vi "COD主界面（列队使用）.vi"() -> (8 "多列列表框":i32(listbox))   [LabVIEW 2016, in "斯坦道CODMn.lvlib"]
uses:
  <vilib>/Analysis/6fits.llb/Curve Fitting Criteria.ctl
  <vilib>/Utility/miscctls.llb/LVPointTypeDef.ctl
  <vilib>/Utility/config.llb/Read Key (I32).vi
  <vilib>/Utility/config.llb/Read Key (Double).vi
  <vilib>/Utility/config.llb/Read Key (Boolean).vi
  <vilib>/Utility/config.llb/Write Key (Double).vi
  <vilib>/Utility/config.llb/Write Key (Boolean).vi
  <vilib>/Utility/config.llb/Write Key (I32).vi
  <vilib>/Waveform/WDTFileIO.llb/Read Waveform from File.vi
  <vilib>/ptbypt/NI_PtbyPt.lvlib
  <vilib>/Utility/config.llb/NI_LVConfig.lvlib
  <vilib>/Analysis/NI_AALPro.lvlib
panel:
  in  "标样核查量程选择":enum32{"H", "L", "AUTO"}(ring)=enum."AUTO"
  in  "标样浓度":dbl
  in  "零点核查量程选择":enum32{"H", "L", "AUTO"}(ring)=enum."AUTO"
  in  "零点核查浓度":dbl
  out "序列号":string
  in  "采水泵排液时间/s:":i32
  in  "采水泵润洗时间/s:":i32
  in  "采水泵沉淀时间/s:":i32
  in  "采水泵进样时间/s:":i32
  in  "常规版/认证版":enum16{"常规版", "认证版", "浮台版"}(ring)
  in  "释放串口":bool
  in  "打开串口":bool
  in  "保存参数":dbl[](array[numeric])
  out "报警数字":i16
  out "CODMn工作状态":T1(ring)
  out "ORP-K":string
  out "ORP-B":string
  out "ORP-A":string
  out "x = y?":bool
  out "稀释倍数解释":string
  in  "跨度量程选择":enum32{"H", "L", "AUTO"}(ring)=enum."AUTO"
  in  "跨度液浓度":dbl
  in  "水样":dbl
  in  "蒸馏水":dbl
  in  "标液":dbl
  in  "质控样":dbl
  in  "加标回收":dbl
  in  "草酸钠":dbl
  in  "高锰酸钾":dbl
  in  "硫酸":dbl
  out "量程解释说明":string
  in  "高切低阈值:":dbl
  in  "低切高阈值:":dbl
  in  "自动切换量程:":enum16{"关闭", "自动切换测一次", "自动切换测两次"}(ring)
  in  "修正系数":dbl
  in  "标准液浓度":dbl
  in  "温度":dbl
  in  "恒温时间":dbl
  in  "基本量程":enum16{"L", "H"}(ring)
  in  "CODMn零点核查选择":enum16{"零点核查走纯水管", "零点核查走质控管"}(ring)
  in  "锁定按钮":bool
  in  "低量程稀释倍数:":i8=1
  out "切换量程连续测两次":bool
  in  "高量程稀释倍数:":i8=2
  in  "一键写入":bool
  in  "测量模式(公式)":u16(ring)=1 items=["水样测试"=1, "标样核查"=2, "零点核查"=3, "跨度核查"=4, "空白测试"=5, "平行样"=6, "加标回收"=7]
  out "基本量程(显示)":string
  out "测量模式(显示)":string
  in  "量程切换次数":u8
  out "数据时间":string
  out "断电排液标记":bool
  out "COM":string
  in  "启用5":bool
  in  "校准5":bool
  in  "泵滴定数5":dbl
  in  "浓度5":dbl
  in  "启用4":bool
  in  "校准4":bool
  in  "泵滴定数4":dbl
  in  "浓度4":dbl
  out "波形时间":timestamp
  in  "历史波形":bool
  out "滴定数-ORP值":u16[](array[numeric]) caption="数组"
  in  "关闭 3":bool
  in  "滴定曲线":bool
  out "ORP滴定曲线":u16[](graph)
  out "空白测试标记":bool
  out "跨度核查标记":bool
  out "启动选择 2":u16(ring) items=["水样测试", "标样核查", "零点核查", "跨度核查", "空白测试", "加标回收", "平行样", "校零", "校标"]
  in  "量程选择":enum16{"低量程", "高量程", "0-2量程"}(ring)
  in  "手动控制":bool
  in  "选用水样":enum16{"葡萄糖", "草酸钠"}(ring)
  in  "方程系数":cluster{"K":dbl, "b":dbl, "X^2":dbl} {"X^2" format="%#.6g"; "b" format="%#.6g"; "K" format="%#.6g"}
  out "多项式系数":dbl[](array[numeric])
  out "XY图":cluster{"X Values":dbl[], "Y Values":dbl[]}[](graph)
  in  "模型":enum32{"线性", "多项式"}(ring)
  out "启动时间":timestamp format="%<%Y/%m/%d %H:%M:%S>T"
  in  "关闭 2":bool
  out "r^2":dbl format="%.8g"
  out "拟合公式":string
  out "b":dbl format="%#.4g"
  out "K":dbl format="%#.4f"
  out "当前校准":i32
  in  "启用3":bool
  in  "启用2":bool
  in  "启用1":bool
  in  "校准3":bool
  in  "校准2":bool
  in  "校准1":bool
  in  "泵滴定数3":dbl
  in  "泵滴定数2":dbl
  in  "泵滴定数1":dbl
  in  "浓度3":dbl
  in  "浓度2":dbl
  in  "浓度1":dbl
  in  "写入":bool
  out "测量模式数字":i32
  out "零点核查标记":bool
  out "排液故障":bool
  out "进水样超量程":bool
  out "标样核查标记":bool
  out "平行样测量":bool
  out "加标回收测量":bool
  out "质控样测量":bool
  out "待机":bool
  out "校标错误":bool
  out "校零错误":bool
  out "测量错误":bool
  out "草酸钠报警":bool
  out "高锰酸钾报警":bool
  out "加热故障":bool
  out "温控器故障":bool
  out "ORP故障":bool
  out "排液标记":bool
  out "故障标记":bool
  out "校标标记":bool
  out "校零标记":bool
  out "通讯状态":bool
  out "水样测量":bool
  in  "读取":bool
  in  "返回":bool
  in  "校准配置":bool
  in  "零点泵计量数 2":dbl
  in  "标度泵计量数 2":dbl
  out "标度滴定值":dbl
  out "零点滴定值":dbl
  in  "保存":bool
  in  "关闭":bool
  out "测量数据区":T2 {"单位" items=["ug/L", "mg/L", "ppm", "mg/m3", "cm", "ppb", "ug/m3", "%", "nmol/mol", "umol/mol", "MPN/L", "MPN/100ml", "ng/m3", "NTU", "无量纲", "ms/cm", "us/cm", "℃", "mV", "万个/L"]}
  out "仪器时间":timestamp format="%<%Y/%m/%d %H:%M:%S>T"
  out "秒":u16
  out "分":u16
  out "COD浓度（mg/L)":dbl format="%.2g"
  out "进样管":dbl
  out "高锰酸钾":dbl
  out "草酸钠":dbl
  out "硫酸":dbl
  out "ORP显示":dbl
  out "温度":dbl
  out "加热":bool
  out "搅拌":bool
  out "进硫酸":bool
  out "进加标回收样":bool
  out "进质控样":bool
  out "进标液":bool
  out "进蒸馏水":bool
  out "进水样":bool
  out "进草酸钠":bool
  out "进高锰酸钾":bool
  out "定时启动":bool
  in  "启动":bool
  in  "故障清除":bool
  in  "参数配置":bool
  in  "停止":bool
  in  "单步启动":bool
  out "系统时间":timestamp
  in  "时间校准":bool
  out "报警簇":T3
  out "模式（受控）":u16
  # "测量时间："
  # "(水样~加标回收)"
  # "mV"
  # "℃"
  # "注：遇到加热故障和排液故障时仪器不能正常启动，\n必须排查故障并点击报警清除按钮方可运行。"
  # "mg/L"
  # "基本参数设置"
  # "校零校标结果"
  # "泵计量参数设置"
  # "校零结果："
  # "校零滴定值："
  # "加热恒温温度(℃):"
  # "水样："
  # "高锰酸钾："
  # "校标结果："
  # "标度滴定值："
  # "恒温时间(分钟):"
  # "草酸钠："
  # "蒸馏水："
  # "零点泵计量值："
  # "标准液浓度(mg/L):"
  # "硫酸："
  # "标液："
  # "标度泵计量值："
  # "修正系数："
  # "跨度核查浓度："
  # "质控样:"
  # "基本量程(L、H)可选:"
  # "跨度量程选择："
  # "加标回收样："
  # "零点核查浓度："
  # "标样浓度："
  # "零点量程选择："
  # "标样量程选择："
  # "是否启用"
  # "泵滴定数"
  # "浓度"
  # "辅\n助\n计\n算\n区"
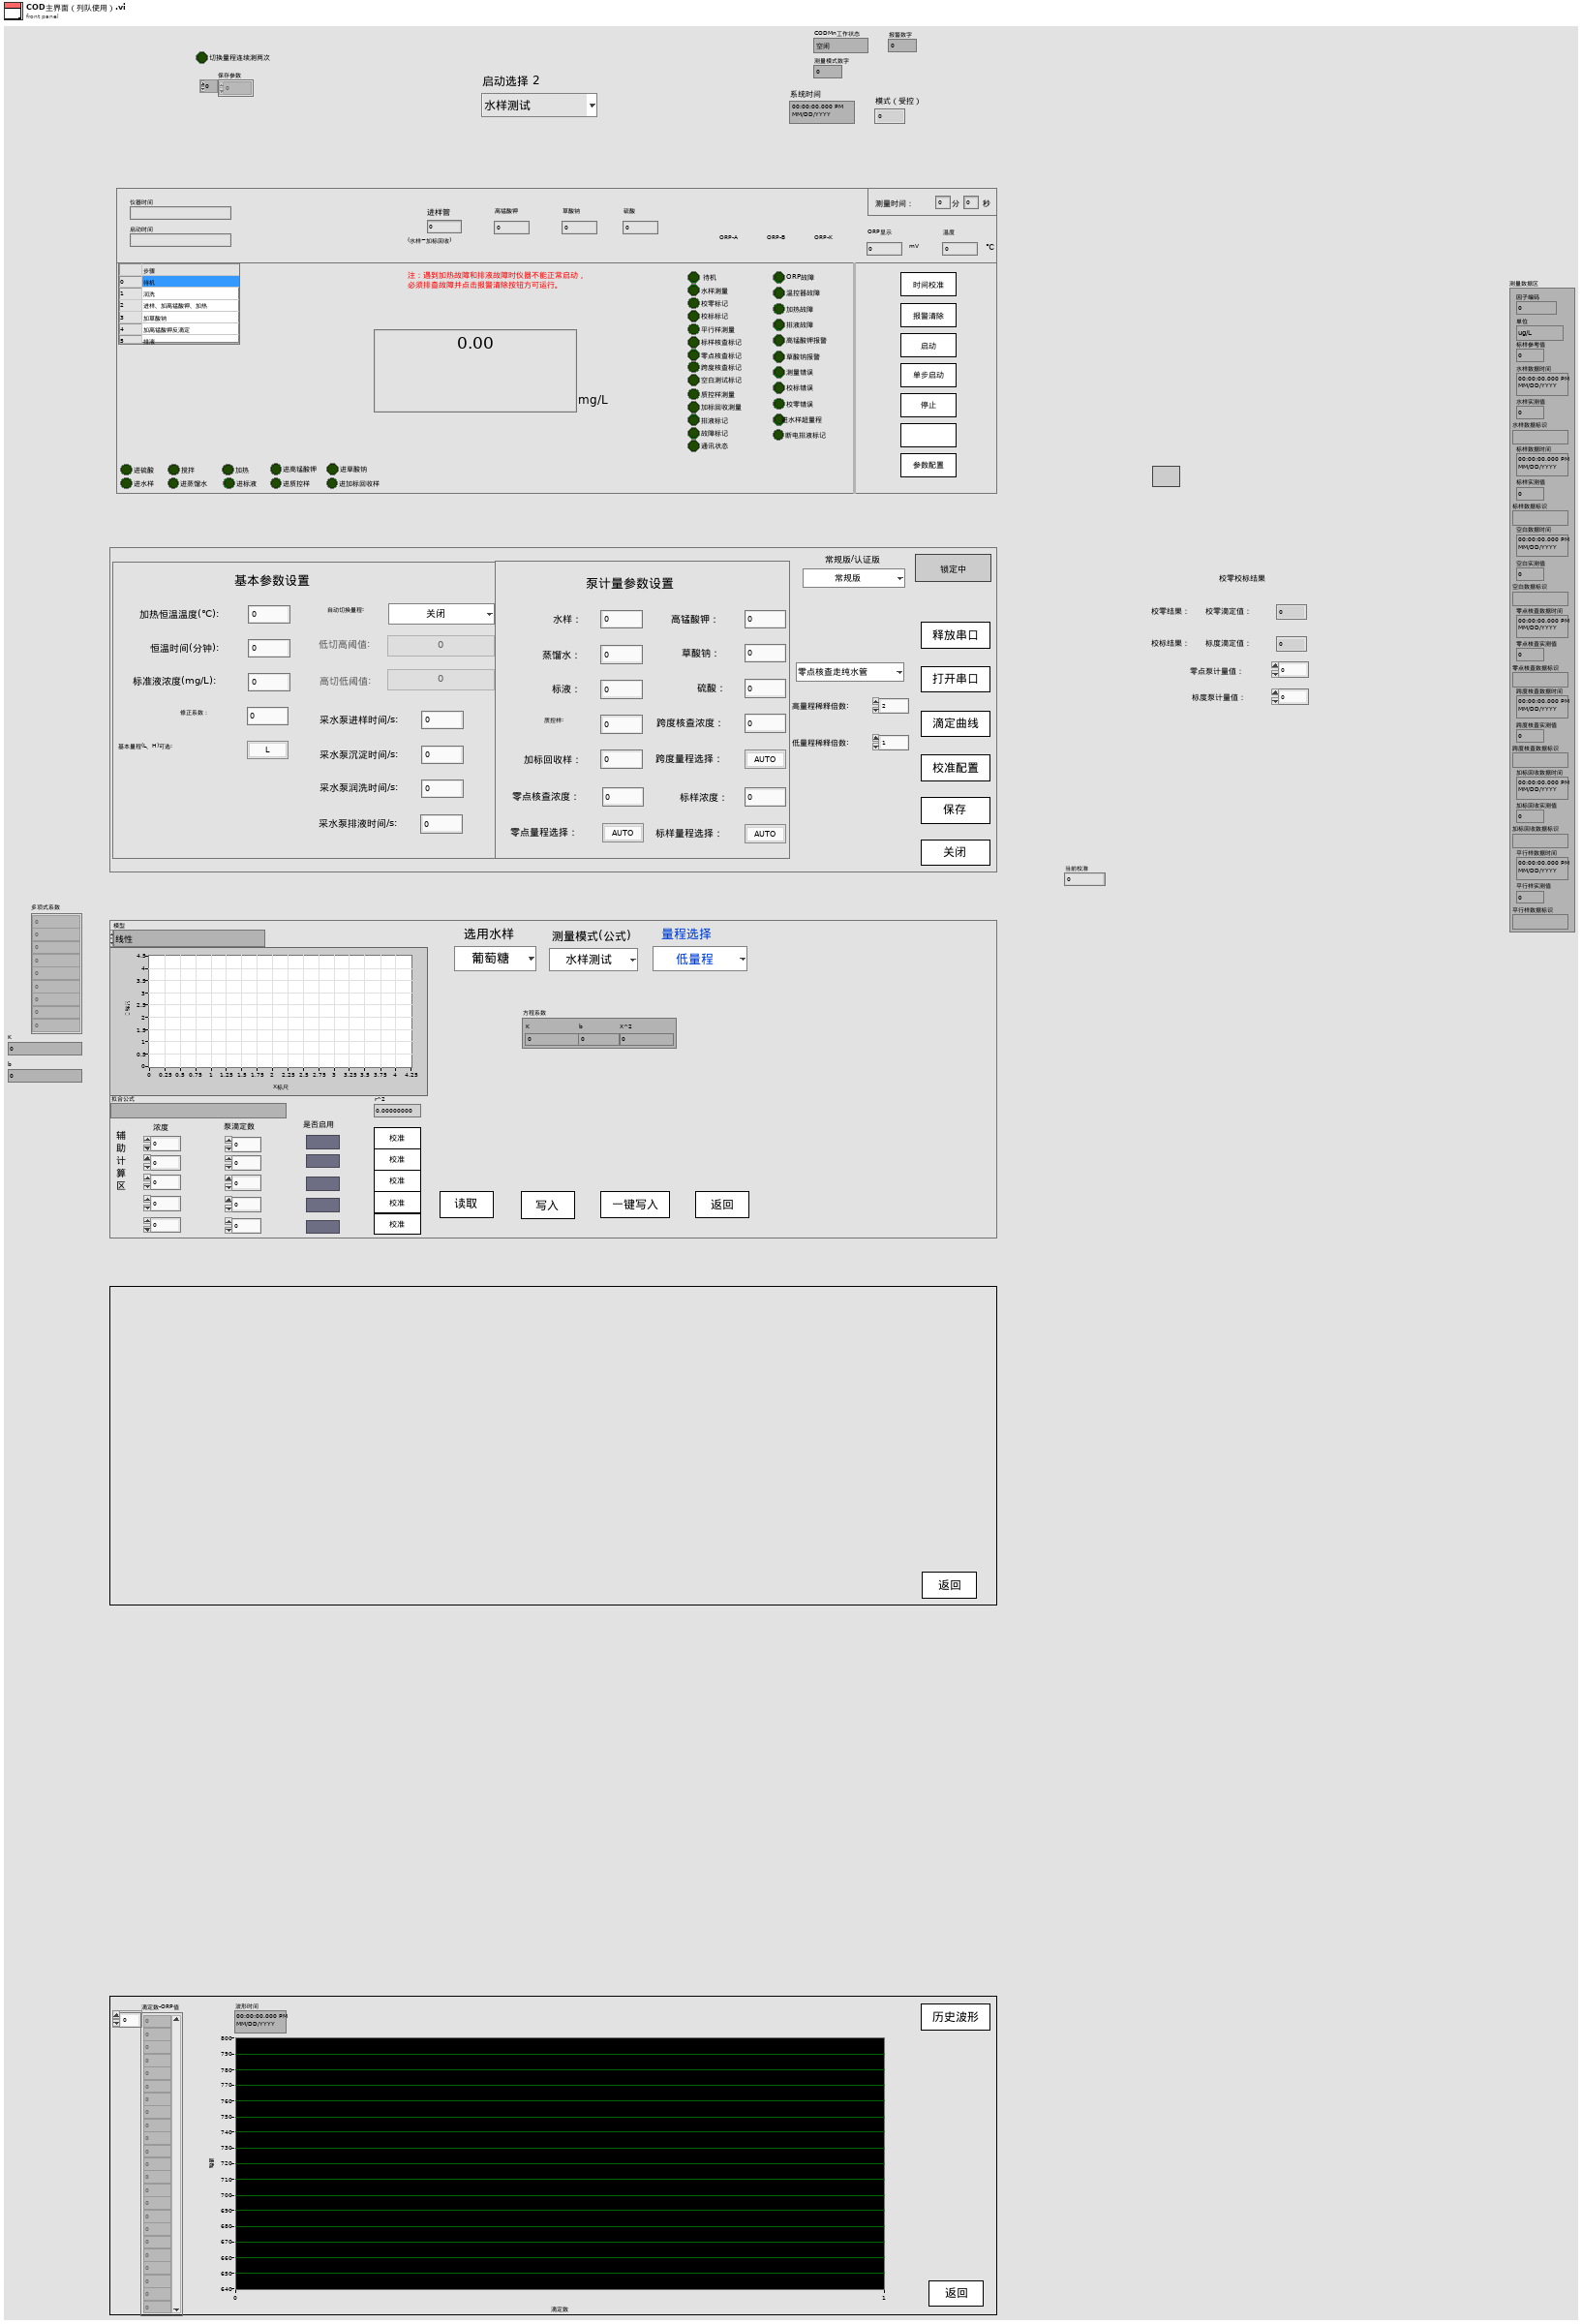
[diagram p1: front panel]
types:
  T1 = enum16{"空闲", "水样测试", "标样核查", "零点核查", "跨度核查", "空白测试", "平行样测试", "质控样", "空白校准", "标样校准", "加标回收"}
  T2 = cluster{"因子编码":u32, "单位":u16, "标样参考值":sgl, "水样数据时间":timestamp, "水样实测值":sgl, "水样数据标识":string, "标样数据时间":timestamp, "标样实测值":sgl, "标样数据标识":string, "空白数据时间":timestamp, "空白实测值":sgl, "空白数据标识":string, "零点核查数据时间":timestamp, "零点核查实测值":sgl, "零点核查数据标识":string, "跨度核查数据时间":timestamp, "跨度核查实测值":sgl, "跨度核查数据标识":string, "加标回收数据时间":timestamp, "加标回收实测值":sgl, "加标回收数据标识":string, "平行样数据时间":timestamp, "平行样实测值":sgl, "平行样数据标识":string}
  T3 = cluster{"ORP故障":bool, "温控器故障":bool, "加热故障":bool, "高锰酸钾报警":bool, "草酸钠报警":bool, "测量错误":bool, "校零错误":bool, "校标错误":bool, " 进水样超量程":bool, "排液阀故障":bool}
  T4 = cluster{"命令":string, "测量模式":enum16{"水样测量", "标样核查", "零点核查", "跨度核查", "空白测试", "加标回收", "平行样", "校零", "校标"}, "CODMn量程切换":enum32{"H", "L", "AUTO"}}
  T5 = cluster{"时间":timestamp, "测量模式":string, "数据类型":string, "检测值":sgl, "单位":string, "数据标识":string, "因子编码":string, "标样参考值":sgl, "ORP-A":sgl, "ORP-B":sgl, "ORP-K":sgl, "COD滴定值":sgl, "高锰酸钾滴定数":sgl, "温度":sgl, "序列号":string, "量程":sgl, "LastTime":timestamp}
  T6 = enum8{"Enabled", "Disabled", "Disabled and Grayed Out"}
  T7 = cluster{"数组 2[0]":sgl, "数组 2[1]":sgl, "数组 2[2]":sgl, "数组 2[3]":sgl, "数组 2[4]":sgl, "数组 2[5]":sgl, "数组 2[6]":sgl, "数组 2[7]":sgl, "数组 2[8]":sgl, "数组 2[9]":sgl, "数组 2[10]":sgl, "数组 2[11]":sgl, "数组 2[12]":sgl, "数组 2[13]":sgl, "数组 2[14]":sgl, "数组 2[15]":sgl, "数组 2[16]":sgl, "数组 2[17]":sgl, "数组 2[18]":sgl, "数组 2[19]":sgl, "数组 2[20]":sgl, "数组 2[21]":sgl, "数组 2[22]":sgl, "数组 2[23]":sgl, "数组 2[24]":sgl, "数组 2[25]":sgl, "数组 2[26]":sgl, "数组 2[27]":sgl, "数组 2[28]":sgl, "数组 2[29]":sgl, "数组 2[30]":sgl, "数组 2[31]":sgl, "数组 2[32]":sgl, "数组 2[33]":sgl, "数组 2[34]":sgl, "数组 2[35]":sgl, "数组 2[36]":sgl, "数组 2[37]":sgl, "数组 2[38]":sgl, "数组 2[39]":sgl, "数组 2[40]":sgl, "数组 2[41]":sgl}
  T8 = typedef "NI_AALPro.lvlib/Curve Fitting Criteria.ctl" = u16
  T9 = cluster{"测量模式":enum16{"水样测量", "标样核查", "零点核查", "跨度核查", "空白测试", "加标回收", "平行样", "校零", "校标"}}
  T10 = cluster{"仪器测试类型":enum16{"水样测试", "零点核查", "标样核查", "空白测试", "跨度核查", "加标回收", "平行样", "校零", "校标"}, "周期设置类型":enum16{"定点启动", "间隔启动"}, "定时功能启用":bool, "定时间隔":dbl, "24H周期设置":bool[]}
  T11 = typedef "LVDateTimeRec.ctl" = cluster{"秒数的小数部分":dbl, "秒":i32, "分":i32, "时":i32, "日":i32, "月":i32, "年":i32, "天数（周）":i32, "天数（年）":i32, "DST":i32}
  T12 = enum16{"水样测试", "零点核查", "标样核查", "空白测试", "跨度核查", "加标回收", "平行样", "校零", "校标"}
  T13 = cluster{"时间标识":timestamp, "设备":string, "日志信息":string}
  T14 = cluster{"时间标识":timestamp, "参数":string, "日志信息":string, "流程参数":string}
  T15 = cluster{"时间标识":timestamp, "设备":string, "日志信息":string, "流程参数":string}
  T16 = typedef "NI_LVConfig.lvlib/Config Data RefNum.ctl" = refnum<k1>
  T17 = typedef "LVPointTypeDef.ctl" = cluster{"Horizontal":i16, "Vertical":i16}
  T18 = enum16{"水样测量", "标样核查", "零点核查", "跨度核查", "空白测试", "加标回收", "平行样", "校零", "校标"}
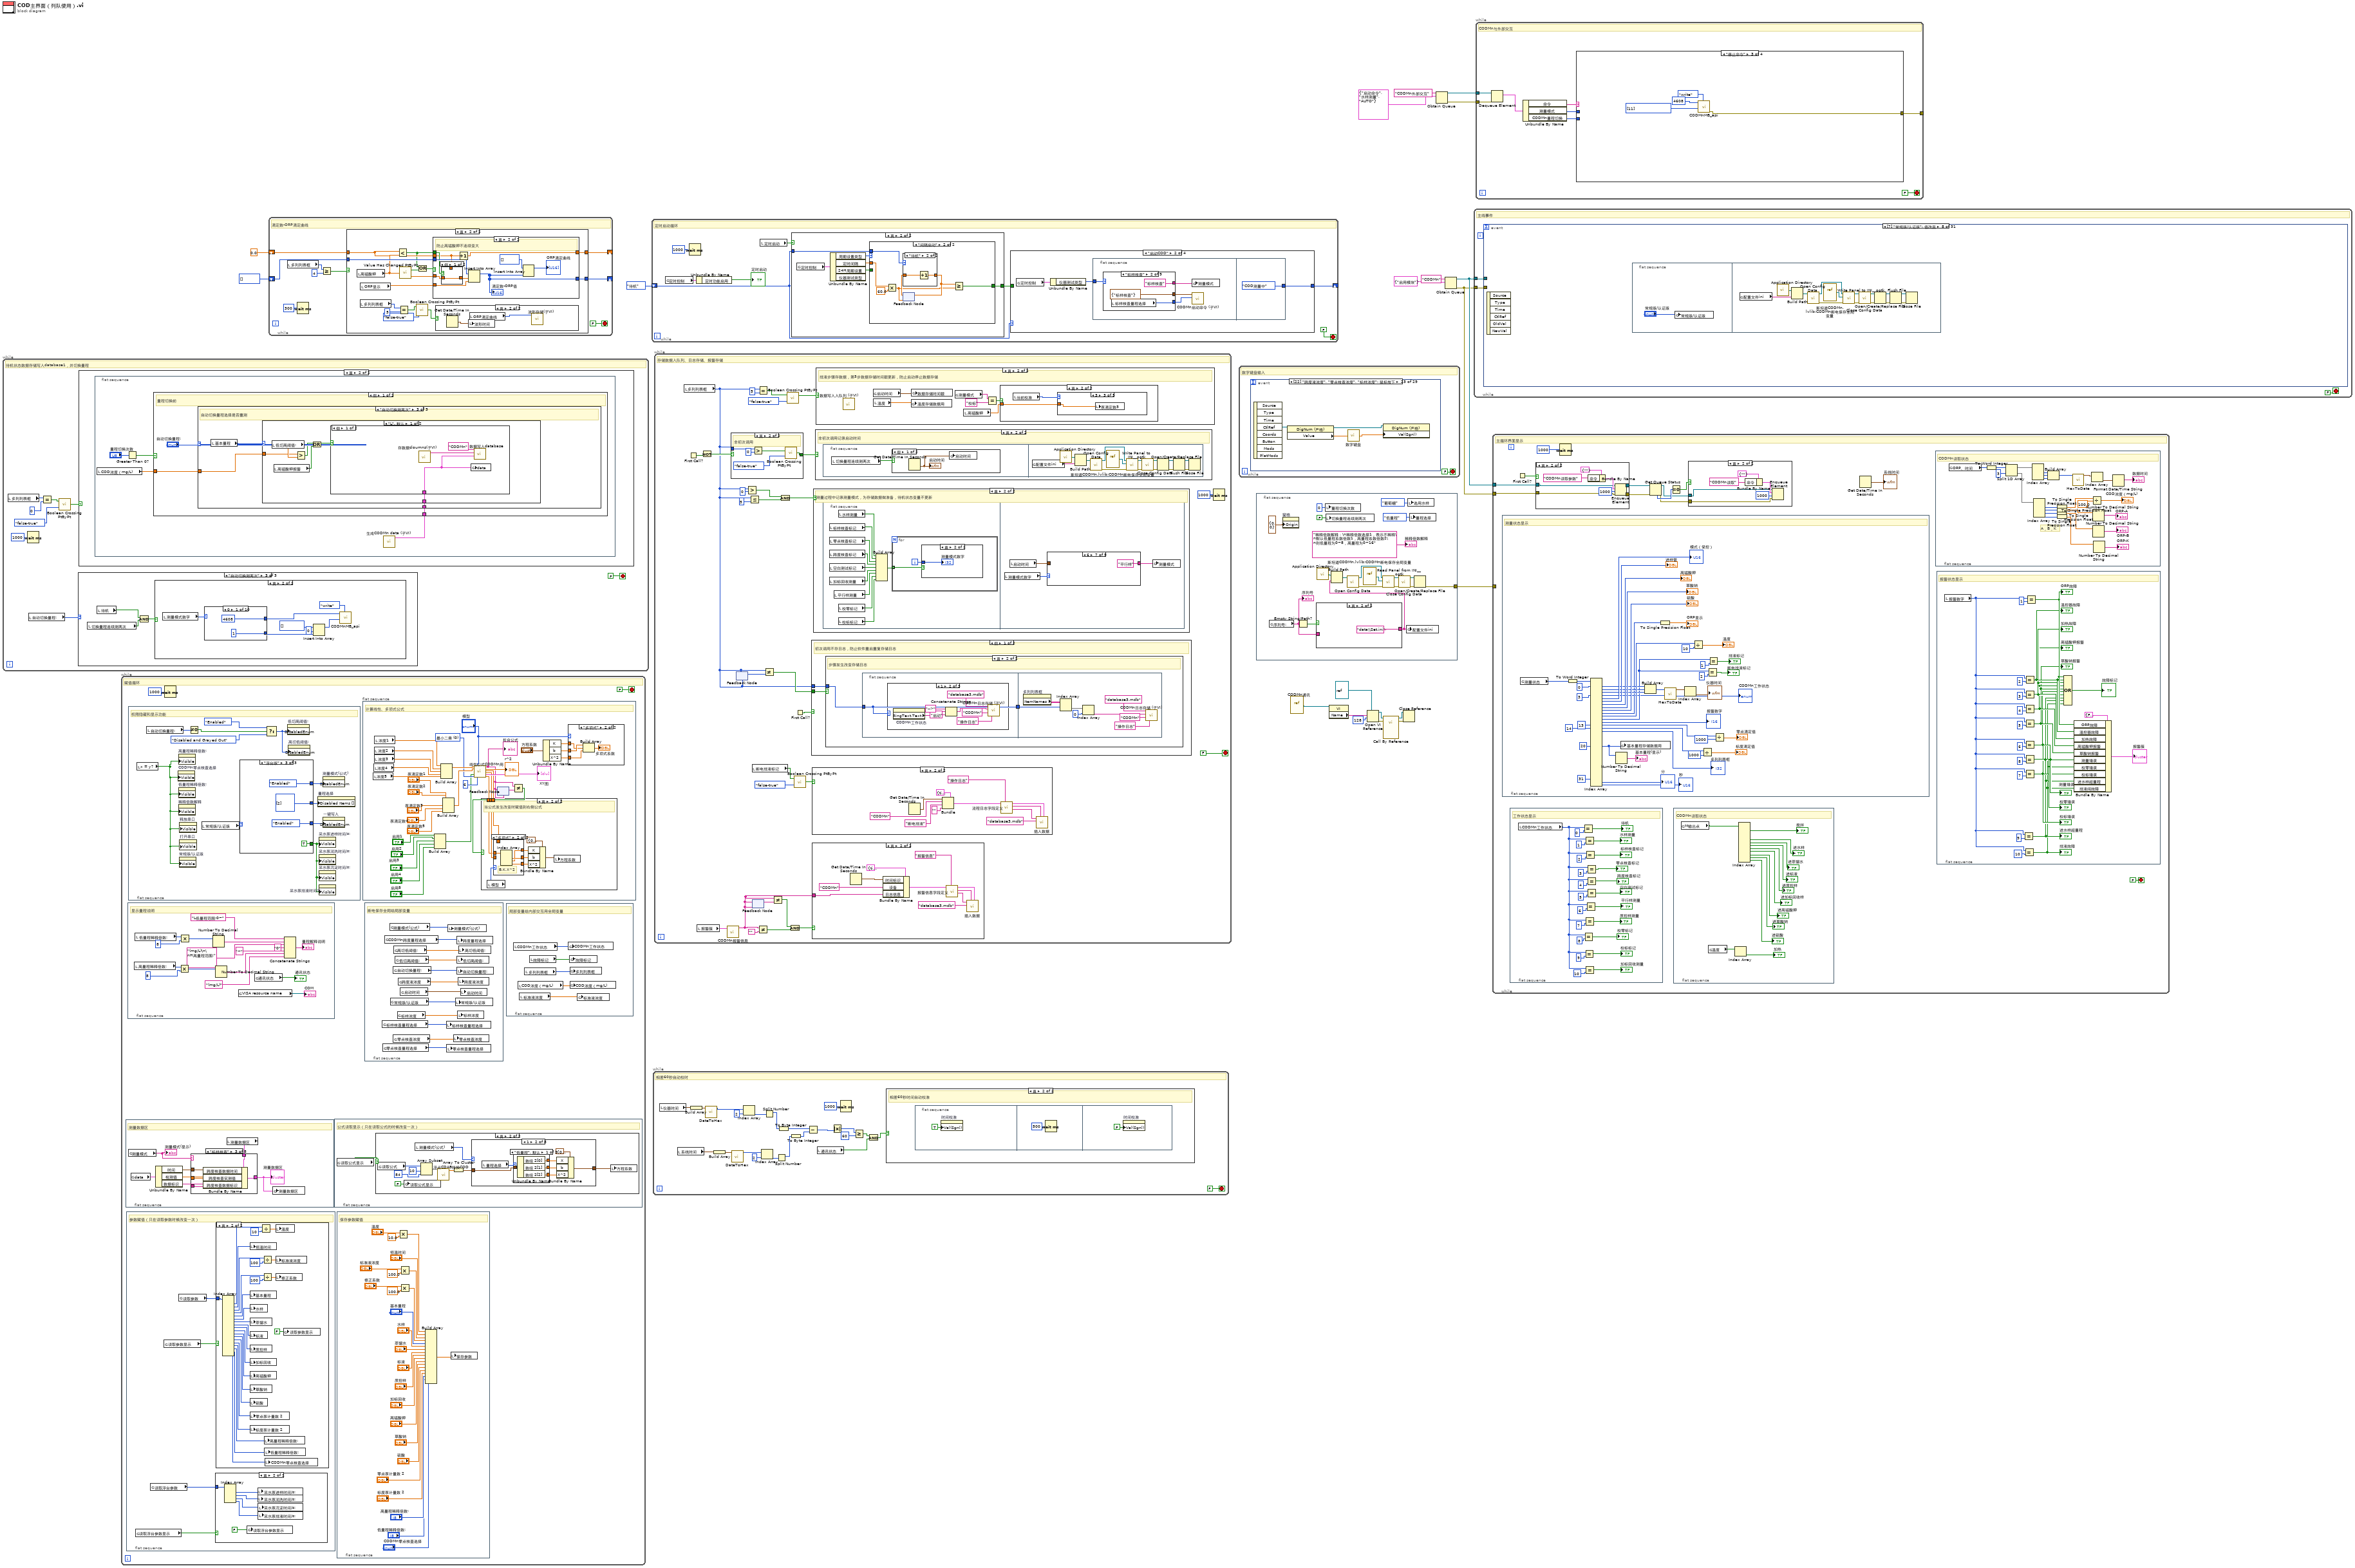
[diagram p0: block diagram]
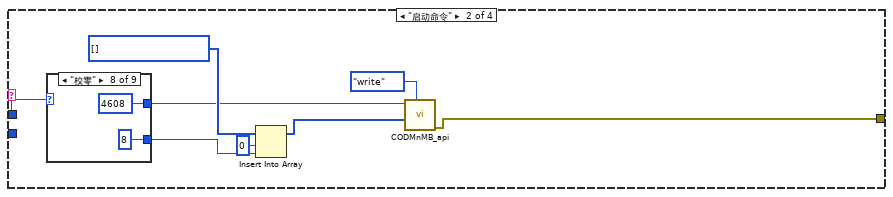
[diagram p3: hidden frame]
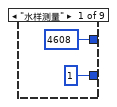
[diagram p4: hidden frame]
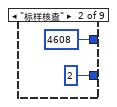
[diagram p5: hidden frame]
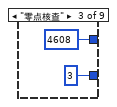
[diagram p6: hidden frame]
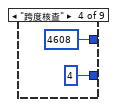
[diagram p7: hidden frame]
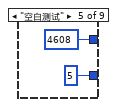
[diagram p8: hidden frame]
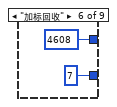
[diagram p9: hidden frame]
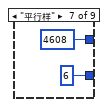
[diagram p10: hidden frame]
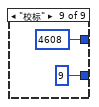
[diagram p11: hidden frame]
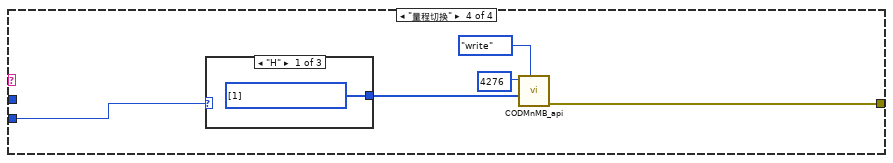
[diagram p12: hidden frame]
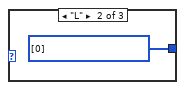
[diagram p13: hidden frame]
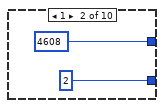
[diagram p19: hidden frame]
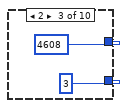
[diagram p20: hidden frame]
diagram:
  n1 = while {
    stop <- FALSE stop-if-true
    # "待机状态数据存储写入database1，并切换量程"
    n2 = local read "多列列表框"() -> (w26:i32)
    n3 = Wait (ms)(milliseconds to wait=u32 1000 ("等待时间（毫秒）")) -> ()  [unwired: 1 out]
    n4 = local read "自动切换量程:"() -> (w21:enum16{"关闭", "自动切换测一次", "自动切换测两次"})
    n5 = Equal?(x=w26, y=0) -> (x = y?=w24:bool)
    n6 = call <vilib>:"Boolean Crossing PtByPt.vi"("direction"=enum16{"either", "false-true", "true-false"}."false-true", "input"=w24) -> ("crossing"=w22:bool)  [unwired: 1 in]
    n7 = case shown="\"自动切换测两次\"" w21 {
      frame "关闭", Default {
      }
      frame "自动切换测一次" {
      }
      frame "自动切换测两次" {
        n8 = local read "切换量程连续测两次"() -> (w30:bool)
        n9 = local read "待机"() -> (w31:bool)
        n10 = Compound Arithmetic op=AND ("复合运算")(w31, w30) -> (w29:bool)
        n11 = case shown="真" w29 {
          frame False {
          }
          frame True {
            n12 = local read "测量模式数字"() -> (w35:i32)
            n13 = case shown="0" w35 {
              tunnel: [u16 4608 ("address") u16 4608 ("address") u16 4608 ("address") u16 4608 ("address") u16 4608 ("address") u16 4608 ("address") u16 4608 ("address") u16 4608 ("address") u16 4608 ("address") u16 4608 ("address")] -> w32
              tunnel: [u16 1 ("address") u16 2 ("address") u16 3 ("address") u16 4 ("address") u16 5 ("address") u16 7 ("address") u16 6 ("address") u16 8 ("address") u16 9 ("address") u16 0 ("address")] -> w38
              frame 0 {
              }
              frame 1 {
              }
              frame 2 {
              }
              frame 3 {
              }
              frame 4 {
              }
              frame 5 {
              }
              frame 6 {
              }
              frame 7 {
              }
              frame 8 {
              }
              frame 9, Default {
              }
            }
            n14 = Insert Into Array(array=u16[] [] ("values"), index=0 ("索引"), new element=w38) -> (w33:u16[])
            n15 = call "CODMnMB_api.vi"("STEP"=enum16{"open", "read", "write", "close"}."write", "values"=w33, "starting address"=w32) -> ()  [unwired: 5 in, 4 out]
          }
        }
      }
    }
    n16 = case shown="真" w22 {
      frame False {
      }
      frame True {
        n17 = flat-sequence {
          frame #0 {
            n18 = local read "COD浓度（mg/L)"() -> (w59:dbl)
            n19 = Greater Than 0?(x="量程切换次数") -> (x > 0?=w60:bool)
            n20 = call "生成CODMn data (子VI).vi"() -> ("data"=w62:T5)  [unwired: 11 in]
            n21 = case shown="假" w60 {
              tunnel: w62 -> [w64 w121]
              tunnel: w59 -> [w63 _]
              frame False {
                # "量程切换前"
                n22 = case shown="\"自动切换测两次\"" "自动切换量程:" {
                  tunnel: w64 -> [w66 w71 w95]
                  tunnel: w63 -> [_ w70 w94]
                  frame "关闭", Default {
                    # "关闭自动切换量程"
                    n23 = call "存数据cloumns(子VI).vi"() -> ("数组"=w68:string[])  [unwired: 11 in]
                    n24 = global write "COD读取DATA全局.vi" "data"(w66) -> ()
                    n25 = call "数据写入database.vi"("data"=w66, "columns"=w68, "table"="CODMn") -> ()  [unwired: 8 in, 1 out]
                  }
                  frame "自动切换测一次" {
                    # "自动切换量程选择是否重测"
                    n26 = global read "COD测量模式全局.vi" "测量模式"() -> (w77:string)
                    n27 = Not Equal?(x=w77, y="水样测试") -> (x != y?=w75:bool)
                    n28 = case shown="假" w75 {
                      tunnel: [w78 w79] -> w74
                      tunnel: w70 -> [w78 _]
                      frame False {
                      }
                      frame True {
                        n29 = global read "COD读取DATA全局.vi" "测量数据区"() -> (w80:T2)
                        n30 = Unbundle By Name(w80) -> ("水样实测值"=w79:sgl)
                      }
                    }
                    n31 = local read "基本量程"() -> (w69:enum16{"L", "H"})
                    n32 = case shown="\"H\"" w69 {
                      tunnel: w74 -> [w81 w87]
                      frame "L", Default {
                        n33 = Greater?(x=w81, y="低切高阈值:") -> (0:w82:bool)
                        n34 = case shown="假" w82 {
                          frame False {
                          }
                          frame True {
                            n35 = call "CODMnMB_api.vi"("STEP"=enum16{"open", "read", "write", "close"}."write", "values"=u16[] [1], "starting address"=u16 4276) -> ()  [unwired: 5 in, 4 out]
                          }
                        }
                      }
                      frame "H" {
                        n36 = Less?(x=w87, y="高切低阈值:") -> (x < y?=w88:bool)
                        n37 = case shown="真" w88 {
                          frame False {
                          }
                          frame True {
                            n38 = call "CODMnMB_api.vi"("STEP"=enum16{"open", "read", "write", "close"}."write", "values"=u16[] [0], "starting address"=u16 4276) -> ()  [unwired: 5 in, 4 out]
                          }
                        }
                      }
                    }
                    n39 = call "存数据cloumns(子VI).vi"() -> ("数组"=w73:string[])  [unwired: 11 in]
                    n40 = global write "COD读取DATA全局.vi" "data"(w71) -> ()
                    n41 = call "数据写入database.vi"("data"=w71, "columns"=w73, "table"="CODMn") -> ()  [unwired: 8 in, 1 out]
                  }
                  frame "自动切换测两次" {
                    # "自动切换量程选择是否重测"
                    n42 = local read "基本量程"() -> (w93:enum16{"L", "H"})
                    n43 = case shown="\"L\", 默认" w93 {
                      tunnel: w94 -> [w99 w110]
                      tunnel: w95 -> [w98 w109]
                      frame "L", Default {
                        n44 = local read "低切高阈值:"() -> (w100:dbl)
                        n45 = local read "高锰酸钾报警"() -> (w96:bool)
                        n46 = Greater?(x=w99, y=w100) -> (0:w101:bool)
                        n47 = Or(x=w101, y=w96) -> (x .or. y?=w97:bool)
                        n48 = case shown="假" w97 {
                          tunnel: w98 -> [w102 _]
                          frame False {
                            n49 = call "存数据cloumns(子VI).vi"() -> ("数组"=w104:string[])  [unwired: 11 in]
                            n50 = global write "COD读取DATA全局.vi" "data"(w102) -> ()
                            n51 = call "数据写入database.vi"("data"=w102, "columns"=w104, "table"="CODMn") -> ()  [unwired: 8 in, 1 out]
                          }
                          frame True {
                            n52 = call "CODMnMB_api.vi"("STEP"=enum16{"open", "read", "write", "close"}."write", "values"=u16[] [1], "starting address"=u16 4276) -> ()  [unwired: 5 in, 4 out]
                            "切换量程连续测两次" <- TRUE ("切换量程连续测两次")
                          }
                        }
                      }
                      frame "H" {
                        n53 = local read "高切低阈值:"() -> (w111:dbl)
                        n54 = Less?(x=w110, y=w111) -> (x < y?=w112:bool)
                        n55 = case shown="真" w112 {
                          tunnel: w109 -> [w113 _]
                          frame False {
                            n56 = call "存数据cloumns(子VI).vi"() -> ("数组"=w115:string[])  [unwired: 11 in]
                            n57 = global write "COD读取DATA全局.vi" "data"(w113) -> ()
                            n58 = call "数据写入database.vi"("data"=w113, "columns"=w115, "table"="CODMn") -> ()  [unwired: 8 in, 1 out]
                          }
                          frame True {
                            # "重测第一次不存数据"
                            n59 = call "CODMnMB_api.vi"("STEP"=enum16{"open", "read", "write", "close"}."write", "values"=u16[] [0], "starting address"=u16 4276) -> ()  [unwired: 5 in, 4 out]
                            n60 = local write "切换量程连续测两次"(TRUE ("切换量程连续测两次")) -> ()
                          }
                        }
                      }
                    }
                  }
                }
              }
              frame True {
                # "防止无限切量程"
                n61 = local write "量程切换次数"(u8 0 ("量程切换次数")) -> ()
                n62 = call "存数据cloumns(子VI).vi"() -> ("数组"=w123:string[])  [unwired: 11 in]
                n63 = call "数据写入database.vi"("data"=w121, "columns"=w123, "table"="CODMn") -> ()  [unwired: 8 in, 1 out]
                n64 = global write "COD读取DATA全局.vi" "data"(w121) -> ()
              }
            }
          }
        }
      }
    }
  }
  n65 = while {
    stop <- FALSE stop-if-true
    # "赋值循环"
    n66 = flat-sequence {
      frame #0 {
        # "测量数据区"
        n67 = global read "COD测量模式全局.vi" "测量模式"() -> (w391:string)
        "测量模式(显示)" <- w391
        n68 = global read "COD读取DATA全局.vi" "data"() -> (w396:T5)
        n69 = Unbundle By Name(w396) -> ("时间"=w395:timestamp, "检测值"=w394:sgl, "数据标识"=w393:string)
        n70 = local read "测量数据区"() -> (w397:T2)
        n71 = case shown="\"标样核查\"" w391 {
          tunnel: w397 -> [w398 w403 w408 w413 w418 w423 w428 w433]
          tunnel: [w398 w402 w404 w412 w417 w422 w424 w432] -> w392
          tunnel: w395 -> [_ w401 w407 w411 w416 w421 w427 w431]
          tunnel: w394 -> [_ w400 w406 w410 w415 w420 w426 w430]
          tunnel: w393 -> [_ w399 w405 w409 w414 w419 w425 w429]
          frame "", Default {
          }
          frame "水样测试" {
            n72 = Bundle By Name(cluster=w403, "水样数据时间"=w401, "水样实测值"=w400, "水样数据标识"=w399) -> (w402:T2)
          }
          frame "标样核查" {
            n73 = Bundle By Name(cluster=w408, "跨度核查数据时间"=w407, "跨度核查实测值"=w406, "跨度核查数据标识"=w405) -> (w404:T2)
          }
          frame "零点核查" {
            n74 = Bundle By Name(cluster=w413, "零点核查数据时间"=w411, "零点核查实测值"=w410, "零点核查数据标识"=w409) -> (w412:T2)
          }
          frame "加标回收" {
            n75 = Bundle By Name(cluster=w418, "加标回收数据时间"=w416, "加标回收实测值"=w415, "加标回收数据标识"=w414) -> (w417:T2)
          }
          frame "平行样" {
            n76 = Bundle By Name(cluster=w423, "平行样数据时间"=w421, "平行样实测值"=w420, "平行样数据标识"=w419) -> (w422:T2)
          }
          frame "校零" {
            n77 = Bundle By Name(cluster=w428, "空白数据时间"=w427, "空白实测值"=w426, "空白数据标识"=w425) -> (w424:T2)
          }
          frame "校标" {
            n78 = Bundle By Name(cluster=w433, "标样数据时间"=w431, "标样实测值"=w430, "标样数据标识"=w429) -> (w432:T2)
          }
        }
        "测量数据区" <- w392
        n79 = global write "COD读取DATA全局.vi" "测量数据区"(w392) -> ()
      }
    }
    n80 = flat-sequence {
      frame #0 {
        # "参数赋值（只在读取参数时候改变一次）"
        n81 = global read "COD读取DATA全局.vi" "读取浮台参数显示"() -> (w157:bool)
        n82 = global read "COD读取DATA全局.vi" "读取浮台参数"() -> (w156:u16[])
        n83 = global read "COD读取DATA全局.vi" "读取参数显示"() -> (w158:bool)
        n84 = global read "COD读取DATA全局.vi" "读取参数"() -> (w159:u16[])
        n85 = case shown="真" w157 {
          tunnel: w156 -> [_ w165]
          frame False {
          }
          frame True {
            n86 = Index Array(array=w165) -> (element #1=w164:u16, element #2=w163:u16, element #3=w162:u16, element #4=w161:u16)  [unwired: 4 in]
            n87 = global write "COD读取DATA全局.vi" "读取浮台参数显示"(FALSE ("读取参数显示")) -> ()
            n88 = local write "采水泵进样时间/s:"(w164) -> ()
            n89 = local write "采水泵润洗时间/s:"(w163) -> ()
            n90 = local write "采水泵沉淀时间/s:"(w162) -> ()
            n91 = local write "采水泵排液时间/s:"(w161) -> ()
          }
        }
        n92 = case shown="真" w158 {
          tunnel: w159 -> [_ w167]
          frame False {
          }
          frame True {
            n93 = Index Array(array=w167) -> (element #1=w179:u16, element #2=w191:u16, element #3=w172:u16, element #4=w177:u16, element #5=w175:u16, element #6=w174:u16, element #7=w190:u16, element #8=w189:u16, element #9=w188:u16, element #10=w187:u16, element #11=w186:u16, element #12=w185:u16, element #13=w184:u16, element #14=w183:u16, element #15=w182:u16, element #16=w170:u16, element #17=w169:u16, element #18=w168:u16)  [unwired: 18 in]
            n94 = local write "恒温时间"(w191) -> ()
            n95 = local write "基本量程"(w175) -> ()
            n96 = local write "水样"(w174) -> ()
            n97 = local write "蒸馏水"(w190) -> ()
            n98 = local write "标液"(w189) -> ()
            n99 = local write "质控样"(w188) -> ()
            n100 = local write "加标回收"(w187) -> ()
            n101 = local write "高锰酸钾"(w186) -> ()
            n102 = local write "草酸钠"(w185) -> ()
            n103 = local write "硫酸"(w184) -> ()
            n104 = local write "零点泵计量数 2"(w183) -> ()
            n105 = local write "标度泵计量数 2"(w182) -> ()
            n106 = Divide(x=w179, y=u16 10) -> (x/y=w180:dbl)
            n107 = Divide(x=w172, y=u16 100) -> (x/y=w171:dbl)
            n108 = Divide(x=w177, y=u16 100) -> (x/y=w176:dbl)
            n109 = local write "高量程稀释倍数:"(w170) -> ()
            n110 = local write "低量程稀释倍数:"(w169) -> ()
            n111 = local write "CODMn零点核查选择"(w168) -> ()
            n112 = local write "温度"(w180) -> ()
            n113 = local write "标准液浓度"(w171) -> ()
            n114 = local write "修正系数"(w176) -> ()
            n115 = global write "COD读取DATA全局.vi" "读取参数显示"(FALSE ("读取参数显示")) -> ()
          }
        }
      }
    }
    n116 = flat-sequence {
      frame #0 {
        # "显示量程说明"
        n117 = local read "高量程稀释倍数:"() -> (w449:i8)
        n118 = local read "低量程稀释倍数:"() -> (w459:i8)
        n119 = Multiply(x=w449, y=i8 8) -> (x*y=w447:i8)
        n120 = Multiply(x=w459, y=i8 8) -> (x*y=w451:i8)
        n121 = Number To Decimal String(number=w451) -> (decimal integer string=w456:string)  [unwired: 1 in]
        n122 = Number To Decimal String(number=w447) -> (decimal integer string=w454:string)  [unwired: 1 in]
        n123 = global read "CODMn断电保存全局变量.vi" "VISA resource name"() -> (→"COM":refnum<visa-resource-name>)
        n124 = global read "COD读取DATA全局.vi" "通讯状态"() -> (→"通讯状态":bool)
        n125 = Concatenate Strings("L低量程范围:0~" ("量程解释说明"), w456, "(mg/L)\n\nH高量程范围:" ("量程解释说明"), "0" ("字符串"), "~" ("量程解释说明"), w454, "(mg/L)" ("量程解释说明")) -> (→"量程解释说明":string)
      }
    }
    n126 = flat-sequence {
      frame #0 {
        # "权限隐藏和显示功能"
        n127 = local read "x = y?"() -> (w462:bool)
        n128 = local read "自动切换量程:"() -> (w469:enum16{"关闭", "自动切换测一次", "自动切换测两次"})
        n129 = property on="CODMn零点核查选择" class="Enum (严格)"("Visible"=w462) -> ()  [unwired: 2 in, 2 out]
        n130 = property on="高量程稀释倍数:" class="DigNum (严格)"("Visible"=w462) -> ()  [unwired: 2 in, 2 out]
        n131 = property on="低量程稀释倍数:" class="DigNum (严格)"("Visible"=w462) -> ()  [unwired: 2 in, 2 out]
        n132 = property on="稀释倍数解释" class="Str"("Visible"=w462) -> ()  [unwired: 2 in, 2 out]
        n133 = property on="常规版/认证版" class="Enum (严格)"("Visible"=w462) -> ()  [unwired: 2 in, 2 out]
        n134 = property on="释放串口" class="Bool"("Visible"=w462) -> ()  [unwired: 2 in, 2 out]
        n135 = property on="打开串口" class="Bool"("Visible"=w462) -> ()  [unwired: 2 in, 2 out]
        n136 = Not Equal To 0?(x=w469) -> (x != 0?=w468:bool)
        n137 = local read "常规版/认证版"() -> (w467:enum16{"常规版", "认证版", "浮台版"})
        n138 = case shown="\"浮台版\"" w467 {
          tunnel: [T6."Enabled" ("禁用") T6."Disabled and Grayed Out" ("禁用") T6."Enabled" ("禁用")] -> w466
          tunnel: [i32[] [2] ("禁用项[]") i32[] [] ("禁用项[]") i32[] [2] ("禁用项[]")] -> w465
          tunnel: [T6."Enabled" ("禁用") T6."Disabled and Grayed Out" ("禁用") T6."Enabled" ("禁用")] -> w464
          tunnel: [FALSE FALSE TRUE] -> w463
          frame "常规版", Default {
          }
          frame "认证版" {
            w478 = u16 1 items=["水样测试"=1, "标样核查"=2, "零点核查"=3, "跨度核查"=4, "空白测试"=5, "平行样"=6, "加标回收"=7] ("测量模式(公式)")
            n139 = global write "CODMn断电保存全局变量.vi" "测量模式(公式)"(w478) -> ()
          }
          frame "浮台版" {
          }
        }
        n140 = Select(t=T6."Enabled" ("禁用"), s=w468, f=T6."Disabled and Grayed Out" ("禁用")) -> (s? t:f=w470:T6)
        n141 = property on="低切高阈值:" class="DigNum (严格)"("DisabledEnum"=w470) -> ()  [unwired: 2 in, 2 out]
        n142 = property on="高切低阈值:" class="DigNum (严格)"("DisabledEnum"=w470) -> ()  [unwired: 2 in, 2 out]
        n143 = property on="量程选择" class="Enum (严格)"("Disabled Items []"=w465) -> ()  [unwired: 2 in, 2 out]
        n144 = property on="采水泵进样时间/s:" class="DigNum (严格)"("Visible"=w463) -> ()  [unwired: 2 in, 2 out]
        n145 = property on="采水泵润洗时间/s:" class="DigNum (严格)"("Visible"=w463) -> ()  [unwired: 2 in, 2 out]
        n146 = property on="采水泵沉淀时间/s:" class="DigNum (严格)"("Visible"=w463) -> ()  [unwired: 2 in, 2 out]
        n147 = property on="采水泵排液时间/s:" class="DigNum (严格)"("Visible"=w463) -> ()  [unwired: 2 in, 2 out]
        n148 = property on="测量模式(公式)" class="Ring (严格)"("DisabledEnum"=w466) -> ()  [unwired: 2 in, 2 out]
        n149 = property on="一键写入" class="Bool (严格)"("DisabledEnum"=w464) -> ()  [unwired: 2 in, 2 out]
      }
    }
    n150 = Wait (ms)(milliseconds to wait=u32 1000 ("等待时间（毫秒）")) -> ()  [unwired: 1 out]
    n151 = flat-sequence {
      frame #0 {
        # "公式读取显示（只在读取公式的时候改变一次）"
        n152 = global read "COD读取DATA全局.vi" "读取公式显示"() -> (w192:bool)
        n153 = case shown="真" w192 {
          frame False {
          }
          frame True {
            n154 = global read "COD读取DATA全局.vi" "读取公式"() -> (w201:u16[])
            n155 = global write "COD读取DATA全局.vi" "读取公式显示"(FALSE ("读取参数显示")) -> ()
            n156 = local read "测量模式(公式)"() -> (w199:u16)
            n157 = Array Subset(array=w201, index=10 ("索引"), length=84 ("长度")) -> (w196:u16[])
            n158 = call "浮点CDAB转换COD.vi"("数组"=w196) -> ("数组 2"=w197:sgl[])  [unwired: 10 in]
            n159 = Array To Cluster(array=w197) -> (cluster=w200:T7)
            n160 = case shown="1" w199 {
              tunnel: [cluster{"X":dbl, "b":dbl, "X^2":dbl} {"X"=999.0, "b"=999.0, "X^2"=999.0} ("方程系数") w204 w223 w242 w261 w280 w299 w318] -> w198
              tunnel: w200 -> [_ w203 w222 w241 w260 w279 w298 w317]
              frame 0, Default {
              }
              frame 1 {
                n161 = local read "量程选择"() -> (w206:enum16{"低量程", "高量程", "0-2量程"})
                n162 = case shown="\"低量程\", 默认" w206 {
                  tunnel: w203 -> [w213 w217 w221]
                  tunnel: [w212 w216 w220] -> w209
                  tunnel: [w211 w215 w219] -> w208
                  tunnel: [w210 w214 w218] -> w207
                  frame "低量程", Default {
                    n163 = Unbundle By Name(w213) -> ("数组 2[0]"=w212:sgl, "数组 2[1]"=w211:sgl, "数组 2[2]"=w210:sgl)
                  }
                  frame "高量程" {
                    n164 = Unbundle By Name(w217) -> ("数组 2[3]"=w216:sgl, "数组 2[4]"=w215:sgl, "数组 2[5]"=w214:sgl)
                  }
                  frame "0-2量程" {
                    n165 = Unbundle By Name(w221) -> ("数组 2[6]"=w220:sgl, "数组 2[7]"=w219:sgl, "数组 2[8]"=w218:sgl)
                  }
                }
                n166 = Bundle By Name(cluster=cluster{"X":dbl, "b":dbl, "X^2":dbl} {"X"=0.0, "b"=0.0, "X^2"=0.0} ("方程系数"), "X"=w209, "b"=w208, "X^2"=w207) -> (w204:cluster{"X":dbl, "b":dbl, "X^2":dbl})
              }
              frame 2 {
                n167 = local read "量程选择"() -> (w225:enum16{"低量程", "高量程", "0-2量程"})
                n168 = case shown="\"高量程\"" w225 {
                  tunnel: w222 -> [w232 w236 w240]
                  tunnel: [w231 w235 w239] -> w228
                  tunnel: [w230 w234 w238] -> w227
                  tunnel: [w229 w233 w237] -> w226
                  frame "低量程", Default {
                    n169 = Unbundle By Name(w232) -> ("数组 2[6]"=w231:sgl, "数组 2[7]"=w230:sgl, "数组 2[8]"=w229:sgl)
                  }
                  frame "高量程" {
                    n170 = Unbundle By Name(w236) -> ("数组 2[9]"=w235:sgl, "数组 2[10]"=w234:sgl, "数组 2[11]"=w233:sgl)
                  }
                  frame "0-2量程" {
                    n171 = Unbundle By Name(w240) -> ("数组 2[6]"=w239:sgl, "数组 2[7]"=w238:sgl, "数组 2[8]"=w237:sgl)
                  }
                }
                n172 = Bundle By Name(cluster=cluster{"X":dbl, "b":dbl, "X^2":dbl} {"X"=0.0, "b"=0.0, "X^2"=0.0} ("方程系数"), "X"=w228, "b"=w227, "X^2"=w226) -> (w223:cluster{"X":dbl, "b":dbl, "X^2":dbl})
              }
              frame 3 {
                n173 = local read "量程选择"() -> (w244:enum16{"低量程", "高量程", "0-2量程"})
                n174 = case shown="\"高量程\"" w244 {
                  tunnel: w241 -> [w251 w255 w259]
                  tunnel: [w250 w254 w258] -> w247
                  tunnel: [w249 w253 w257] -> w246
                  tunnel: [w248 w252 w256] -> w245
                  frame "低量程", Default {
                    n175 = Unbundle By Name(w251) -> ("数组 2[12]"=w250:sgl, "数组 2[13]"=w249:sgl, "数组 2[14]"=w248:sgl)
                  }
                  frame "高量程" {
                    n176 = Unbundle By Name(w255) -> ("数组 2[15]"=w254:sgl, "数组 2[16]"=w253:sgl, "数组 2[17]"=w252:sgl)
                  }
                  frame "0-2量程" {
                    n177 = Unbundle By Name(w259) -> ("数组 2[6]"=w258:sgl, "数组 2[7]"=w257:sgl, "数组 2[8]"=w256:sgl)
                  }
                }
                n178 = Bundle By Name(cluster=cluster{"X":dbl, "b":dbl, "X^2":dbl} {"X"=0.0, "b"=0.0, "X^2"=0.0} ("方程系数"), "X"=w247, "b"=w246, "X^2"=w245) -> (w242:cluster{"X":dbl, "b":dbl, "X^2":dbl})
              }
              frame 4 {
                n179 = local read "量程选择"() -> (w263:enum16{"低量程", "高量程", "0-2量程"})
                n180 = case shown="\"高量程\"" w263 {
                  tunnel: w260 -> [w270 w274 w278]
                  tunnel: [w269 w273 w277] -> w266
                  tunnel: [w268 w272 w276] -> w265
                  tunnel: [w267 w271 w275] -> w264
                  frame "低量程", Default {
                    n181 = Unbundle By Name(w270) -> ("数组 2[18]"=w269:sgl, "数组 2[19]"=w268:sgl, "数组 2[20]"=w267:sgl)
                  }
                  frame "高量程" {
                    n182 = Unbundle By Name(w274) -> ("数组 2[21]"=w273:sgl, "数组 2[22]"=w272:sgl, "数组 2[23]"=w271:sgl)
                  }
                  frame "0-2量程" {
                    n183 = Unbundle By Name(w278) -> ("数组 2[6]"=w277:sgl, "数组 2[7]"=w276:sgl, "数组 2[8]"=w275:sgl)
                  }
                }
                n184 = Bundle By Name(cluster=cluster{"X":dbl, "b":dbl, "X^2":dbl} {"X"=0.0, "b"=0.0, "X^2"=0.0} ("方程系数"), "X"=w266, "b"=w265, "X^2"=w264) -> (w261:cluster{"X":dbl, "b":dbl, "X^2":dbl})
              }
              frame 5 {
                n185 = local read "量程选择"() -> (w282:enum16{"低量程", "高量程", "0-2量程"})
                n186 = case shown="\"高量程\"" w282 {
                  tunnel: w279 -> [w289 w293 w297]
                  tunnel: [w288 w292 w296] -> w285
                  tunnel: [w287 w291 w295] -> w284
                  tunnel: [w286 w290 w294] -> w283
                  frame "低量程", Default {
                    n187 = Unbundle By Name(w289) -> ("数组 2[24]"=w288:sgl, "数组 2[25]"=w287:sgl, "数组 2[26]"=w286:sgl)
                  }
                  frame "高量程" {
                    n188 = Unbundle By Name(w293) -> ("数组 2[27]"=w292:sgl, "数组 2[28]"=w291:sgl, "数组 2[29]"=w290:sgl)
                  }
                  frame "0-2量程" {
                    n189 = Unbundle By Name(w297) -> ("数组 2[6]"=w296:sgl, "数组 2[7]"=w295:sgl, "数组 2[8]"=w294:sgl)
                  }
                }
                n190 = Bundle By Name(cluster=cluster{"X":dbl, "b":dbl, "X^2":dbl} {"X"=0.0, "b"=0.0, "X^2"=0.0} ("方程系数"), "X"=w285, "b"=w284, "X^2"=w283) -> (w280:cluster{"X":dbl, "b":dbl, "X^2":dbl})
              }
              frame 6 {
                n191 = local read "量程选择"() -> (w301:enum16{"低量程", "高量程", "0-2量程"})
                n192 = case shown="\"高量程\"" w301 {
                  tunnel: w298 -> [w308 w312 w316]
                  tunnel: [w307 w311 w315] -> w304
                  tunnel: [w306 w310 w314] -> w303
                  tunnel: [w305 w309 w313] -> w302
                  frame "低量程", Default {
                    n193 = Unbundle By Name(w308) -> ("数组 2[30]"=w307:sgl, "数组 2[31]"=w306:sgl, "数组 2[32]"=w305:sgl)
                  }
                  frame "高量程" {
                    n194 = Unbundle By Name(w312) -> ("数组 2[33]"=w311:sgl, "数组 2[34]"=w310:sgl, "数组 2[35]"=w309:sgl)
                  }
                  frame "0-2量程" {
                    n195 = Unbundle By Name(w316) -> ("数组 2[6]"=w315:sgl, "数组 2[7]"=w314:sgl, "数组 2[8]"=w313:sgl)
                  }
                }
                n196 = Bundle By Name(cluster=cluster{"X":dbl, "b":dbl, "X^2":dbl} {"X"=0.0, "b"=0.0, "X^2"=0.0} ("方程系数"), "X"=w304, "b"=w303, "X^2"=w302) -> (w299:cluster{"X":dbl, "b":dbl, "X^2":dbl})
              }
              frame 7 {
                n197 = local read "量程选择"() -> (w320:enum16{"低量程", "高量程", "0-2量程"})
                n198 = case shown="\"高量程\"" w320 {
                  tunnel: w317 -> [w327 w331 w335]
                  tunnel: [w326 w330 w334] -> w323
                  tunnel: [w325 w329 w333] -> w322
                  tunnel: [w324 w328 w332] -> w321
                  frame "低量程", Default {
                    n199 = Unbundle By Name(w327) -> ("数组 2[36]"=w326:sgl, "数组 2[37]"=w325:sgl, "数组 2[38]"=w324:sgl)
                  }
                  frame "高量程" {
                    n200 = Unbundle By Name(w331) -> ("数组 2[39]"=w330:sgl, "数组 2[40]"=w329:sgl, "数组 2[41]"=w328:sgl)
                  }
                  frame "0-2量程" {
                    n201 = Unbundle By Name(w335) -> ("数组 2[6]"=w334:sgl, "数组 2[7]"=w333:sgl, "数组 2[8]"=w332:sgl)
                  }
                }
                n202 = Bundle By Name(cluster=cluster{"X":dbl, "b":dbl, "X^2":dbl} {"X"=0.0, "b"=0.0, "X^2"=0.0} ("方程系数"), "X"=w323, "b"=w322, "X^2"=w321) -> (w318:cluster{"X":dbl, "b":dbl, "X^2":dbl})
              }
            }
            n203 = local write "方程系数"(w198) -> ()
          }
        }
      }
    }
    n204 = flat-sequence {
      frame #0 {
        # "保存参数赋值"
        n205 = Multiply(x="温度", y=10.0) -> (x*y=w136:dbl)
        n206 = Multiply(x="标准液浓度", y=100.0) -> (x*y=w130:dbl)
        n207 = Multiply(x="修正系数", y=100.0) -> (x*y=w133:dbl)
        n208 = Build Array(w136, "恒温时间", w130, w133, "基本量程", "水样", "蒸馏水", "标液", "质控样", "加标回收", "高锰酸钾", "草酸钠", "硫酸", "零点泵计量数 2", "标度泵计量数 2", "高量程稀释倍数:", "低量程稀释倍数:", "CODMn零点核查选择") -> (w127:dbl[])
        n209 = local write "保存参数"(w127) -> ()
      }
    }
    n210 = flat-sequence {
      frame #0 {
        w363 = T8 0 items=["最小二乘", "最小绝对残差", "Bisquare"] ("method")
        # "计算线性、多项式公式"
        n211 = local read "浓度5"() -> (w357:dbl)
        n212 = local read "浓度4"() -> (w358:dbl)
        n213 = local read "浓度2"() -> (w367:dbl)
        n214 = local read "浓度3"() -> (w368:dbl)
        n215 = local read "浓度1"() -> (w366:dbl)
        n216 = Build Array("启用1", "启用2", "启用3", "启用4", "启用5") -> (w351:bool[])
        n217 = Build Array(w366, w367, w368, w358, w357) -> (w365:dbl[])
        n218 = Build Array("泵滴定数1", "泵滴定数2", "泵滴定数3", "泵滴定数4", "泵滴定数5") -> (w364:dbl[])
        n219 = call "线性公式CODMn用.vi"("标液浓度"=w365, "监测浓度"=w364, "启用"=w351, "method"=w363, "模型"="模型", "精度"=6) -> ("拟合方程"=w344:string, "r^2"=→"r^2":dbl, "slope"=w342:dbl, "intercept"=w343:dbl, "XY图"=→"XY图":cluster{"X Values":dbl[], "Y Values":dbl[]}[], "Polynomial Coefficients"=w359:dbl[])  [unwired: 8 in]
        "拟合公式" <- w344
        n220 = feedback-in #1(w344) -> ()
        n221 = feedback #1(w344) -> (w345:string)
        n222 = Not Equal?(x=w344, y=w345) -> (x != y?=w341:bool)
        n223 = case shown="真" w341 {
          tunnel: w359 -> [_ w376]
          tunnel: w343 -> [_ w378]
          tunnel: w342 -> [_ w379]
          frame False {
          }
          frame True {
            # "当公式发生改变时赋值到右侧公式"
            n224 = local read "模型"() -> (w381:enum32{"线性", "多项式"})
            n225 = case shown="\"多项式\"" w381 {
              tunnel: [w386 w388] -> w380
              tunnel: w379 -> [w386 _]
              tunnel: w378 -> [w385 _]
              tunnel: [w385 w389] -> w377
              tunnel: w376 -> [_ w390]
              tunnel: [0.0 ("数值") w387] -> w375
              frame "线性", Default {
              }
              frame "多项式" {
                # "B,K,X^2"
                n226 = Index Array(array=w390) -> (element #1=w389:dbl, element #2=w388:dbl, element #3=w387:dbl)  [unwired: 3 in]
              }
            }
            n227 = Bundle By Name(cluster=cluster{"K":dbl, "b":dbl, "X^2":dbl} {"K"=0.0, "b"=0.0, "X^2"=0.0} ("方程系数"), "K"=w380, "b"=w377, "X^2"=w375) -> (w382:cluster{"K":dbl, "b":dbl, "X^2":dbl})
            n228 = local write "方程系数"(w382) -> ()
          }
        }
        n229 = Unbundle By Name("方程系数") -> ("K"=w338:dbl, "b"=w337:dbl, "X^2"=w336:dbl)
        n230 = case shown="\"多项式\"" "模型" {
          tunnel: w338 -> [w370 w373]
          tunnel: w337 -> [w369 w374]
          tunnel: w336 -> [_ w372]
          frame "线性", Default {
            "K" <- w370
            "b" <- w369
          }
          frame "多项式" {
            n231 = Build Array(w374, w373, w372) -> (→"多项式系数":dbl[])
          }
        }
      }
    }
    n232 = flat-sequence {
      frame #0 {
        # "断电保存全局给局部变量"
        n233 = global read "CODMn断电保存全局变量.vi" "标样核查量程选择"() -> (w434:enum32{"H", "L", "AUTO"})
        n234 = global read "CODMn断电保存全局变量.vi" "零点核查量程选择"() -> (w436:enum32{"H", "L", "AUTO"})
        n235 = global read "CODMn断电保存全局变量.vi" "CODMn跨度量程选择"() -> (w444:enum32{"H", "L", "AUTO"})
        n236 = global read "CODMn断电保存全局变量.vi" "测量模式(公式)"() -> (w445:u16)
        n237 = global read "CODMn断电保存全局变量.vi" "常规版/认证版"() -> (w438:enum16{"常规版", "认证版", "浮台版"})
        n238 = global read "CODMn断电保存全局变量.vi" "自动切换量程:"() -> (w441:enum16{"关闭", "自动切换测一次", "自动切换测两次"})
        n239 = global read "CODMn断电保存全局变量.vi" "零点核查浓度"() -> (w435:dbl)
        n240 = global read "CODMn断电保存全局变量.vi" "高切低阈值:"() -> (w443:dbl)
        n241 = global read "CODMn断电保存全局变量.vi" "低切高阈值:"() -> (w442:dbl)
        n242 = global read "CODMn断电保存全局变量.vi" "标样浓度"() -> (w437:dbl)
        n243 = global read "CODMn断电保存全局变量.vi" "跨度液浓度"() -> (w440:dbl)
        n244 = global read "CODMn断电保存全局变量.vi" "启动时间"() -> (w439:timestamp)
        n245 = local write "标样核查量程选择"(w434) -> ()
        n246 = local write "零点核查量程选择"(w436) -> ()
        n247 = local write "测量模式(公式)"(w445) -> ()
        n248 = local write "零点核查浓度"(w435) -> ()
        n249 = local write "常规版/认证版"(w438) -> ()
        n250 = local write "自动切换量程:"(w441) -> ()
        n251 = local write "跨度量程选择"(w444) -> ()
        n252 = local write "低切高阈值:"(w442) -> ()
        n253 = local write "标样浓度"(w437) -> ()
        n254 = local write "跨度液浓度"(w440) -> ()
        n255 = local write "高切低阈值:"(w443) -> ()
        n256 = local write "启动时间"(w439) -> ()
      }
    }
    n257 = flat-sequence {
      frame #0 {
        # "局部变量给内部交互用全局变量"
        n258 = local read "CODMn工作状态"() -> (w155:T1)
        n259 = local read "COD浓度（mg/L)"() -> (w152:dbl)
        n260 = local read "标准液浓度"() -> (w151:dbl)
        n261 = local read "多列列表框"() -> (w153:i32)
        n262 = local read "故障标记"() -> (w154:bool)
        n263 = global write "COD测量模式全局.vi" "CODMn工作状态"(w155) -> ()
        n264 = global write "COD读取DATA全局.vi" "故障标记"(w154) -> ()
        n265 = global write "运行时序全局变量.vi" "多列列表框"(w153) -> ()
        n266 = global write "COD浓度全局变量.vi" "COD浓度（mg/L)"(w152) -> ()
        n267 = global write "COD浓度全局变量.vi" "标准液浓度"(w151) -> ()
      }
    }
  }
  n268 = while {
    shift-right: [w491] -> _
    shift-left: u16[] [] ("ORP滴定曲线") -> [w492]
    shift-right: [w486] -> _
    shift-left: 0.0 -> [w487]
    stop <- FALSE stop-if-true
    # "滴定数-ORP滴定曲线"
    n269 = local read "多列列表框"() -> (w490:i32)
    n270 = Wait (ms)(milliseconds to wait=u32 300 ("等待时间（毫秒）")) -> ()  [unwired: 1 out]
    n271 = Greater Or Equal?(x=w490, y=4) -> (x >= y?=w488:bool)
    n272 = case shown="真" w488 {
      tunnel: w492 -> [_ w511]
      tunnel: [u16[] [] ("ORP滴定曲线") w510] -> w491
      tunnel: w487 -> [_ w499]
      tunnel: [0.0 w498] -> w486
      frame False {
      }
      frame True {
        n273 = local read "高锰酸钾"() -> (w501:dbl)
        n274 = local read "多列列表框"() -> (w506:i32)
        n275 = local read "ORP显示"() -> (w507:dbl)
        n276 = Less?(x=w499, y=w501) -> (x < y?=w497:bool)
        n277 = Equal?(x=w506, y=5) -> (x = y?=w504:bool)
        n278 = call <vilib>:"Value Has Changed PtByPt.vi"("input data point"=w501) -> ("has changed"=w509:bool, "output data point"=w508:dbl)  [unwired: 1 in]
        n279 = call <vilib>:"Boolean Crossing PtByPt.vi"("direction"=enum16{"either", "false-true", "true-false"}."false-true", "input"=w504) -> ("crossing"=w502:bool)  [unwired: 1 in]
        n280 = Or(x=w497, y=w509) -> (x .or. y?=w500:bool)
        n281 = case shown="真" w500 {
          tunnel: w511 -> [w518 w532]
          tunnel: [w517 w531] -> w510
          tunnel: w508 -> [w519 w525]
          tunnel: w507 -> [w515 w530]
          tunnel: w499 -> [w514 w527]
          tunnel: [w514 w529] -> w498
          tunnel: w497 -> [_ w528]
          frame False {
            n282 = Equal To 0?(x=w519) -> (x = 0?=w516:bool)
            n283 = case shown="真" w516 {
              tunnel: [w520 w523] -> w517
              tunnel: w518 -> [w520 _]
              tunnel: w515 -> [_ w522]
              frame False {
              }
              frame True {
                n284 = Insert Into Array(array=u16[] [] ("ORP滴定曲线"), index=0 ("索引"), new element=w522) -> (w523:u16[])
                n285 = local write "滴定数-ORP值"(w523) -> ()
              }
            }
          }
          frame True {
            # "防止高锰酸钾不连续变大"
            n286 = case shown="假" w528 {
              tunnel: w527 -> [_ w536]
              tunnel: [w535 w536] -> w526
              tunnel: w525 -> [w535 _]
              frame False {
              }
              frame True {
              }
            }
            n287 = Increment(x=w527) -> (x+1=w529:dbl)
            n288 = Insert Into Array(array=w532, index=w526, new element=w530) -> (w531:u16[])
            "滴定数-ORP值" <- w531
            n289 = Insert Into Array(array=u16[] [] ("ORP滴定曲线"), new element=w531) -> (→"ORP滴定曲线":u16[])  [unwired: 1 in]
          }
        }
        n290 = case shown="真" w502 {
          frame False {
          }
          frame True {
            n291 = Get Date/Time In Seconds() -> (seconds since 1Jan1904=w512:timestamp)
            n292 = local write "波形时间"(w512) -> ()
            n293 = local read "ORP滴定曲线"() -> (w513:u16[])
            n294 = call "波形存储(子VI).vi"("ORP滴定曲线"=w513) -> ()  [unwired: 11 in]
          }
        }
      }
    }
  }
  n295 = while {
    shift-right: [w542] -> _
    shift-left: enum16{"待机", "启动COD", "COD测量中", "延时"}."待机" -> [w541]
    stop <- FALSE stop-if-true
    # "定时启动循环"
    n296 = global read "CODMn断电保存全局变量.vi" "定时控制"() -> (w538:T10)
    n297 = Wait (ms)(milliseconds to wait=u32 1000 ("等待时间（毫秒）")) -> ()  [unwired: 1 out]
    n298 = Unbundle By Name(w538) -> ("定时功能启用"=→"定时启动":bool)
    n299 = local read "定时启动"() -> (w539:bool)
    n300 = case shown="真" w539 {
      tunnel: w541 -> [_ w597]
      tunnel: [_ w596] -> w540
      frame False {
      }
      frame True {
        n301 = global read "CODMn断电保存全局变量.vi" "定时控制"() -> (w595:T10)
        n302 = Unbundle By Name(w595) -> ("周期设置类型"=w598:enum16{"定点启动", "间隔启动"}, "定时间隔"=w599:dbl, "24H周期设置"=w600:bool[])  [unwired: 1 out]
        n303 = case shown="\"间隔启动\"" w598 {
          tunnel: w599 -> [_ w617]
          tunnel: w600 -> [w603 _]
          tunnel: w597 -> [w601 w620]
          tunnel: [w602 w615] -> w596
          frame "定点启动", Default {
            n304 = case shown="\"待机\", 默认" w601 {
              tunnel: w603 -> [w611 _]
              tunnel: [w604 _] -> w602
              frame "待机", Default {
                n305 = Get Date/Time In Seconds() -> (seconds since 1Jan1904=w613:timestamp)
                n306 = Seconds To Date/Time(time stamp (now)=w613) -> (date time rec=w612:T11)  [unwired: 1 in]
                n307 = Unbundle By Name(w612) -> ("时"=w610:i32, "分"=w608:i32, "秒"=w609:i32)
                n308 = Equal To 0?(x=w608) -> (x = 0?=w606:bool)
                n309 = Equal To 0?(x=w609) -> (x = 0?=w605:bool)
                n310 = Index Array(array=w611, index=w610) -> (element=w607:bool)
                n311 = Compound Arithmetic op=AND ("复合运算")(w607, w606, w605) -> (w604:bool)
              }
              frame "启动COD" {
              }
            }
          }
          frame "间隔启动" {
            n312 = Multiply(x=w617, y=60.0) -> (x*y=w614:dbl)
            n313 = feedback #2(w614) -> (w619:dbl)
            n314 = case shown="\"待机\"" w620 {
              tunnel: w619 -> [_ w622]
              tunnel: [_ w621] -> w618
              frame Default {
              }
              frame "待机" {
                n315 = Increment(x=w622) -> (x+1=w621:dbl)
              }
            }
            n316 = feedback-in #2(w618) -> ()
            n317 = Greater Or Equal?(x=w618, y=w614) -> (x >= y?=w615:bool)
          }
        }
      }
    }
    n318 = case shown="\"启动COD\"" w541 {
      tunnel: [w545 w551 w585 enum16{"待机", "启动COD", "COD测量中", "延时"}."待机"] -> w542
      tunnel: w540 -> [w548 _ _ _]
      frame "待机", Default {
        n319 = Select(t=enum16{"待机", "启动COD", "COD测量中", "延时"}."启动COD", s=w548, f=enum16{"待机", "启动COD", "COD测量中", "延时"}."待机") -> (s? t:f=w545:enum16{"待机", "启动COD", "COD测量中", "延时"})
      }
      frame "启动COD" {
        n320 = global read "CODMn断电保存全局变量.vi" "定时控制"() -> (w549:T10)
        n321 = Unbundle By Name(w549) -> ("仪器测试类型"=w550:T12)
        n322 = flat-sequence {
          tunnel: w550 -> [w555]
          tunnel: [enum16{"待机", "启动COD", "COD测量中", "延时"}."COD测量中"] -> w551
          frame #0 {
            n323 = case shown="\"标样核查\"" w555 {
              tunnel: [T9 {"测量模式"=enum."水样测量"} ("启动测量模式") T9 {"测量模式"=enum."标样核查"} ("启动测量模式") T9 {"测量模式"=enum."空白测试"} ("启动测量模式") T9 {"测量模式"=enum."跨度核查"} ("启动测量模式") T9 {"测量模式"=enum."加标回收"} ("启动测量模式") T9 {"测量模式"=enum."平行样"} ("启动测量模式") T9 {"测量模式"=enum."校零"} ("启动测量模式") T9 {"测量模式"=enum."校标"} ("启动测量模式") T9 {"测量模式"=enum."零点核查"} ("启动测量模式")] -> w554
              tunnel: ["水样测试" ("测量模式") "标样核查" ("测量模式") "空白测试" ("测量模式") "跨度核查" ("测量模式") "加标回收" ("测量模式") "平行样" ("测量模式") "校零" ("测量模式") "校标" ("测量模式") "零点核查" ("测量模式")] -> w553
              tunnel: [enum32{"H", "L", "AUTO"}."AUTO" ("CODMn跨度量程选择") w559 enum32{"H", "L", "AUTO"}."L" ("CODMn跨度量程选择") w565 enum32{"H", "L", "AUTO"}."AUTO" ("CODMn跨度量程选择") enum32{"H", "L", "AUTO"}."AUTO" ("CODMn跨度量程选择") enum32{"H", "L", "AUTO"}."L" ("CODMn跨度量程选择") enum32{"H", "L", "AUTO"}."AUTO" ("CODMn跨度量程选择") w580] -> w552
              frame "水样测试", Default {
              }
              frame "标样核查" {
                n324 = local read "标样核查量程选择"() -> (w559:enum32{"H", "L", "AUTO"})
              }
              frame "空白测试" {
              }
              frame "跨度核查" {
                n325 = local read "跨度量程选择"() -> (w565:enum32{"H", "L", "AUTO"})
              }
              frame "加标回收" {
              }
              frame "平行样" {
              }
              frame "校零" {
              }
              frame "校标" {
              }
              frame "零点核查" {
                n326 = local read "零点核查量程选择"() -> (w580:enum32{"H", "L", "AUTO"})
              }
            }
            n327 = global write "COD测量模式全局.vi" "测量模式"(w553) -> ()
            n328 = call "CODMn启动命令 (子VI).vi"("CODMn量程切换"=w552, "启动测量模式"=w554) -> ()  [unwired: 10 in]
          }
          frame #1 {
          }
        }
      }
      frame "COD测量中" {
        n329 = flat-sequence {
          tunnel: [w586] -> w584
          tunnel: [w593] -> w585
          tunnel: w584 -> [w593]
          frame #0 {
            n330 = global read "运行时序全局变量.vi" "多列列表框"() -> (w591:i32)
            n331 = Equal?(x=w591, y=0) -> (x = y?=w589:bool)
            n332 = Select(t=enum16{"待机", "启动COD", "COD测量中", "延时"}."延时", s=w589, f=enum16{"待机", "启动COD", "COD测量中", "延时"}."COD测量中") -> (s? t:f=w586:enum16{"待机", "启动COD", "COD测量中", "延时"})
          }
          frame #1 {
            n333 = Wait (ms)(milliseconds to wait=u32 5000 ("等待时间（毫秒）")) -> ()  [unwired: 1 out]
          }
        }
      }
      frame "延时" {
      }
    }
  }
  n334 = while {
    stop <- FALSE stop-if-true
    # "相差60秒自动校时"
    n335 = local read "仪器时间"() -> (w626:timestamp)
    n336 = local read "系统时间"() -> (w627:timestamp)
    n337 = Build Array(w626) -> (w625:timestamp[])
    n338 = call "DateToHex.vi"("DATE"=w625) -> ("数组"=w638:u16[])  [unwired: 10 in]
    n339 = Build Array(w627) -> (w644:timestamp[])
    n340 = call "DateToHex.vi"("DATE"=w644) -> ("数组"=w643:u16[])  [unwired: 10 in]
    n341 = Index Array(array=w638, index=2 ("索引")) -> (element=w640:u16)
    n342 = Index Array(array=w643, index=2 ("索引")) -> (element=w641:u16)
    n343 = Split Number(x=w640) -> (hi(x)=w634:u8)  [unwired: 1 out]
    n344 = Split Number(x=w641) -> (hi(x)=w637:u8)  [unwired: 1 out]
    n345 = To Byte Integer(number=w634) -> (8bit integer=w633:i8)
    n346 = To Byte Integer(number=w637) -> (8bit integer=w636:i8)
    n347 = Subtract(x=w633, y=w636) -> (x-y=w635:i8)
    n348 = local read "通讯状态"() -> (w629:bool)
    n349 = Absolute Value(x=w635) -> (abs(x)=w632:i8)
    n350 = Wait (ms)(milliseconds to wait=u32 1000 ("等待时间（毫秒）")) -> ()  [unwired: 1 out]
    n351 = Greater Or Equal?(x=w632, y=i8 60) -> (x >= y?=w630:bool)
    n352 = And(x=w630, y=w629) -> (x .and. y?=w628:bool)
    n353 = case shown="真" w628 {
      frame False {
      }
      frame True {
        # "相差60秒时间自动校准"
        n354 = flat-sequence {
          frame #0 {
            n355 = property on="时间校准" class="Bool (严格)"("Val(Sgnl)"=TRUE ("值(信号)")) -> ()  [unwired: 2 in, 2 out]
          }
          frame #1 {
            n356 = Wait (ms)(milliseconds to wait=u32 500 ("等待时间（毫秒）")) -> ()  [unwired: 1 out]
          }
          frame #2 {
            n357 = property on="时间校准" class="Bool (严格)"("Val(Sgnl)"=FALSE ("值(信号)")) -> ()  [unwired: 2 in, 2 out]
          }
        }
      }
    }
  }
  n358 = while {
    stop <- FALSE stop-if-true
    # "存储数据入队列、日志存储、报警存储"
    n359 = local read "多列列表框"() -> (w648:i32)
    n360 = First Call?() -> (First Call?: T/F=w651:bool)
    n361 = local read "报警簇"() -> (w652:T3)
    n362 = Not(x=w651) -> (.not. x?=w649:bool)
    n363 = call "CODMn报警信息.vi"("报警簇"=w652) -> ("CODMN报警信息"=w653:string)  [unwired: 10 in]
    n364 = case shown="真" w649 {
      selector: w649 -> [w676 _]
      tunnel: w648 -> [_ w678]
      tunnel: [w676 w677] -> w650
      frame False {
      }
      frame True {
        # "非初次调用"
        n365 = Greater?(x=w678, y=u16 0) -> (0:w681:bool)
        n366 = call <vilib>:"Boolean Crossing PtByPt.vi"("direction"=enum16{"either", "false-true", "true-false"}."false-true", "input"=w681) -> ("crossing"=w677:bool)  [unwired: 1 in]
      }
    }
    n367 = feedback #3(w648) -> (w664:i32)
    n368 = feedback-in #3(w648) -> ()
    n369 = Greater?(x=w648, y=u16 0) -> (0:w675:bool)
    n370 = Less Or Equal?(x=w648, y=u16 5) -> (x <= y?=w672:bool)
    n371 = local read "断电排液标记"() -> (w660:bool)
    n372 = feedback #4(w653) -> (w654:string)
    n373 = feedback-in #4(w653) -> ()
    n374 = Not Equal?(x=w653, y="") -> (x != y?=w658:bool)
    n375 = Equal?(x=w648, y=u16 5) -> (x = y?=w668:bool)
    n376 = Not Equal?(x=w648, y=w664) -> (x != y?=w665:bool)
    n377 = Not Equal?(x=w653, y=w654) -> (x != y?=w655:bool)
    n378 = And(x=w675, y=w672) -> (x .and. y?=w673:bool)
    n379 = call <vilib>:"Boolean Crossing PtByPt.vi"("direction"=enum16{"either", "false-true", "true-false"}."false-true", "input"=w668) -> ("crossing"=w670:bool)  [unwired: 1 in]
    n380 = And(x=w655, y=w658) -> (x .and. y?=w656:bool)
    n381 = call <vilib>:"Boolean Crossing PtByPt.vi"("direction"=enum16{"either", "false-true", "true-false"}."false-true", "input"=w660) -> ("crossing"=w659:bool)  [unwired: 1 in]
    n382 = First Call?() -> (First Call?: T/F=w666:bool)
    n383 = case shown="假" w666 {
      tunnel: w665 -> [w704 _]
      tunnel: w648 -> [w703 _]
      frame False {
        # "初次调用不存日志，防止软件重启重复存储日志"
        n384 = case shown="真" w704 {
          tunnel: w703 -> [_ w706]
          frame False {
          }
          frame True {
            # "步骤发生改变存储日志"
            n385 = flat-sequence {
              tunnel: w706 -> [w707]
              tunnel: [w707] -> w705
              tunnel: w705 -> [w727]
              frame #0 {
                n386 = case shown="1" w707 {
                  frame 0 {
                    n387 = global read "COD测量模式全局.vi" "测量模式"() -> (w714:string)
                    n388 = Concatenate Strings("-->", w714, "结束" ("字符串")) -> (w713:string)
                    n389 = call "CODMn日志存储 (子VI).vi"("table输入"="操作日志", "参数"="CODMn" ("table输入"), "日志信息"=w713, "database"="database3.mdb") -> ()  [unwired: 8 in]
                  }
                  frame 1 {
                    n390 = property on="CODMn工作状态" class="Enum (严格)"() -> ("RingText.Text"=w717:string)  [unwired: 2 in, 2 out]
                    n391 = Concatenate Strings("-->", w717, "启动" ("字符串")) -> (w715:string)
                    n392 = call "CODMn日志存储 (子VI).vi"("table输入"="操作日志", "参数"="CODMn" ("table输入"), "日志信息"=w715, "database"="database3.mdb") -> ()  [unwired: 8 in]
                  }
                  frame 2, Default {
                  }
                }
              }
              frame #1 {
                n393 = property on="多列列表框" class="MCListbox (严格)"() -> ("ItemNames"=w725:string[][])  [unwired: 2 in, 2 out]
                n394 = Index Array(array=w725, index (row)=w727) -> (element=w724:string[])  [unwired: 1 in]
                n395 = Index Array(array=w724, index=0 ("索引")) -> (element=w722:string)
                n396 = call "CODMn日志存储 (子VI).vi"("table输入"="操作日志", "参数"="CODMn" ("table输入"), "日志信息"=w722, "database"="database3.mdb") -> ()  [unwired: 8 in]
              }
            }
          }
        }
      }
      frame True {
      }
    }
    n397 = case shown="真" w659 {
      frame False {
      }
      frame True {
        n398 = Get Date/Time In Seconds() -> (seconds since 1Jan1904=w697:timestamp)
        n399 = Bundle(cluster=T14 {"时间标识"=timestamp(0 s since 1904-01-01), "参数"="", "日志信息"="", "流程参数"=""} ("data in"), "时间标识"=w697, "参数"="CODMn" ("table输入"), "日志信息"="断电排液", "流程参数"="" ("table输入")) -> (w695:T14)
        n400 = call "流程日志字段定义.vi"("table输入"="操作日志", "data in"=w695) -> ("table输出"=w700:string, "columns"=w701:string[], "data out"=w702:T15)  [unwired: 7 in]
        n401 = call "插入数据.vi"("data"=w702, "columns"=w701, "database"="database3.mdb", "table"=w700) -> ()  [unwired: 7 in, 1 out]
      }
    }
    n402 = case shown="真" w656 {
      tunnel: w653 -> [_ w682]
      frame False {
      }
      frame True {
        n403 = Get Date/Time In Seconds() -> (seconds since 1Jan1904=w684:timestamp)
        n404 = Bundle By Name(cluster=T13 {"时间标识"=timestamp(0 s since 1904-01-01), "设备"="", "日志信息"=""} ("data in"), "时间标识"=w684, "设备"="CODMn", "日志信息"=w682) -> (w685:T13)
        n405 = call "报警信息字段定义.vi"("table输入"="报警信息", "data in"=w685) -> ("table输出"=w689:string, "columns"=w690:string[], "data out"=w691:T13)  [unwired: 7 in]
        n406 = call "插入数据.vi"("data"=w691, "columns"=w690, "database"="database3.mdb", "table"=w689) -> ()  [unwired: 7 in, 1 out]
      }
    }
    n407 = case shown="真" w673 {
      frame False {
      }
      frame True {
        # "测量过程中记录测量模式，为存储数据做准备，待机状态变量不更新"
        n408 = flat-sequence {
          frame #0 {
            n409 = local read "标样核查标记"() -> (w755:bool)
            n410 = local read "零点核查标记"() -> (w754:bool)
            n411 = local read "跨度核查标记"() -> (w752:bool)
            n412 = local read "空白测试标记"() -> (w751:bool)
            n413 = local read "加标回收测量"() -> (w750:bool)
            n414 = local read "平行样测量"() -> (w749:bool)
            n415 = local read "水样测量"() -> (w756:bool)
            n416 = local read "校零标记"() -> (w748:bool)
            n417 = local read "校标标记"() -> (w747:bool)
            n418 = Build Array(w756, w755, w754, w752, w751, w750, w749, w748, w747) -> (w753:bool[])
            n419 = for {
              tunnel: w753 -> [w758] mode=indexing
              i -> [w757]
              n420 = case shown="真" w758 {
                tunnel: w757 -> [_ w759]
                frame False {
                }
                frame True {
                  "测量模式数字" <- w759
                }
              }
            }
          }
          frame #1 {
            n421 = local read "测量模式数字"() -> (w762:i32)
            n422 = local read "启动时间"() -> (w760:timestamp)
            n423 = case shown="6" w762 {
              tunnel: ["水样测试" ("测量模式") "标样核查" ("测量模式") "零点核查" ("测量模式") "跨度核查" ("测量模式") "空白测试" ("测量模式") "加标回收" ("测量模式") "平行样" ("测量模式") "校零" ("测量模式") "校标" ("测量模式")] -> w761
              tunnel: w760 -> [w763 _ _ _ _ w769 _ _ _]
              frame 0, Default {
                n424 = global write "COD测量模式全局.vi" "水样启动时间"(w763) -> ()
              }
              frame 1 {
              }
              frame 2 {
              }
              frame 3 {
              }
              frame 4 {
              }
              frame 5 {
                n425 = global write "COD测量模式全局.vi" "加标回收启动时间"(w769) -> ()
              }
              frame 6 {
              }
              frame 7 {
              }
              frame 8 {
              }
            }
            n426 = global write "COD测量模式全局.vi" "测量模式"(w761) -> ()
          }
        }
      }
    }
    n427 = case shown="真" w650 {
      frame False {
      }
      frame True {
        # "非初次调用记录启动时间"
        n428 = flat-sequence {
          frame #0 {
            n429 = local read "切换量程连续测两次"() -> (w730:bool)
            n430 = case shown="假" w730 {
              frame False {
                n431 = Get Date/Time In Seconds() -> (seconds since 1Jan1904=w731:timestamp)
                "启动时间" <- w731
                n432 = global write "CODMn断电保存全局变量.vi" "启动时间"(w731) -> ()
              }
              frame True {
                n433 = local write "切换量程连续测两次"(FALSE ("切换量程连续测两次")) -> ()
              }
            }
          }
          frame #1 {
            n434 = global read "COD读取DATA全局.vi" "配置文件ini"() -> (w733:string)
            n435 = call <vilib>:"Application Directory.vi"() -> ("Application Directory"=w746:path)
            n436 = Build Path(base path=w746, name or relative path=w733) -> (appended path=w745:path)
            n437 = call <vilib>:"Open Config Data.vi"("configuration file path"=w745) -> ("error out"=w741:errorcluster, "refnum"=w744:T16)  [unwired: 8 in, 1 out]
            n438 = vi-ref "斯坦道CODMn.lvlib:CODMn断电保存全局变量.vi"() -> (w743:refnum<vi>)
            n439 = call <userlib>:"Write Panel to INI__ogtk.vi"("error in (no error)"=w741, "VI ref"=w743, "refnum"=w744) -> ("error out"=w740:errorcluster, "refnum out"=w742:T16)  [unwired: 7 in]
            n440 = call <vilib>:"Close Config Data.vi"("error in (no error)"=w740, "refnum"=w742) -> ("error out"=w735:errorcluster, "file path"=w734:path)  [unwired: 8 in]
            n441 = Open/Create/Replace File(file path (use dialog)=w734, error in=w735) -> (refnum out=w738:refnum<file>, error out=w739:errorcluster)  [unwired: 4 in, 1 out]
            n442 = Flush File(refnum=w738, error in=w739) -> (refnum out=w737:refnum<file>, error out=w736:errorcluster)
            n443 = Close File(refnum=w737, error in=w736) -> ()  [unwired: 2 out]
          }
        }
      }
    }
    n444 = case shown="真" w670 {
      frame False {
      }
      frame True {
        # "排液步骤存数据，第5步数据存储时间戳更新，防止启动停止数据存储"
        n445 = call "数据写入入队列 (子VI).vi"() -> ()  [unwired: 12 in]
        n446 = global read "CODMn断电保存全局变量.vi" "启动时间"() -> (w779:timestamp)
        n447 = local read "温度"() -> (w774:dbl)
        n448 = global write "COD读取DATA全局.vi" "温度存储数据用"(w774) -> ()
        n449 = global write "COD读取DATA全局.vi" "数据存储时间戳"(w779) -> ()
        n450 = global read "COD测量模式全局.vi" "测量模式"() -> (w778:string)
        n451 = local read "高锰酸钾"() -> (w775:dbl)
        n452 = Equal?(x=w778, y="校标") -> (x = y?=w776:bool)
        n453 = case shown="真" w776 {
          tunnel: w775 -> [_ w780]
          frame False {
          }
          frame True {
            n454 = local read "当前校准"() -> (w781:i32)
            n455 = case shown="3" w781 {
              tunnel: w780 -> [w782 w783 w784 w785 w786]
              frame 1, Default {
                n456 = local write "泵滴定数1"(w782) -> ()
              }
              frame 2 {
                n457 = local write "泵滴定数2"(w783) -> ()
              }
              frame 3 {
                n458 = local write "泵滴定数3"(w784) -> ()
              }
              frame 4 {
                n459 = local write "泵滴定数4"(w785) -> ()
              }
              frame 5 {
                n460 = local write "泵滴定数5"(w786) -> ()
              }
            }
          }
        }
      }
    }
    n461 = Wait (ms)(milliseconds to wait=u32 1000 ("等待时间（毫秒）")) -> ()  [unwired: 1 out]
  }
  n462 = while {
    stop <- FALSE stop-if-true
    # "数字键盘输入"
    n463 = event shown="[22] \"跨度液浓度\", \"零点核查浓度\", \"标样浓度\": 鼠标按下" {
      selector: _ -> [_ _ _ _ _ _ _ _ _ _ _ _ _ _ _ _ _ _ _ _ _ _ _ _ _ _ _ _ _]
      dyn-events: _ -> [_ _ _ _ _ _ _ _ _ _ _ _ _ _ _ _ _ _ _ _ _ _ _ _ _ _ _ _ _]
      timeout: _ -> [_ _ _ _ _ _ _ _ _ _ _ _ _ _ _ _ _ _ _ _ _ _ _ _ _ _ _ _ _]
      event Timeout {
        n464 = event-data() -> ()  [unwired: 1 in, 3 out]
      }
      event "温度": Mouse Down {
        n465 = event-data() -> ()  [unwired: 1 in, 8 out]
        n466 = local read "温度"() -> (w789:dbl)
        n467 = call "数字键盘.vi"("OldNumber"=w789) -> ("NewNumber"=w788:sgl)
        n468 = local write "温度"(w788) -> ()
      }
      event "恒温时间": Mouse Down {
        n469 = event-data() -> ()  [unwired: 1 in, 8 out]
        n470 = local read "恒温时间"() -> (w790:dbl)
        n471 = call "数字键盘.vi"("OldNumber"=w790) -> ("NewNumber"=w791:sgl)
        n472 = local write "恒温时间"(w791) -> ()
      }
      event "标准液浓度": Mouse Down {
        n473 = event-data() -> ()  [unwired: 1 in, 8 out]
        n474 = local read "标准液浓度"() -> (w793:dbl)
        n475 = call "数字键盘.vi"("OldNumber"=w793) -> ("NewNumber"=w792:sgl)
        n476 = local write "标准液浓度"(w792) -> ()
      }
      event "修正系数": Mouse Down {
        n477 = event-data() -> ()  [unwired: 1 in, 8 out]
        n478 = local read "修正系数"() -> (w794:dbl)
        n479 = call "数字键盘.vi"("OldNumber"=w794) -> ("NewNumber"=w795:sgl)
        n480 = local write "修正系数"(w795) -> ()
      }
      event "水样": Mouse Down {
        n481 = event-data() -> ()  [unwired: 1 in, 8 out]
        n482 = local read "水样"() -> (w796:dbl)
        n483 = call "数字键盘.vi"("OldNumber"=w796) -> ("NewNumber"=w797:sgl)
        n484 = local write "水样"(w797) -> ()
      }
      event "蒸馏水": Mouse Down {
        n485 = event-data() -> ()  [unwired: 1 in, 8 out]
        n486 = local read "蒸馏水"() -> (w798:dbl)
        n487 = call "数字键盘.vi"("OldNumber"=w798) -> ("NewNumber"=w799:sgl)
        n488 = local write "蒸馏水"(w799) -> ()
      }
      event "标液": Mouse Down {
        n489 = event-data() -> ()  [unwired: 1 in, 8 out]
        n490 = local read "标液"() -> (w800:dbl)
        n491 = call "数字键盘.vi"("OldNumber"=w800) -> ("NewNumber"=w801:sgl)
        n492 = local write "标液"(w801) -> ()
      }
      event "质控样": Mouse Down {
        n493 = event-data() -> ()  [unwired: 1 in, 8 out]
        n494 = local read "质控样"() -> (w802:dbl)
        n495 = call "数字键盘.vi"("OldNumber"=w802) -> ("NewNumber"=w803:sgl)
        n496 = local write "质控样"(w803) -> ()
      }
      event "加标回收": Mouse Down {
        n497 = event-data() -> ()  [unwired: 1 in, 8 out]
        n498 = local read "加标回收"() -> (w804:dbl)
        n499 = call "数字键盘.vi"("OldNumber"=w804) -> ("NewNumber"=w805:sgl)
        n500 = local write "加标回收"(w805) -> ()
      }
      event "草酸钠": Mouse Down {
        n501 = event-data() -> ()  [unwired: 1 in, 8 out]
        n502 = local read "草酸钠"() -> (w806:dbl)
        n503 = call "数字键盘.vi"("OldNumber"=w806) -> ("NewNumber"=w807:sgl)
        n504 = local write "草酸钠"(w807) -> ()
      }
      event "高锰酸钾": Mouse Down {
        n505 = event-data() -> ()  [unwired: 1 in, 8 out]
        n506 = local read "高锰酸钾"() -> (w808:dbl)
        n507 = call "数字键盘.vi"("OldNumber"=w808) -> ("NewNumber"=w809:sgl)
        n508 = local write "高锰酸钾"(w809) -> ()
      }
      event "硫酸": Mouse Down {
        n509 = event-data() -> ()  [unwired: 1 in, 8 out]
        n510 = local read "硫酸"() -> (w810:dbl)
        n511 = call "数字键盘.vi"("OldNumber"=w810) -> ("NewNumber"=w811:sgl)
        n512 = local write "硫酸"(w811) -> ()
      }
      event "零点泵计量数 2": Mouse Down {
        n513 = event-data() -> ()  [unwired: 1 in, 8 out]
        n514 = local read "零点泵计量数 2"() -> (w812:dbl)
        n515 = call "数字键盘.vi"("OldNumber"=w812) -> ("NewNumber"=w813:sgl)
        n516 = local write "零点泵计量数 2"(w813) -> ()
      }
      event "标度泵计量数 2": Mouse Down {
        n517 = event-data() -> ()  [unwired: 1 in, 8 out]
        n518 = local read "标度泵计量数 2"() -> (w814:dbl)
        n519 = call "数字键盘.vi"("OldNumber"=w814) -> ("NewNumber"=w815:sgl)
        n520 = local write "标度泵计量数 2"(w815) -> ()
      }
      event "高量程稀释倍数:": Mouse Down {
        n521 = event-data() -> ()  [unwired: 1 in, 8 out]
        n522 = local read "高量程稀释倍数:"() -> (w817:i8)
        n523 = call "数字键盘.vi"("OldNumber"=w817) -> ("NewNumber"=w816:sgl)
        n524 = local write "高量程稀释倍数:"(w816) -> ()
      }
      event "低量程稀释倍数:": Mouse Down {
        n525 = event-data() -> ()  [unwired: 1 in, 8 out]
        n526 = local read "低量程稀释倍数:"() -> (w819:i8)
        n527 = call "数字键盘.vi"("OldNumber"=w819) -> ("NewNumber"=w818:sgl)
        n528 = local write "低量程稀释倍数:"(w818) -> ()
      }
      event "浓度1": Mouse Down {
        n529 = event-data() -> ()  [unwired: 1 in, 8 out]
        n530 = local read "浓度1"() -> (w821:dbl)
        n531 = call "数字键盘.vi"("OldNumber"=w821) -> ("NewNumber"=w820:sgl)
        n532 = property on="浓度1" class="DigNum (严格)"("Val(Sgnl)"=w820) -> ()  [unwired: 2 in, 2 out]
      }
      event "浓度2": Mouse Down {
        n533 = event-data() -> ()  [unwired: 1 in, 8 out]
        n534 = local read "浓度2"() -> (w823:dbl)
        n535 = call "数字键盘.vi"("OldNumber"=w823) -> ("NewNumber"=w822:sgl)
        n536 = property on="浓度2" class="DigNum (严格)"("Val(Sgnl)"=w822) -> ()  [unwired: 2 in, 2 out]
      }
      event "浓度3": Mouse Down {
        n537 = event-data() -> ()  [unwired: 1 in, 8 out]
        n538 = local read "浓度3"() -> (w825:dbl)
        n539 = call "数字键盘.vi"("OldNumber"=w825) -> ("NewNumber"=w824:sgl)
        n540 = property on="浓度3" class="DigNum (严格)"("Val(Sgnl)"=w824) -> ()  [unwired: 2 in, 2 out]
      }
      event "浓度4": Mouse Down {
        n541 = event-data() -> ()  [unwired: 1 in, 8 out]
        n542 = local read "浓度4"() -> (w827:dbl)
        n543 = call "数字键盘.vi"("OldNumber"=w827) -> ("NewNumber"=w826:sgl)
        n544 = property on="浓度4" class="DigNum (严格)"("Val(Sgnl)"=w826) -> ()  [unwired: 2 in, 2 out]
      }
      event "浓度5": Mouse Down {
        n545 = event-data() -> ()  [unwired: 1 in, 8 out]
        n546 = local read "浓度5"() -> (w829:dbl)
        n547 = call "数字键盘.vi"("OldNumber"=w829) -> ("NewNumber"=w828:sgl)
        n548 = property on="浓度5" class="DigNum (严格)"("Val(Sgnl)"=w828) -> ()  [unwired: 2 in, 2 out]
      }
      event "跨度液浓度", "零点核查浓度", "标样浓度": Mouse Down {
        n549 = event-data() -> ("CtlRef"=w833:refnum<vi>)  [unwired: 1 in, 7 out]
        n550 = property class="DigNum (严格)"(reference=w833) -> (reference out=w830:refnum<vi>, "Value"=w832:dbl)  [unwired: 1 in, 1 out]
        n551 = call "数字键盘.vi"("OldNumber"=w832) -> ("NewNumber"=w831:sgl)
        n552 = property class="DigNum (严格)"(reference=w830, "Val(Sgnl)"=w831) -> ()  [unwired: 1 in, 2 out]
      }
      event "泵滴定数1": Mouse Down {
        n553 = event-data() -> ()  [unwired: 1 in, 8 out]
        n554 = local read "泵滴定数1"() -> (w835:dbl)
        n555 = call "数字键盘.vi"("OldNumber"=w835) -> ("NewNumber"=w834:sgl)
        n556 = property on="泵滴定数1" class="DigNum (严格)"("Val(Sgnl)"=w834) -> ()  [unwired: 2 in, 2 out]
      }
      event "泵滴定数2": Mouse Down {
        n557 = event-data() -> ()  [unwired: 1 in, 8 out]
        n558 = local read "泵滴定数2"() -> (w837:dbl)
        n559 = call "数字键盘.vi"("OldNumber"=w837) -> ("NewNumber"=w836:sgl)
        n560 = property on="泵滴定数2" class="DigNum (严格)"("Val(Sgnl)"=w836) -> ()  [unwired: 2 in, 2 out]
      }
      event "泵滴定数3": Mouse Down {
        n561 = event-data() -> ()  [unwired: 1 in, 8 out]
        n562 = local read "泵滴定数3"() -> (w839:dbl)
        n563 = call "数字键盘.vi"("OldNumber"=w839) -> ("NewNumber"=w838:sgl)
        n564 = property on="泵滴定数3" class="DigNum (严格)"("Val(Sgnl)"=w838) -> ()  [unwired: 2 in, 2 out]
      }
      event "泵滴定数4": Mouse Down {
        n565 = event-data() -> ()  [unwired: 1 in, 8 out]
        n566 = local read "泵滴定数4"() -> (w841:dbl)
        n567 = call "数字键盘.vi"("OldNumber"=w841) -> ("NewNumber"=w840:sgl)
        n568 = property on="泵滴定数4" class="DigNum (严格)"("Val(Sgnl)"=w840) -> ()  [unwired: 2 in, 2 out]
      }
      event "泵滴定数5": Mouse Down {
        n569 = event-data() -> ()  [unwired: 1 in, 8 out]
        n570 = local read "泵滴定数5"() -> (w843:dbl)
        n571 = call "数字键盘.vi"("OldNumber"=w843) -> ("NewNumber"=w842:sgl)
        n572 = property on="泵滴定数5" class="DigNum (严格)"("Val(Sgnl)"=w842) -> ()  [unwired: 2 in, 2 out]
      }
      event "低切高阈值:", "高切低阈值:": Mouse Down {
        n573 = event-data() -> ("CtlRef"=w847:refnum<vi>)  [unwired: 1 in, 7 out]
        n574 = property class="DigNum (严格)"(reference=w847) -> (reference out=w846:refnum<vi>, "Value"=w845:dbl)  [unwired: 1 in, 1 out]
        n575 = call "数字键盘.vi"("OldNumber"=w845) -> ("NewNumber"=w844:sgl)
        n576 = property class="DigNum (严格)"(reference=w846, "Val(Sgnl)"=w844) -> ()  [unwired: 1 in, 2 out]
      }
    }
  }
  n577 = flat-sequence {
    tunnel: [w851] -> w7
    frame #0 {
      n578 = global read "COD读取DATA全局.vi" "序列号:"() -> (w848:string)
      "序列号" <- w848
      n579 = property on="窗格" class="Pane"("Origin"=T17 {"Horizontal"=0, "Vertical"=0} ("原点")) -> ()  [unwired: 2 in, 2 out]
      n580 = Empty String/Path?(string/path=w848) -> (empty?=w850:bool)
      n581 = case shown="真" w850 {
        tunnel: w848 -> [w868 _]
        tunnel: [w867 "data\\Set.ini" ("名称或相对路径")] -> w849
        frame False {
          # "与生产用上位机交互"
          n582 = Concatenate Strings("data\\" ("字符串"), "序列号" ("字符串"), w868, "Set.ini" ("名称或相对路径")) -> (w867:string)
        }
        frame True {
        }
      }
      n583 = call <vilib>:"Application Directory.vi"() -> ("Application Directory"=w860:path)
      n584 = local write "量程切换次数"(u8 0 ("量程切换次数")) -> ()
      n585 = local write "切换量程连续测两次"(FALSE ("切换量程连续测两次")) -> ()
      n586 = Build Path(base path=w860, name or relative path=w849) -> (appended path=w859:path)
      n587 = call <vilib>:"Open Config Data.vi"("configuration file path"=w859) -> ("error out"=w855:errorcluster, "refnum"=w858:T16)  [unwired: 8 in, 1 out]
      n588 = vi-ref "斯坦道CODMn.lvlib:CODMn断电保存全局变量.vi"() -> (w857:refnum<vi>)
      n589 = call <userlib>:"Read Panel from INI__ogtk.vi"("error in (no error)"=w855, "VI ref"=w857, "refnum"=w858) -> ("error out"=w854:errorcluster, "refnum out"=w856:T16)  [unwired: 7 in]
      n590 = call <vilib>:"Close Config Data.vi"("error in (no error)"=w854, "refnum"=w856) -> ("error out"=w853:errorcluster, "file path"=w852:path)  [unwired: 8 in]
      n591 = global write "COD读取DATA全局.vi" "配置文件ini"(w849) -> ()
      n592 = local write "选用水样"(enum16{"葡萄糖", "草酸钠"}."葡萄糖" ("选用水样")) -> ()
      n593 = local write "量程选择"(enum16{"低量程", "高量程", "0-2量程"}."低量程" ("量程选择")) -> ()
      n594 = Open/Create/Replace File(file path (use dialog)=w852, error in=w853) -> (error out=w851:errorcluster)  [unwired: 4 in, 2 out]
      "稀释倍数解释" <- "稀释倍数解释：\n稀释倍数选择1，表示不稀释\n默认低量程系数倍数1，高量程系数倍数2\n则低量程为0~8，高量程为0~16" ("稀释倍数解释")
    }
  }
  n595 = vi-ref "CODMn通讯.vi"() -> (w6:refnum<vi>)
  n596 = property class="VI"(reference=w6) -> ("Name"=w8:string)  [unwired: 1 in, 2 out]
  n597 = Open VI Reference(type specifier VI Refnum (for type only)=refnum<vi> refnum, vi path=w8, options=128 ("选项")) -> (vi reference=w10:refnum<vi>, error out=w12:errorcluster)  [unwired: 3 in]
  n598 = call-by-ref "?"(reference=w10, error in=w12) -> (reference out=w14:refnum<vi>, error out=w13:errorcluster)  [unwired: 12 in]
  n599 = Close Reference(reference=w14, error in (no error)=w13) -> ()  [unwired: 1 out]
  n600 = Obtain Queue(name (unnamed)="CODMn外部交互" ("名称（未命名）"), element data type=T4 {"命令"="启动命令", "测量模式"=enum."水样测量", "CODMn量程切换"=enum."AUTO"} ("元素")) -> (queue out=w2:refnum<queue>, error out=w1:errorcluster)  [unwired: 3 in, 1 out]
  n601 = Obtain Queue(name (unnamed)="CODMn" ("名称（未命名）"), element data type=cluster{"命令":string} {"命令"="启用模块"} ("元素")) -> (queue out=w16:refnum<queue>, error out=w15:errorcluster)  [unwired: 3 in, 1 out]
  n602 = while {
    tunnel: w16 -> [w874]
    tunnel: w15 -> [w873]
    stop <- FALSE stop-if-true
    # "主线事件"
    n603 = event shown="[7] \"常规版/认证版\": 值改变" {
      selector: _ -> [_ _ _ _ _ _ _ _ _ _ _ _ _ _ _ _ _ _ _ _ _ _ _ _ _ _ _ _ _ _ _]
      dyn-events: _ -> [_ _ _ _ _ _ _ _ _ _ _ _ _ _ _ _ _ _ _ _ _ _ _ _ _ _ _ _ _ _ _]
      timeout: _ -> [_ _ _ _ _ _ _ _ _ _ _ _ _ _ _ _ _ _ _ _ _ _ _ _ _ _ _ _ _ _ _]
      tunnel: w874 -> [_ _ _ _ _ w931 _ _ _ _ _ _ _ _ _ _ _ _ _ _ _ _ _ w1524 _ _ _ _ w1742 w1749 _]
      tunnel: w873 -> [_ _ _ _ _ w930 _ _ _ _ _ _ _ _ _ _ _ _ _ _ _ _ _ w1523 _ _ _ _ w1741 w1748 _]
      event "单步启动": Mouse Down {
        n604 = event-data() -> ()  [unwired: 1 in, 8 out]
        n605 = call "CODMn手动控制框.vi"() -> ()  [unwired: 12 in]
      }
      event "启动": Mouse Down {
        n606 = event-data() -> ()  [unwired: 1 in, 8 out]
        n607 = flat-sequence {
          tunnel: [w877] -> w876
          tunnel: w876 -> [w883]
          frame #0 {
            n608 = call "启动测量模式选择对话框.vi"() -> ("启动选择 2"=w877:u16)  [unwired: 11 in]
            "启动选择 2" <- w877
          }
          frame #1 {
            n609 = case shown="9, 默认" w883 {
              tunnel: [u16 4608 ("address") u16 4608 ("address") u16 4608 ("address") u16 4608 ("address") u16 4608 ("address") u16 4608 ("address") u16 4608 ("address") u16 4608 ("address") u16 4608 ("address") u16 4608 ("address")] -> w879
              tunnel: [u16 1 ("address") u16 2 ("address") u16 3 ("address") u16 4 ("address") u16 5 ("address") u16 7 ("address") u16 6 ("address") u16 8 ("address") u16 9 ("address") u16 0 ("address")] -> w884
              frame 0 {
              }
              frame 1 {
              }
              frame 2 {
              }
              frame 3 {
              }
              frame 4 {
              }
              frame 5 {
              }
              frame 6 {
              }
              frame 7 {
              }
              frame 8 {
              }
              frame 9, Default {
              }
            }
            n610 = Not Equal?(x=w883, y=u16 9) -> (x != y?=w881:bool)
            n611 = global write "CODMN外部API.vi" "手动启动CODMn"(w881) -> ()
            n612 = Insert Into Array(array=u16[] [] ("values"), index=0 ("索引"), new element=w884) -> (w878:u16[])
            n613 = call "CODMnMB_api.vi"("STEP"=enum16{"open", "read", "write", "close"}."write", "values"=w878, "starting address"=w879) -> ()  [unwired: 5 in, 4 out]
          }
        }
      }
      event "停止": Value Change {
        n614 = event-data() -> ()  [unwired: 1 in, 6 out]
        n615 = Two Button Dialog(message="确认是否停止？" ("消息"), 1:"否" ("F按钮名称（“取消”）"), 2:"是" ("T按钮名称（“确定”）")) -> (T button?=w909:bool)
        n616 = case shown="真" w909 {
          frame False {
          }
          frame True {
            n617 = call "CODMnMB_api.vi"("STEP"=enum16{"open", "read", "write", "close"}."write", "values"=u16[] [11], "starting address"=u16 4608) -> ()  [unwired: 5 in, 4 out]
          }
        }
      }
      event "手动控制": Value Change {
        n618 = event-data() -> ()  [unwired: 1 in, 6 out]
        n619 = call "数字密码键盘.vi"() -> ("NewNumber"=w914:sgl)  [unwired: 1 in]
        n620 = Equal?(x=w914, y=8.0) -> (x = y?=w915:bool)
        n621 = case shown="假" w915 {
          frame False {
            n622 = call "窗口弹出对话框(子VI).vi"("消息"="密码错误") -> ()  [unwired: 10 in, 1 out]
          }
          frame True {
          }
        }
      }
      event "锁定按钮": Mouse Down {
        n623 = event-data() -> ("CtlRef"=w920:refnum<vi>)  [unwired: 1 in, 7 out]
        n624 = property class="Bool (严格)"(reference=w920) -> ("Value"=w919:bool)  [unwired: 1 in, 2 out]
        n625 = case shown="真" w919 {
          selector: w919 -> [w921 _]
          tunnel: [w921 w922] -> w918
          frame False {
          }
          frame True {
            n626 = call "数字密码键盘.vi"() -> ("NewNumber"=w923:sgl)  [unwired: 1 in]
            n627 = Equal?(x=w923, y=8.0) -> (x = y?=w922:bool)
            n628 = case shown="假" w922 {
              selector: w922 -> [w926 _]
              frame False {
                n629 = One Button Dialog(message="密码错误!" ("消息")) -> ()  [unwired: 1 in, 1 out]
                n630 = local write "锁定按钮"(w926) -> ()
              }
              frame True {
                n631 = One Button Dialog(message="解锁成功!" ("消息")) -> ()  [unwired: 1 in, 1 out]
              }
            }
          }
        }
        "x = y?" <- w918
      }
      event "参数配置": Value Change {
        (unwired) u16 20 ("number of holding registers")
        (unwired) u16 4272 ("starting address")
        n632 = event-data() -> ()  [unwired: 1 in, 6 out]
        n633 = property on="窗格" class="Pane"("Origin"=T17 {"Horizontal"=0, "Vertical"=650} ("原点")) -> ()  [unwired: 2 in, 2 out]
        n634 = Bundle By Name(cluster=cluster{"命令":string} {"命令"=""} ("元素"), "命令"="CODMn读取参数" ("名称（未命名）")) -> (w932:cluster{"命令":string})
        n635 = Enqueue Element(queue=w931, element=w932, error in (no error)=w930) -> ()  [unwired: 1 in, 3 out]
        n636 = global read "COD读取DATA全局.vi" "配置文件ini"() -> (w928:string)
        n637 = call <vilib>:"Application Directory.vi"() -> ("Application Directory"=w935:path)
        n638 = Build Path(base path=w935, name or relative path=w928) -> (appended path=w936:path)
        n639 = call <vilib>:"Open Config Data.vi"("configuration file path"=w936) -> ("error out"=w940:errorcluster, "refnum"=w937:T16)  [unwired: 8 in, 1 out]
        n640 = vi-ref "斯坦道CODMn.lvlib:CODMn断电保存全局变量.vi"() -> (w938:refnum<vi>)
        n641 = call <userlib>:"Read Panel from INI__ogtk.vi"("error in (no error)"=w940, "VI ref"=w938, "refnum"=w937) -> ("error out"=w941:errorcluster, "refnum out"=w939:T16)  [unwired: 7 in]
        n642 = call <vilib>:"Close Config Data.vi"("error in (no error)"=w941, "refnum"=w939) -> ("error out"=w942:errorcluster, "file path"=w943:path)  [unwired: 8 in]
        n643 = Open/Create/Replace File(file path (use dialog)=w943, error in=w942) -> (error out=w929:errorcluster)  [unwired: 4 in, 2 out]
        n644 = call <vilib>:"Clear Errors.vi"("error in (no error)"=w929) -> ()  [unwired: 5 in, 2 out]
      }
      event "保存": Mouse Down {
        n645 = event-data() -> ()  [unwired: 1 in, 8 out]
        n646 = call "CODMnMB_api.vi"("STEP"=enum16{"open", "read", "write", "close"}."write", "values"="保存参数", "starting address"=u16 4272) -> ("error out"=w951:errorcluster)  [unwired: 5 in, 3 out]
        n647 = Build Array("采水泵进样时间/s:", "采水泵润洗时间/s:", "采水泵沉淀时间/s:", "采水泵排液时间/s:") -> (w945:i32[])
        n648 = call "CODMnMB_api.vi"("STEP"=enum16{"open", "read", "write", "close"}."write", "Error in"=w951, "values"=w945, "starting address"=u16 5596) -> ()  [unwired: 4 in, 4 out]
      }
      event "常规版/认证版": Value Change {
        n649 = event-data() -> ()  [unwired: 1 in, 6 out]
        n650 = flat-sequence {
          frame #0 {
            n651 = global write "CODMn断电保存全局变量.vi" "常规版/认证版"("常规版/认证版") -> ()
          }
          frame #1 {
            n652 = global read "COD读取DATA全局.vi" "配置文件ini"() -> (w957:string)
            n653 = call <vilib>:"Application Directory.vi"() -> ("Application Directory"=w970:path)
            n654 = Build Path(base path=w970, name or relative path=w957) -> (appended path=w969:path)
            n655 = call <vilib>:"Open Config Data.vi"("configuration file path"=w969) -> ("error out"=w965:errorcluster, "refnum"=w968:T16)  [unwired: 8 in, 1 out]
            n656 = vi-ref "斯坦道CODMn.lvlib:CODMn断电保存全局变量.vi"() -> (w967:refnum<vi>)
            n657 = call <userlib>:"Write Panel to INI__ogtk.vi"("error in (no error)"=w965, "VI ref"=w967, "refnum"=w968) -> ("error out"=w964:errorcluster, "refnum out"=w966:T16)  [unwired: 7 in]
            n658 = call <vilib>:"Close Config Data.vi"("error in (no error)"=w964, "refnum"=w966) -> ("error out"=w959:errorcluster, "file path"=w958:path)  [unwired: 8 in]
            n659 = Open/Create/Replace File(file path (use dialog)=w958, error in=w959) -> (refnum out=w962:refnum<file>, error out=w963:errorcluster)  [unwired: 4 in, 1 out]
            n660 = Flush File(refnum=w962, error in=w963) -> (refnum out=w961:refnum<file>, error out=w960:errorcluster)
            n661 = Close File(refnum=w961, error in=w960) -> ()  [unwired: 2 out]
          }
        }
      }
      event "校准配置": Value Change {
        n662 = event-data() -> ()  [unwired: 1 in, 6 out]
        n663 = property on="窗格" class="Pane"("Origin"=T17 {"Horizontal"=0, "Vertical"=1300} ("原点")) -> ()  [unwired: 2 in, 2 out]
        n664 = global read "COD读取DATA全局.vi" "配置文件ini"() -> (w971:string)
        n665 = call <vilib>:"Application Directory.vi"() -> ("Application Directory"=w1021:path)
        n666 = Build Path(base path=w1021, name or relative path=w971) -> (appended path=w1020:path)
        n667 = call <vilib>:"Open Config Data.vi"("configuration file path"=w1020) -> ("error out"=w990:errorcluster, "refnum"=w991:T16)  [unwired: 8 in, 1 out]
        n668 = local read "量程选择"() -> (w997:enum16{"低量程", "高量程", "0-2量程"})
        n669 = call-poly <vilib>:"Read Key.vi"("section"="CODMn模型选择" ("key"), "error in (no error)"=w990, "key"="线性和多项式", "refnum"=w991) -> ("error out"=w987:errorcluster, "value"=w989:i32, "refnum out"=w988:T16)  [unwired: 4 in, 1 out]
        n670 = case shown="\"0-2量程\"" w997 {
          tunnel: ["低量程" "高量程" "0-2量程"] -> w995
          frame "低量程", Default {
          }
          frame "高量程" {
          }
          frame "0-2量程" {
          }
        }
        n671 = local write "模型"(w989) -> ()
        n672 = call-poly <vilib>:"Read Key.vi"("section"="标线选择", "error in (no error)"=w987, "key"="选用水样", "refnum"=w988) -> ("error out"=w985:errorcluster, "value"=w972:i32, "refnum out"=w986:T16)  [unwired: 4 in, 1 out]
        n673 = case shown="0, 默认" w972 {
          tunnel: ["葡萄糖标线" ("section") "草酸钠标线" ("section")] -> w996
          frame 0, Default {
          }
          frame 1 {
          }
        }
        n674 = local write "选用水样"(w972) -> ()
        n675 = Concatenate Strings(w996, w995) -> (w994:string)
        n676 = call-poly <vilib>:"Read Key.vi"("section"=w994, "error in (no error)"=w985, "key"="浓度1", "refnum"=w986) -> ("error out"=w1025:errorcluster, "value"=w1023:dbl, "refnum out"=w1024:T16)  [unwired: 4 in, 1 out]
        n677 = local write "浓度1"(w1023) -> ()
        n678 = call-poly <vilib>:"Read Key.vi"("section"=w994, "error in (no error)"=w1025, "key"="浓度2", "refnum"=w1024) -> ("error out"=w1039:errorcluster, "value"=w1026:dbl, "refnum out"=w1038:T16)  [unwired: 4 in, 1 out]
        n679 = local write "浓度2"(w1026) -> ()
        n680 = call-poly <vilib>:"Read Key.vi"("section"=w994, "error in (no error)"=w1039, "key"="浓度3", "refnum"=w1038) -> ("error out"=w1040:errorcluster, "value"=w1028:dbl, "refnum out"=w1037:T16)  [unwired: 4 in, 1 out]
        n681 = local write "浓度3"(w1028) -> ()
        n682 = call-poly <vilib>:"Read Key.vi"("section"=w994, "error in (no error)"=w1040, "key"="泵滴定数1", "refnum"=w1037) -> ("error out"=w1041:errorcluster, "value"=w1030:dbl, "refnum out"=w1036:T16)  [unwired: 4 in, 1 out]
        n683 = local write "泵滴定数1"(w1030) -> ()
        n684 = call-poly <vilib>:"Read Key.vi"("section"=w994, "error in (no error)"=w1041, "key"="泵滴定数2", "refnum"=w1036) -> ("error out"=w1035:errorcluster, "value"=w1033:dbl, "refnum out"=w1042:T16)  [unwired: 4 in, 1 out]
        n685 = local write "泵滴定数2"(w1033) -> ()
        n686 = call-poly <vilib>:"Read Key.vi"("section"=w994, "error in (no error)"=w1035, "key"="泵滴定数3", "refnum"=w1042) -> ("error out"=w1047:errorcluster, "value"=w1046:dbl, "refnum out"=w1043:T16)  [unwired: 4 in, 1 out]
        n687 = local write "泵滴定数3"(w1046) -> ()
        n688 = call-poly <vilib>:"Read Key.vi"("section"=w994, "error in (no error)"=w1047, "key"="浓度4", "refnum"=w1043) -> ("error out"=w1048:errorcluster, "value"=w978:dbl, "refnum out"=w1044:T16)  [unwired: 4 in, 1 out]
        n689 = local write "浓度4"(w978) -> ()
        n690 = call-poly <vilib>:"Read Key.vi"("section"=w994, "error in (no error)"=w1048, "key"="浓度5", "refnum"=w1044) -> ("error out"=w983:errorcluster, "value"=w977:dbl, "refnum out"=w984:T16)  [unwired: 4 in, 1 out]
        n691 = local write "浓度5"(w977) -> ()
        n692 = call-poly <vilib>:"Read Key.vi"("section"=w994, "error in (no error)"=w983, "key"="泵滴定数4", "refnum"=w984) -> ("error out"=w1049:errorcluster, "value"=w976:dbl, "refnum out"=w1045:T16)  [unwired: 4 in, 1 out]
        n693 = local write "泵滴定数4"(w976) -> ()
        n694 = call-poly <vilib>:"Read Key.vi"("section"=w994, "error in (no error)"=w1049, "key"="泵滴定数5", "refnum"=w1045) -> ("error out"=w981:errorcluster, "value"=w975:dbl, "refnum out"=w982:T16)  [unwired: 4 in, 1 out]
        n695 = local write "泵滴定数5"(w975) -> ()
        n696 = call-poly <vilib>:"Read Key.vi"("section"=w994, "error in (no error)"=w981, "key"="当前选用的校准", "refnum"=w982) -> ("error out"=w1016:errorcluster, "value"=w1018:i32, "refnum out"=w1017:T16)  [unwired: 4 in, 1 out]
        n697 = local write "当前校准"(w1018) -> ()
        n698 = call-poly <vilib>:"Read Key.vi"("section"=w994, "error in (no error)"=w1016, "key"="启用1", "refnum"=w1017) -> ("error out"=w1013:errorcluster, "value"=w1002:bool, "refnum out"=w1014:T16)  [unwired: 4 in, 1 out]
        n699 = local write "启用1"(w1002) -> ()
        n700 = call-poly <vilib>:"Read Key.vi"("section"=w994, "error in (no error)"=w1013, "key"="启用2", "refnum"=w1014) -> ("error out"=w1011:errorcluster, "value"=w1001:bool, "refnum out"=w1012:T16)  [unwired: 4 in, 1 out]
        n701 = local write "启用2"(w1001) -> ()
        n702 = call-poly <vilib>:"Read Key.vi"("section"=w994, "error in (no error)"=w1011, "key"="启用3", "refnum"=w1012) -> ("error out"=w1009:errorcluster, "value"=w1000:bool, "refnum out"=w1010:T16)  [unwired: 4 in, 1 out]
        n703 = local write "启用3"(w1000) -> ()
        n704 = call-poly <vilib>:"Read Key.vi"("section"=w994, "error in (no error)"=w1009, "key"="启用4", "refnum"=w1010) -> ("error out"=w1007:errorcluster, "value"=w974:bool, "refnum out"=w1008:T16)  [unwired: 4 in, 1 out]
        n705 = local write "启用4"(w974) -> ()
        n706 = call-poly <vilib>:"Read Key.vi"("section"=w994, "error in (no error)"=w1007, "key"="启用5", "refnum"=w1008) -> ("error out"=w979:errorcluster, "value"=w973:bool, "refnum out"=w980:T16)  [unwired: 4 in, 1 out]
        n707 = local write "启用5"(w973) -> ()
        n708 = call <vilib>:"Close Config Data.vi"("error in (no error)"=w979, "refnum"=w980) -> ()  [unwired: 8 in, 2 out]
      }
      event "选用水样": Value Change {
        (unwired) "浓度6" ("key")
        n709 = event-data() -> ()  [unwired: 1 in, 6 out]
        n710 = property on="窗格" class="Pane"("Origin"=T17 {"Horizontal"=0, "Vertical"=1300} ("原点")) -> ()  [unwired: 2 in, 2 out]
        n711 = local read "量程选择"() -> (w1074:enum16{"低量程", "高量程", "0-2量程"})
        n712 = global read "COD读取DATA全局.vi" "配置文件ini"() -> (w1060:string)
        n713 = case shown="\"0-2量程\"" w1074 {
          tunnel: ["低量程" "高量程" "0-2量程"] -> w1075
          frame "低量程", Default {
          }
          frame "高量程" {
          }
          frame "0-2量程" {
          }
        }
        n714 = case shown="\"葡萄糖\", 默认" "选用水样" {
          tunnel: ["葡萄糖标线" ("section") "草酸钠标线" ("section")] -> w1076
          frame "葡萄糖", Default {
          }
          frame "草酸钠" {
          }
        }
        n715 = call <vilib>:"Application Directory.vi"() -> ("Application Directory"=w1099:path)
        n716 = Build Path(base path=w1099, name or relative path=w1060) -> (appended path=w1098:path)
        n717 = call <vilib>:"Open Config Data.vi"("configuration file path"=w1098) -> ("error out"=w1100:errorcluster, "refnum"=w1101:T16)  [unwired: 8 in, 1 out]
        n718 = Concatenate Strings(w1076, w1075) -> (w1073:string)
        n719 = call-poly <vilib>:"Read Key.vi"("section"=w1073, "error in (no error)"=w1100, "key"="浓度1", "refnum"=w1101) -> ("error out"=w1105:errorcluster, "value"=w1103:dbl, "refnum out"=w1104:T16)  [unwired: 4 in, 1 out]
        n720 = local write "浓度1"(w1103) -> ()
        n721 = call-poly <vilib>:"Read Key.vi"("section"=w1073, "error in (no error)"=w1105, "key"="浓度2", "refnum"=w1104) -> ("error out"=w1119:errorcluster, "value"=w1106:dbl, "refnum out"=w1118:T16)  [unwired: 4 in, 1 out]
        n722 = local write "浓度2"(w1106) -> ()
        n723 = call-poly <vilib>:"Read Key.vi"("section"=w1073, "error in (no error)"=w1119, "key"="浓度3", "refnum"=w1118) -> ("error out"=w1120:errorcluster, "value"=w1108:dbl, "refnum out"=w1117:T16)  [unwired: 4 in, 1 out]
        n724 = local write "浓度3"(w1108) -> ()
        n725 = call-poly <vilib>:"Read Key.vi"("section"=w1073, "error in (no error)"=w1120, "key"="泵滴定数1", "refnum"=w1117) -> ("error out"=w1121:errorcluster, "value"=w1110:dbl, "refnum out"=w1116:T16)  [unwired: 4 in, 1 out]
        n726 = local write "泵滴定数1"(w1110) -> ()
        n727 = call-poly <vilib>:"Read Key.vi"("section"=w1073, "error in (no error)"=w1121, "key"="泵滴定数2", "refnum"=w1116) -> ("error out"=w1115:errorcluster, "value"=w1113:dbl, "refnum out"=w1122:T16)  [unwired: 4 in, 1 out]
        n728 = local write "泵滴定数2"(w1113) -> ()
        n729 = call-poly <vilib>:"Read Key.vi"("section"=w1073, "error in (no error)"=w1115, "key"="泵滴定数3", "refnum"=w1122) -> ("error out"=w1127:errorcluster, "value"=w1126:dbl, "refnum out"=w1123:T16)  [unwired: 4 in, 1 out]
        n730 = local write "泵滴定数3"(w1126) -> ()
        n731 = call-poly <vilib>:"Read Key.vi"("section"=w1073, "error in (no error)"=w1127, "key"="浓度4", "refnum"=w1123) -> ("error out"=w1128:errorcluster, "value"=w1068:dbl, "refnum out"=w1124:T16)  [unwired: 4 in, 1 out]
        n732 = local write "浓度4"(w1068) -> ()
        n733 = call-poly <vilib>:"Read Key.vi"("section"=w1073, "error in (no error)"=w1128, "key"="浓度5", "refnum"=w1124) -> ("error out"=w1071:errorcluster, "value"=w1067:dbl, "refnum out"=w1072:T16)  [unwired: 4 in, 1 out]
        n734 = local write "浓度5"(w1067) -> ()
        n735 = call-poly <vilib>:"Read Key.vi"("section"=w1073, "error in (no error)"=w1071, "key"="泵滴定数4", "refnum"=w1072) -> ("error out"=w1129:errorcluster, "value"=w1066:dbl, "refnum out"=w1125:T16)  [unwired: 4 in, 1 out]
        n736 = local write "泵滴定数4"(w1066) -> ()
        n737 = call-poly <vilib>:"Read Key.vi"("section"=w1073, "error in (no error)"=w1129, "key"="泵滴定数5", "refnum"=w1125) -> ("error out"=w1069:errorcluster, "value"=w1065:dbl, "refnum out"=w1070:T16)  [unwired: 4 in, 1 out]
        n738 = local write "泵滴定数5"(w1065) -> ()
        n739 = call-poly <vilib>:"Read Key.vi"("section"=w1073, "error in (no error)"=w1069, "key"="当前选用的校准", "refnum"=w1070) -> ("error out"=w1094:errorcluster, "value"=w1096:i32, "refnum out"=w1095:T16)  [unwired: 4 in, 1 out]
        n740 = call-poly <vilib>:"Read Key.vi"("section"=w1073, "error in (no error)"=w1094, "key"="启用1", "refnum"=w1095) -> ("error out"=w1091:errorcluster, "value"=w1080:bool, "refnum out"=w1092:T16)  [unwired: 4 in, 1 out]
        n741 = local write "当前校准"(w1096) -> ()
        n742 = local write "启用1"(w1080) -> ()
        n743 = call-poly <vilib>:"Read Key.vi"("section"=w1073, "error in (no error)"=w1091, "key"="启用2", "refnum"=w1092) -> ("error out"=w1089:errorcluster, "value"=w1079:bool, "refnum out"=w1090:T16)  [unwired: 4 in, 1 out]
        n744 = local write "启用2"(w1079) -> ()
        n745 = call-poly <vilib>:"Read Key.vi"("section"=w1073, "error in (no error)"=w1089, "key"="启用3", "refnum"=w1090) -> ("error out"=w1087:errorcluster, "value"=w1078:bool, "refnum out"=w1088:T16)  [unwired: 4 in, 1 out]
        n746 = local write "启用3"(w1078) -> ()
        n747 = call-poly <vilib>:"Read Key.vi"("section"=w1073, "error in (no error)"=w1087, "key"="启用4", "refnum"=w1088) -> ("error out"=w1085:errorcluster, "value"=w1062:bool, "refnum out"=w1086:T16)  [unwired: 4 in, 1 out]
        n748 = local write "启用4"(w1062) -> ()
        n749 = call-poly <vilib>:"Read Key.vi"("section"=w1073, "error in (no error)"=w1085, "key"="启用5", "refnum"=w1086) -> ("error out"=w1063:errorcluster, "value"=w1061:bool, "refnum out"=w1064:T16)  [unwired: 4 in, 1 out]
        n750 = local write "启用5"(w1061) -> ()
        n751 = call <vilib>:"Close Config Data.vi"("error in (no error)"=w1063, "refnum"=w1064) -> ()  [unwired: 8 in, 2 out]
      }
      event "量程选择": Value Change {
        n752 = event-data() -> ()  [unwired: 1 in, 6 out]
        n753 = local read "选用水样"() -> (w1157:enum16{"葡萄糖", "草酸钠"})
        n754 = global read "COD读取DATA全局.vi" "配置文件ini"() -> (w1140:string)
        n755 = property on="窗格" class="Pane"("Origin"=T17 {"Horizontal"=0, "Vertical"=1300} ("原点")) -> ()  [unwired: 2 in, 2 out]
        n756 = case shown="\"葡萄糖\", 默认" w1157 {
          tunnel: ["葡萄糖标线" ("section") "草酸钠标线" ("section")] -> w1156
          frame "葡萄糖", Default {
          }
          frame "草酸钠" {
          }
        }
        n757 = case shown="\"0-2量程\"" "量程选择" {
          tunnel: ["低量程" "高量程" "0-2量程"] -> w1153
          frame "低量程", Default {
          }
          frame "高量程" {
          }
          frame "0-2量程" {
          }
        }
        n758 = call <vilib>:"Application Directory.vi"() -> ("Application Directory"=w1179:path)
        n759 = Build Path(base path=w1179, name or relative path=w1140) -> (appended path=w1178:path)
        n760 = call <vilib>:"Open Config Data.vi"("configuration file path"=w1178) -> ("error out"=w1180:errorcluster, "refnum"=w1181:T16)  [unwired: 8 in, 1 out]
        n761 = Concatenate Strings(w1156, w1153) -> (w1155:string)
        n762 = call-poly <vilib>:"Read Key.vi"("section"=w1155, "error in (no error)"=w1180, "key"="浓度1", "refnum"=w1181) -> ("error out"=w1185:errorcluster, "value"=w1183:dbl, "refnum out"=w1184:T16)  [unwired: 4 in, 1 out]
        n763 = local write "浓度1"(w1183) -> ()
        n764 = call-poly <vilib>:"Read Key.vi"("section"=w1155, "error in (no error)"=w1185, "key"="浓度2", "refnum"=w1184) -> ("error out"=w1199:errorcluster, "value"=w1186:dbl, "refnum out"=w1198:T16)  [unwired: 4 in, 1 out]
        n765 = local write "浓度2"(w1186) -> ()
        n766 = call-poly <vilib>:"Read Key.vi"("section"=w1155, "error in (no error)"=w1199, "key"="浓度3", "refnum"=w1198) -> ("error out"=w1200:errorcluster, "value"=w1188:dbl, "refnum out"=w1197:T16)  [unwired: 4 in, 1 out]
        n767 = local write "浓度3"(w1188) -> ()
        n768 = call-poly <vilib>:"Read Key.vi"("section"=w1155, "error in (no error)"=w1200, "key"="泵滴定数1", "refnum"=w1197) -> ("error out"=w1201:errorcluster, "value"=w1190:dbl, "refnum out"=w1196:T16)  [unwired: 4 in, 1 out]
        n769 = local write "泵滴定数1"(w1190) -> ()
        n770 = call-poly <vilib>:"Read Key.vi"("section"=w1155, "error in (no error)"=w1201, "key"="泵滴定数2", "refnum"=w1196) -> ("error out"=w1195:errorcluster, "value"=w1193:dbl, "refnum out"=w1202:T16)  [unwired: 4 in, 1 out]
        n771 = local write "泵滴定数2"(w1193) -> ()
        n772 = call-poly <vilib>:"Read Key.vi"("section"=w1155, "error in (no error)"=w1195, "key"="泵滴定数3", "refnum"=w1202) -> ("error out"=w1207:errorcluster, "value"=w1206:dbl, "refnum out"=w1203:T16)  [unwired: 4 in, 1 out]
        n773 = local write "泵滴定数3"(w1206) -> ()
        n774 = call-poly <vilib>:"Read Key.vi"("section"=w1155, "error in (no error)"=w1207, "key"="浓度4", "refnum"=w1203) -> ("error out"=w1208:errorcluster, "value"=w1144:dbl, "refnum out"=w1204:T16)  [unwired: 4 in, 1 out]
        n775 = local write "浓度4"(w1144) -> ()
        n776 = call-poly <vilib>:"Read Key.vi"("section"=w1155, "error in (no error)"=w1208, "key"="浓度5", "refnum"=w1204) -> ("error out"=w1151:errorcluster, "value"=w1143:dbl, "refnum out"=w1152:T16)  [unwired: 4 in, 1 out]
        n777 = local write "浓度5"(w1143) -> ()
        n778 = call-poly <vilib>:"Read Key.vi"("section"=w1155, "error in (no error)"=w1151, "key"="泵滴定数4", "refnum"=w1152) -> ("error out"=w1209:errorcluster, "value"=w1142:dbl, "refnum out"=w1205:T16)  [unwired: 4 in, 1 out]
        n779 = local write "泵滴定数4"(w1142) -> ()
        n780 = call-poly <vilib>:"Read Key.vi"("section"=w1155, "error in (no error)"=w1209, "key"="泵滴定数5", "refnum"=w1205) -> ("error out"=w1149:errorcluster, "value"=w1141:dbl, "refnum out"=w1150:T16)  [unwired: 4 in, 1 out]
        n781 = local write "泵滴定数5"(w1141) -> ()
        n782 = call-poly <vilib>:"Read Key.vi"("section"=w1155, "error in (no error)"=w1149, "key"="当前选用的校准", "refnum"=w1150) -> ("error out"=w1174:errorcluster, "value"=w1176:i32, "refnum out"=w1175:T16)  [unwired: 4 in, 1 out]
        n783 = local write "当前校准"(w1176) -> ()
        n784 = call-poly <vilib>:"Read Key.vi"("section"=w1155, "error in (no error)"=w1174, "key"="启用1", "refnum"=w1175) -> ("error out"=w1171:errorcluster, "value"=w1160:bool, "refnum out"=w1172:T16)  [unwired: 4 in, 1 out]
        n785 = local write "启用1"(w1160) -> ()
        n786 = call-poly <vilib>:"Read Key.vi"("section"=w1155, "error in (no error)"=w1171, "key"="启用2", "refnum"=w1172) -> ("error out"=w1169:errorcluster, "value"=w1159:bool, "refnum out"=w1170:T16)  [unwired: 4 in, 1 out]
        n787 = local write "启用2"(w1159) -> ()
        n788 = call-poly <vilib>:"Read Key.vi"("section"=w1155, "error in (no error)"=w1169, "key"="启用3", "refnum"=w1170) -> ("error out"=w1167:errorcluster, "value"=w1158:bool, "refnum out"=w1168:T16)  [unwired: 4 in, 1 out]
        n789 = local write "启用3"(w1158) -> ()
        n790 = call-poly <vilib>:"Read Key.vi"("section"=w1155, "error in (no error)"=w1167, "key"="启用4", "refnum"=w1168) -> ("error out"=w1165:errorcluster, "value"=w1146:bool, "refnum out"=w1166:T16)  [unwired: 4 in, 1 out]
        n791 = local write "启用4"(w1146) -> ()
        n792 = call-poly <vilib>:"Read Key.vi"("section"=w1155, "error in (no error)"=w1165, "key"="启用5", "refnum"=w1166) -> ("error out"=w1147:errorcluster, "value"=w1145:bool, "refnum out"=w1148:T16)  [unwired: 4 in, 1 out]
        n793 = local write "启用5"(w1145) -> ()
        n794 = call <vilib>:"Close Config Data.vi"("error in (no error)"=w1147, "refnum"=w1148) -> ()  [unwired: 8 in, 2 out]
      }
      event "返回": Value Change {
        w1234 = "CODMn" ("section")
        n795 = event-data() -> ()  [unwired: 1 in, 6 out]
        n796 = global read "COD读取DATA全局.vi" "配置文件ini"() -> (w1220:string)
        n797 = property on="窗格" class="Pane"("Origin"=T17 {"Horizontal"=0, "Vertical"=0} ("原点")) -> ()  [unwired: 2 in, 2 out]
        n798 = call <vilib>:"Application Directory.vi"() -> ("Application Directory"=w1286:path)
        n799 = Build Path(base path=w1286, name or relative path=w1220) -> (appended path=w1285:path)
        n800 = local read "浓度1"() -> (w1281:dbl)
        n801 = call <vilib>:"Open Config Data.vi"("configuration file path"=w1285) -> ("error out"=w1283:errorcluster, "refnum"=w1284:T16)  [unwired: 8 in, 1 out]
        n802 = local read "浓度2"() -> (w1265:dbl)
        n803 = call-poly <vilib>:"Write Key.vi"("section"=w1234, "error in (no error)"=w1283, "value"=w1281, "key"="浓度1", "refnum"=w1284) -> ("error out"=w1280:errorcluster, "refnum out"=w1279:T16)  [unwired: 4 in, 1 out]
        n804 = local read "浓度3"() -> (w1261:dbl)
        n805 = call-poly <vilib>:"Write Key.vi"("section"=w1234, "error in (no error)"=w1280, "value"=w1265, "key"="浓度2", "refnum"=w1279) -> ("error out"=w1278:errorcluster, "refnum out"=w1277:T16)  [unwired: 4 in, 1 out]
        n806 = local read "泵滴定数1"() -> (w1259:dbl)
        n807 = call-poly <vilib>:"Write Key.vi"("section"=w1234, "error in (no error)"=w1278, "value"=w1261, "key"="浓度3", "refnum"=w1277) -> ("error out"=w1276:errorcluster, "refnum out"=w1275:T16)  [unwired: 4 in, 1 out]
        n808 = call-poly <vilib>:"Write Key.vi"("section"=w1234, "error in (no error)"=w1276, "value"=w1259, "key"="泵滴定数1", "refnum"=w1275) -> ("error out"=w1274:errorcluster, "refnum out"=w1273:T16)  [unwired: 4 in, 1 out]
        n809 = local read "泵滴定数2"() -> (w1257:dbl)
        n810 = call-poly <vilib>:"Write Key.vi"("section"=w1234, "error in (no error)"=w1274, "value"=w1257, "key"="泵滴定数2", "refnum"=w1273) -> ("error out"=w1272:errorcluster, "refnum out"=w1271:T16)  [unwired: 4 in, 1 out]
        n811 = local read "泵滴定数3"() -> (w1255:dbl)
        n812 = local read "浓度4"() -> (w1222:dbl)
        n813 = call-poly <vilib>:"Write Key.vi"("section"=w1234, "error in (no error)"=w1272, "value"=w1255, "key"="泵滴定数3", "refnum"=w1271) -> ("error out"=w1270:errorcluster, "refnum out"=w1269:T16)  [unwired: 4 in, 1 out]
        n814 = call-poly <vilib>:"Write Key.vi"("section"=w1234, "error in (no error)"=w1270, "value"=w1222, "key"="浓度4", "refnum"=w1269) -> ("error out"=w1263:errorcluster, "refnum out"=w1264:T16)  [unwired: 4 in, 1 out]
        n815 = local read "浓度5"() -> (w1221:dbl)
        n816 = call-poly <vilib>:"Write Key.vi"("section"=w1234, "error in (no error)"=w1263, "value"=w1221, "key"="浓度5", "refnum"=w1264) -> ("error out"=w1231:errorcluster, "refnum out"=w1232:T16)  [unwired: 4 in, 1 out]
        n817 = local read "泵滴定数4"() -> (w1223:dbl)
        n818 = call-poly <vilib>:"Write Key.vi"("section"=w1234, "error in (no error)"=w1231, "value"=w1223, "key"="泵滴定数4", "refnum"=w1232) -> ("error out"=w1268:errorcluster, "refnum out"=w1267:T16)  [unwired: 4 in, 1 out]
        n819 = local read "泵滴定数5"() -> (w1224:dbl)
        n820 = call-poly <vilib>:"Write Key.vi"("section"=w1234, "error in (no error)"=w1268, "value"=w1224, "key"="泵滴定数5", "refnum"=w1267) -> ("error out"=w1229:errorcluster, "refnum out"=w1230:T16)  [unwired: 4 in, 1 out]
        n821 = local read "启用1"() -> (w1243:bool)
        n822 = call-poly <vilib>:"Write Key.vi"("section"=w1234, "error in (no error)"=w1229, "value"=w1243, "key"="启用1", "refnum"=w1230) -> ("error out"=w1239:errorcluster, "refnum out"=w1242:T16)  [unwired: 4 in, 1 out]
        n823 = local read "启用2"() -> (w1240:bool)
        n824 = call-poly <vilib>:"Write Key.vi"("section"=w1234, "error in (no error)"=w1239, "value"=w1240, "key"="启用2", "refnum"=w1242) -> ("error out"=w1250:errorcluster, "refnum out"=w1249:T16)  [unwired: 4 in, 1 out]
        n825 = local read "启用3"() -> (w1238:bool)
        n826 = call-poly <vilib>:"Write Key.vi"("section"=w1234, "error in (no error)"=w1250, "value"=w1238, "key"="启用3", "refnum"=w1249) -> ("error out"=w1248:errorcluster, "refnum out"=w1247:T16)  [unwired: 4 in, 1 out]
        n827 = local read "启用4"() -> (w1226:bool)
        n828 = call-poly <vilib>:"Write Key.vi"("section"=w1234, "error in (no error)"=w1248, "value"=w1226, "key"="启用4", "refnum"=w1247) -> ("error out"=w1246:errorcluster, "refnum out"=w1245:T16)  [unwired: 4 in, 1 out]
        n829 = local read "启用5"() -> (w1225:bool)
        n830 = call-poly <vilib>:"Write Key.vi"("section"=w1234, "error in (no error)"=w1246, "value"=w1225, "key"="启用5", "refnum"=w1245) -> ("error out"=w1227:errorcluster, "refnum out"=w1228:T16)  [unwired: 4 in, 1 out]
        n831 = call <vilib>:"Close Config Data.vi"("error in (no error)"=w1227, "refnum"=w1228) -> ()  [unwired: 8 in, 2 out]
      }
      event "关闭", "关闭 2", "关闭 3": Value Change {
        n832 = event-data() -> ()  [unwired: 1 in, 6 out]
        n833 = property on="窗格" class="Pane"("Origin"=T17 {"Horizontal"=0, "Vertical"=0} ("原点")) -> ()  [unwired: 2 in, 2 out]
      }
      event Application Instance Close {
        n834 = event-data() -> ()  [unwired: 1 in, 4 out]
      }
      event "时间校准": Value Change {
        n835 = event-data() -> ()  [unwired: 1 in, 6 out]
        n836 = Get Date/Time In Seconds() -> (seconds since 1Jan1904=w1296:timestamp)
        n837 = Build Array(w1296) -> (w1295:timestamp[])
        n838 = call "DateToHex.vi"("DATE"=w1295) -> ("数组"=w1293:u16[])  [unwired: 10 in]
        n839 = Insert Into Array(array=u16[] [1] ("values"), index=1 ("索引"), new element=w1293) -> (w1289:u16[])
        n840 = call "CODMnMB_api.vi"("STEP"=enum16{"open", "read", "write", "close"}."write", "values"=w1289, "starting address"=u16 4612) -> ("error out"=w1288:errorcluster)  [unwired: 5 in, 3 out]
        n841 = call <vilib>:"Clear Errors.vi"("error in (no error)"=w1288) -> ()  [unwired: 5 in, 2 out]
      }
      event "故障清除": Value Change {
        n842 = event-data() -> ()  [unwired: 1 in, 6 out]
        n843 = call "CODMnMB_api.vi"("STEP"=enum16{"open", "read", "write", "close"}."write", "values"=u16[] [1], "starting address"=u16 4611) -> ()  [unwired: 5 in, 4 out]
      }
      event "定时启动": Mouse Down {
        n844 = event-data() -> ()  [unwired: 1 in, 8 out]
        n845 = flat-sequence {
          frame #0 {
            n846 = global read "CODMn断电保存全局变量.vi" "定时控制"() -> (w1301:T10)
            n847 = call "周期设置.vi"("定时控制参数输入"=w1301) -> ("定时控制参数输出"=w1300:T10)  [unwired: 10 in]
            n848 = global write "CODMn断电保存全局变量.vi" "定时控制"(w1300) -> ()
          }
          frame #1 {
            n849 = global read "COD读取DATA全局.vi" "配置文件ini"() -> (w1302:string)
            n850 = call <vilib>:"Application Directory.vi"() -> ("Application Directory"=w1315:path)
            n851 = Build Path(base path=w1315, name or relative path=w1302) -> (appended path=w1314:path)
            n852 = call <vilib>:"Open Config Data.vi"("configuration file path"=w1314) -> ("error out"=w1310:errorcluster, "refnum"=w1313:T16)  [unwired: 8 in, 1 out]
            n853 = vi-ref "斯坦道CODMn.lvlib:CODMn断电保存全局变量.vi"() -> (w1312:refnum<vi>)
            n854 = call <userlib>:"Write Panel to INI__ogtk.vi"("error in (no error)"=w1310, "VI ref"=w1312, "refnum"=w1313) -> ("error out"=w1309:errorcluster, "refnum out"=w1311:T16)  [unwired: 7 in]
            n855 = call <vilib>:"Close Config Data.vi"("error in (no error)"=w1309, "refnum"=w1311) -> ("error out"=w1304:errorcluster, "file path"=w1303:path)  [unwired: 8 in]
            n856 = Open/Create/Replace File(file path (use dialog)=w1303, error in=w1304) -> (refnum out=w1307:refnum<file>, error out=w1308:errorcluster)  [unwired: 4 in, 1 out]
            n857 = Flush File(refnum=w1307, error in=w1308) -> (refnum out=w1306:refnum<file>, error out=w1305:errorcluster)
            n858 = Close File(refnum=w1306, error in=w1305) -> ()  [unwired: 2 out]
          }
        }
      }
      event "测量模式(公式)": Value Change {
        n859 = event-data() -> ()  [unwired: 1 in, 6 out]
        n860 = flat-sequence {
          frame #0 {
            n861 = global write "CODMn断电保存全局变量.vi" "测量模式(公式)"("测量模式(公式)") -> ()
          }
          frame #1 {
            n862 = global read "COD读取DATA全局.vi" "配置文件ini"() -> (w1317:string)
            n863 = call <vilib>:"Application Directory.vi"() -> ("Application Directory"=w1330:path)
            n864 = Build Path(base path=w1330, name or relative path=w1317) -> (appended path=w1329:path)
            n865 = call <vilib>:"Open Config Data.vi"("configuration file path"=w1329) -> ("error out"=w1325:errorcluster, "refnum"=w1328:T16)  [unwired: 8 in, 1 out]
            n866 = vi-ref "斯坦道CODMn.lvlib:CODMn断电保存全局变量.vi"() -> (w1327:refnum<vi>)
            n867 = call <userlib>:"Write Panel to INI__ogtk.vi"("error in (no error)"=w1325, "VI ref"=w1327, "refnum"=w1328) -> ("error out"=w1324:errorcluster, "refnum out"=w1326:T16)  [unwired: 7 in]
            n868 = call <vilib>:"Close Config Data.vi"("error in (no error)"=w1324, "refnum"=w1326) -> ("error out"=w1319:errorcluster, "file path"=w1318:path)  [unwired: 8 in]
            n869 = Open/Create/Replace File(file path (use dialog)=w1318, error in=w1319) -> (refnum out=w1322:refnum<file>, error out=w1323:errorcluster)  [unwired: 4 in, 1 out]
            n870 = Flush File(refnum=w1322, error in=w1323) -> (refnum out=w1321:refnum<file>, error out=w1320:errorcluster)
            n871 = Close File(refnum=w1321, error in=w1320) -> ()  [unwired: 2 out]
          }
        }
      }
      event "跨度量程选择", "跨度液浓度", "零点核查量程选择", "零点核查浓度", "标样浓度", "标样核查量程选择": Value Change {
        n872 = event-data() -> ()  [unwired: 1 in, 6 out]
        n873 = flat-sequence {
          frame #0 {
            n874 = global write "CODMn断电保存全局变量.vi" "标样浓度"("标样浓度") -> ()
            n875 = global write "CODMn断电保存全局变量.vi" "标样核查量程选择"("标样核查量程选择") -> ()
            n876 = global write "CODMn断电保存全局变量.vi" "零点核查浓度"("零点核查浓度") -> ()
            n877 = global write "CODMn断电保存全局变量.vi" "CODMn跨度量程选择"("跨度量程选择") -> ()
            n878 = global write "CODMn断电保存全局变量.vi" "跨度液浓度"("跨度液浓度") -> ()
            n879 = global write "CODMn断电保存全局变量.vi" "零点核查量程选择"("零点核查量程选择") -> ()
          }
          frame #1 {
            n880 = global read "COD读取DATA全局.vi" "配置文件ini"() -> (w1337:string)
            n881 = call <vilib>:"Application Directory.vi"() -> ("Application Directory"=w1350:path)
            n882 = Build Path(base path=w1350, name or relative path=w1337) -> (appended path=w1349:path)
            n883 = call <vilib>:"Open Config Data.vi"("configuration file path"=w1349) -> ("error out"=w1345:errorcluster, "refnum"=w1348:T16)  [unwired: 8 in, 1 out]
            n884 = vi-ref "斯坦道CODMn.lvlib:CODMn断电保存全局变量.vi"() -> (w1347:refnum<vi>)
            n885 = call <userlib>:"Write Panel to INI__ogtk.vi"("error in (no error)"=w1345, "VI ref"=w1347, "refnum"=w1348) -> ("error out"=w1344:errorcluster, "refnum out"=w1346:T16)  [unwired: 7 in]
            n886 = call <vilib>:"Close Config Data.vi"("error in (no error)"=w1344, "refnum"=w1346) -> ("error out"=w1339:errorcluster, "file path"=w1338:path)  [unwired: 8 in]
            n887 = Open/Create/Replace File(file path (use dialog)=w1338, error in=w1339) -> (refnum out=w1342:refnum<file>, error out=w1343:errorcluster)  [unwired: 4 in, 1 out]
            n888 = Flush File(refnum=w1342, error in=w1343) -> (refnum out=w1341:refnum<file>, error out=w1340:errorcluster)
            n889 = Close File(refnum=w1341, error in=w1340) -> ()  [unwired: 2 out]
          }
        }
      }
      event "校准1", "校准2", "校准3", "校准4", "校准5": Value Change {
        n890 = event-data() -> ()  [unwired: 1 in, 6 out]
        n891 = flat-sequence {
          frame #0 {
            n892 = Build Array("校准1", "校准2", "校准3", "校准4", "校准5") -> (w1353:bool[])
            n893 = for {
              tunnel: w1353 -> [w1364] mode=indexing
              i -> [w1357]
              n894 = case shown="4" w1357 {
                tunnel: ["浓度1" "浓度2" "浓度3" "浓度4" "浓度5"] -> w1360
                frame 0, Default {
                }
                frame 1 {
                }
                frame 2 {
                }
                frame 3 {
                }
                frame 4 {
                }
              }
              n895 = Multiply(x=w1360, y=100.0) -> (x*y=w1358:dbl)
              n896 = Insert Into Array(array=u16[] [] ("values"), index=0 ("索引"), new element=w1358) -> (w1361:u16[])
              n897 = case shown="真" w1364 {
                tunnel: w1361 -> [_ w1371]
                tunnel: w1357 -> [_ w1374]
                frame False {
                }
                frame True {
                  n898 = Increment(x=w1374) -> (x+1=→"当前校准":i32)
                  n899 = call "CODMnMB_api.vi"("STEP"=enum16{"open", "read", "write", "close"}."write", "values"=w1371, "starting address"=u16 4274) -> ()  [unwired: 5 in, 4 out]
                }
              }
            }
          }
          frame #1 {
            n900 = local read "当前校准"() -> (w1381:i32)
            n901 = case shown="5" w1381 {
              tunnel: [w1385 w1386 w1387 w1388 w1389] -> w1380
              frame 1, Default {
                n902 = local read "浓度1"() -> (w1385:dbl)
              }
              frame 2 {
                n903 = local read "浓度2"() -> (w1386:dbl)
              }
              frame 3 {
                n904 = local read "浓度3"() -> (w1387:dbl)
              }
              frame 4 {
                n905 = local read "浓度4"() -> (w1388:dbl)
              }
              frame 5 {
                n906 = local read "浓度5"() -> (w1389:dbl)
              }
            }
            n907 = Not Equal To 0?(x=w1380) -> (x != 0?=w1378:bool)
            n908 = case shown="真" w1378 {
              tunnel: [u16 8 ("address") u16 9 ("address")] -> w1384
              tunnel: ["校零" ("测量模式") "校标" ("测量模式")] -> w1379
              frame False {
              }
              frame True {
              }
            }
            n909 = global write "COD测量模式全局.vi" "测量模式"(w1379) -> ()
            n910 = Insert Into Array(array=u16[] [] ("values"), index=0 ("索引"), new element=w1384) -> (w1375:u16[])
            n911 = call "CODMnMB_api.vi"("STEP"=enum16{"open", "read", "write", "close"}."write", "values"=w1375, "starting address"=u16 4608 ("address")) -> ()  [unwired: 5 in, 4 out]
          }
          frame #2 {
            n912 = local read "选用水样"() -> (w1397:enum16{"葡萄糖", "草酸钠"})
            n913 = local read "量程选择"() -> (w1396:enum16{"低量程", "高量程", "0-2量程"})
            n914 = case shown="\"葡萄糖\", 默认" w1397 {
              tunnel: ["葡萄糖标线" ("section") "草酸钠标线" ("section")] -> w1398
              frame "葡萄糖", Default {
              }
              frame "草酸钠" {
              }
            }
            n915 = global read "COD读取DATA全局.vi" "配置文件ini"() -> (w1394:string)
            n916 = case shown="\"0-2量程\"" w1396 {
              tunnel: ["低量程" "高量程" "0-2量程"] -> w1399
              frame "低量程", Default {
              }
              frame "高量程" {
              }
              frame "0-2量程" {
              }
            }
            n917 = call <vilib>:"Application Directory.vi"() -> ("Application Directory"=w1406:path)
            n918 = Concatenate Strings(w1398, w1399) -> (w1395:string)
            n919 = Build Path(base path=w1406, name or relative path=w1394) -> (appended path=w1407:path)
            n920 = local read "当前校准"() -> (w1402:i32)
            n921 = call <vilib>:"Open Config Data.vi"("configuration file path"=w1407) -> ("error out"=w1404:errorcluster, "refnum"=w1405:T16)  [unwired: 8 in, 1 out]
            n922 = call-poly <vilib>:"Write Key.vi"("section"=w1395, "error in (no error)"=w1404, "value"=w1402, "key"="当前选用的校准" ("section"), "refnum"=w1405) -> ("error out"=w1400:errorcluster, "refnum out"=w1401:T16)  [unwired: 4 in, 1 out]
            n923 = call <vilib>:"Close Config Data.vi"("error in (no error)"=w1400, "refnum"=w1401) -> ()  [unwired: 8 in, 2 out]
          }
        }
      }
      event "自动切换量程:", "低切高阈值:", "高切低阈值:": Value Change {
        n924 = event-data() -> ()  [unwired: 1 in, 6 out]
        n925 = flat-sequence {
          frame #0 {
            n926 = local read "自动切换量程:"() -> (w1415:enum16{"关闭", "自动切换测一次", "自动切换测两次"})
            n927 = local read "低切高阈值:"() -> (w1414:dbl)
            n928 = local read "高切低阈值:"() -> (w1413:dbl)
            n929 = global write "CODMn断电保存全局变量.vi" "自动切换量程:"(w1415) -> ()
            n930 = global write "CODMn断电保存全局变量.vi" "低切高阈值:"(w1414) -> ()
            n931 = global write "CODMn断电保存全局变量.vi" "高切低阈值:"(w1413) -> ()
          }
          frame #1 {
            n932 = global read "COD读取DATA全局.vi" "配置文件ini"() -> (w1416:string)
            n933 = call <vilib>:"Application Directory.vi"() -> ("Application Directory"=w1429:path)
            n934 = Build Path(base path=w1429, name or relative path=w1416) -> (appended path=w1428:path)
            n935 = call <vilib>:"Open Config Data.vi"("configuration file path"=w1428) -> ("error out"=w1424:errorcluster, "refnum"=w1427:T16)  [unwired: 8 in, 1 out]
            n936 = vi-ref "斯坦道CODMn.lvlib:CODMn断电保存全局变量.vi"() -> (w1426:refnum<vi>)
            n937 = call <userlib>:"Write Panel to INI__ogtk.vi"("error in (no error)"=w1424, "VI ref"=w1426, "refnum"=w1427) -> ("error out"=w1423:errorcluster, "refnum out"=w1425:T16)  [unwired: 7 in]
            n938 = call <vilib>:"Close Config Data.vi"("error in (no error)"=w1423, "refnum"=w1425) -> ("error out"=w1418:errorcluster, "file path"=w1417:path)  [unwired: 8 in]
            n939 = Open/Create/Replace File(file path (use dialog)=w1417, error in=w1418) -> (refnum out=w1421:refnum<file>, error out=w1422:errorcluster)  [unwired: 4 in, 1 out]
            n940 = Flush File(refnum=w1421, error in=w1422) -> (refnum out=w1420:refnum<file>, error out=w1419:errorcluster)
            n941 = Close File(refnum=w1420, error in=w1419) -> ()  [unwired: 2 out]
          }
        }
      }
      event "模型": Value Change {
        n942 = event-data() -> ()  [unwired: 1 in, 6 out]
        n943 = global read "COD读取DATA全局.vi" "配置文件ini"() -> (w1430:string)
        n944 = call <vilib>:"Application Directory.vi"() -> ("Application Directory"=w1439:path)
        n945 = Build Path(base path=w1439, name or relative path=w1430) -> (appended path=w1438:path)
        n946 = call <vilib>:"Open Config Data.vi"("configuration file path"=w1438) -> ("error out"=w1436:errorcluster, "refnum"=w1437:T16)  [unwired: 8 in, 1 out]
        n947 = local read "模型"() -> (w1431:enum32{"线性", "多项式"})
        n948 = call-poly <vilib>:"Write Key.vi"("section"="CODMn模型选择" ("key"), "error in (no error)"=w1436, "value"=w1431, "key"="线性和多项式", "refnum"=w1437) -> ("error out"=w1432:errorcluster, "refnum out"=w1433:T16)  [unwired: 4 in, 1 out]
        n949 = call <vilib>:"Close Config Data.vi"("error in (no error)"=w1432, "refnum"=w1433) -> ()  [unwired: 8 in, 2 out]
      }
      event "浓度1", "浓度2", "浓度3", "泵滴定数1", "泵滴定数2", "泵滴定数3", "启用1", "启用2", "启用3", "浓度4", "浓度5", "泵滴定数4", "泵滴定数5", "启用4", "启用5": Value Change {
        n950 = event-data() -> ()  [unwired: 1 in, 6 out]
        n951 = global read "COD读取DATA全局.vi" "配置文件ini"() -> (w1440:string)
        n952 = local read "选用水样"() -> (w1456:enum16{"葡萄糖", "草酸钠"})
        n953 = local read "量程选择"() -> (w1455:enum16{"低量程", "高量程", "0-2量程"})
        n954 = case shown="\"0-2量程\"" w1455 {
          tunnel: ["低量程" "高量程" "0-2量程"] -> w1453
          frame "低量程", Default {
          }
          frame "高量程" {
          }
          frame "0-2量程" {
          }
        }
        n955 = call <vilib>:"Application Directory.vi"() -> ("Application Directory"=w1514:path)
        n956 = case shown="\"葡萄糖\", 默认" w1456 {
          tunnel: ["葡萄糖标线" ("section") "草酸钠标线" ("section")] -> w1462
          frame "葡萄糖", Default {
          }
          frame "草酸钠" {
          }
        }
        n957 = Build Path(base path=w1514, name or relative path=w1440) -> (appended path=w1513:path)
        n958 = call <vilib>:"Open Config Data.vi"("configuration file path"=w1513) -> ("error out"=w1511:errorcluster, "refnum"=w1512:T16)  [unwired: 8 in, 1 out]
        n959 = local read "浓度1"() -> (w1509:dbl)
        n960 = Concatenate Strings(w1462, w1453) -> (w1454:string)
        n961 = local read "浓度2"() -> (w1493:dbl)
        n962 = call-poly <vilib>:"Write Key.vi"("section"=w1454, "error in (no error)"=w1511, "value"=w1509, "key"="浓度1", "refnum"=w1512) -> ("error out"=w1508:errorcluster, "refnum out"=w1507:T16)  [unwired: 4 in, 1 out]
        n963 = local read "浓度3"() -> (w1489:dbl)
        n964 = call-poly <vilib>:"Write Key.vi"("section"=w1454, "error in (no error)"=w1508, "value"=w1493, "key"="浓度2", "refnum"=w1507) -> ("error out"=w1506:errorcluster, "refnum out"=w1505:T16)  [unwired: 4 in, 1 out]
        n965 = local read "泵滴定数1"() -> (w1487:dbl)
        n966 = call-poly <vilib>:"Write Key.vi"("section"=w1454, "error in (no error)"=w1506, "value"=w1489, "key"="浓度3", "refnum"=w1505) -> ("error out"=w1504:errorcluster, "refnum out"=w1503:T16)  [unwired: 4 in, 1 out]
        n967 = call-poly <vilib>:"Write Key.vi"("section"=w1454, "error in (no error)"=w1504, "value"=w1487, "key"="泵滴定数1", "refnum"=w1503) -> ("error out"=w1502:errorcluster, "refnum out"=w1501:T16)  [unwired: 4 in, 1 out]
        n968 = local read "泵滴定数2"() -> (w1485:dbl)
        n969 = call-poly <vilib>:"Write Key.vi"("section"=w1454, "error in (no error)"=w1502, "value"=w1485, "key"="泵滴定数2", "refnum"=w1501) -> ("error out"=w1500:errorcluster, "refnum out"=w1499:T16)  [unwired: 4 in, 1 out]
        n970 = local read "泵滴定数3"() -> (w1483:dbl)
        n971 = local read "浓度4"() -> (w1452:dbl)
        n972 = call-poly <vilib>:"Write Key.vi"("section"=w1454, "error in (no error)"=w1500, "value"=w1483, "key"="泵滴定数3", "refnum"=w1499) -> ("error out"=w1498:errorcluster, "refnum out"=w1497:T16)  [unwired: 4 in, 1 out]
        n973 = local read "浓度5"() -> (w1451:dbl)
        n974 = call-poly <vilib>:"Write Key.vi"("section"=w1454, "error in (no error)"=w1498, "value"=w1452, "key"="浓度4", "refnum"=w1497) -> ("error out"=w1491:errorcluster, "refnum out"=w1492:T16)  [unwired: 4 in, 1 out]
        n975 = call-poly <vilib>:"Write Key.vi"("section"=w1454, "error in (no error)"=w1491, "value"=w1451, "key"="浓度5", "refnum"=w1492) -> ("error out"=w1449:errorcluster, "refnum out"=w1450:T16)  [unwired: 4 in, 1 out]
        n976 = local read "泵滴定数4"() -> (w1448:dbl)
        n977 = call-poly <vilib>:"Write Key.vi"("section"=w1454, "error in (no error)"=w1449, "value"=w1448, "key"="泵滴定数4", "refnum"=w1450) -> ("error out"=w1496:errorcluster, "refnum out"=w1495:T16)  [unwired: 4 in, 1 out]
        n978 = local read "泵滴定数5"() -> (w1447:dbl)
        n979 = call-poly <vilib>:"Write Key.vi"("section"=w1454, "error in (no error)"=w1496, "value"=w1447, "key"="泵滴定数5", "refnum"=w1495) -> ("error out"=w1445:errorcluster, "refnum out"=w1446:T16)  [unwired: 4 in, 1 out]
        n980 = local read "启用1"() -> (w1471:bool)
        n981 = call-poly <vilib>:"Write Key.vi"("section"=w1454, "error in (no error)"=w1445, "value"=w1471, "key"="启用1", "refnum"=w1446) -> ("error out"=w1467:errorcluster, "refnum out"=w1470:T16)  [unwired: 4 in, 1 out]
        n982 = local read "启用2"() -> (w1468:bool)
        n983 = call-poly <vilib>:"Write Key.vi"("section"=w1454, "error in (no error)"=w1467, "value"=w1468, "key"="启用2", "refnum"=w1470) -> ("error out"=w1478:errorcluster, "refnum out"=w1477:T16)  [unwired: 4 in, 1 out]
        n984 = local read "启用3"() -> (w1466:bool)
        n985 = call-poly <vilib>:"Write Key.vi"("section"=w1454, "error in (no error)"=w1478, "value"=w1466, "key"="启用3", "refnum"=w1477) -> ("error out"=w1476:errorcluster, "refnum out"=w1475:T16)  [unwired: 4 in, 1 out]
        n986 = local read "启用4"() -> (w1441:bool)
        n987 = call-poly <vilib>:"Write Key.vi"("section"=w1454, "error in (no error)"=w1476, "value"=w1441, "key"="启用4", "refnum"=w1475) -> ("error out"=w1474:errorcluster, "refnum out"=w1473:T16)  [unwired: 4 in, 1 out]
        n988 = local read "启用5"() -> (w1442:bool)
        n989 = call-poly <vilib>:"Write Key.vi"("section"=w1454, "error in (no error)"=w1474, "value"=w1442, "key"="启用5", "refnum"=w1473) -> ("error out"=w1443:errorcluster, "refnum out"=w1444:T16)  [unwired: 4 in, 1 out]
        n990 = local read "选用水样"() -> (w1461:enum16{"葡萄糖", "草酸钠"})
        n991 = call-poly <vilib>:"Write Key.vi"("section"="标线选择", "error in (no error)"=w1443, "value"=w1461, "key"="选用水样", "refnum"=w1444) -> ("error out"=w1458:errorcluster, "refnum out"=w1459:T16)  [unwired: 4 in, 1 out]
        n992 = call <vilib>:"Close Config Data.vi"("error in (no error)"=w1458, "refnum"=w1459) -> ()  [unwired: 8 in, 2 out]
      }
      event "读取": Value Change {
        (unwired) u16 94 ("number of holding registers")
        (unwired) u16 4616 ("starting address")
        n993 = event-data() -> ()  [unwired: 1 in, 6 out]
        n994 = Bundle By Name(cluster=cluster{"命令":string} {"命令"=""} ("元素"), "命令"="CODMn读取公式" ("名称（未命名）")) -> (w1520:cluster{"命令":string})
        n995 = Enqueue Element(queue=w1524, element=w1520, error in (no error)=w1523) -> ()  [unwired: 1 in, 3 out]
      }
      event "写入": Mouse Down {
        n996 = event-data() -> ()  [unwired: 1 in, 8 out]
        n997 = Two Button Dialog(message="确认是否写入公式，写入会覆盖原有公式！" ("消息")) -> (T button?=w1525:bool)  [unwired: 2 in]
        n998 = case shown="真" w1525 {
          frame False {
          }
          frame True {
            n999 = local read "模型"() -> (w1532:enum32{"线性", "多项式"})
            n1000 = case shown="\"多项式\"" w1532 {
              tunnel: [w1536 w1579] -> w1530
              tunnel: [w1535 w1578] -> w1529
              frame "线性", Default {
                n1001 = local read "测量模式(公式)"() -> (w1537:u16)
                n1002 = case shown="1" w1537 {
                  tunnel: [u16 4626 ("starting address") w1544 w1549 w1554 w1559 w1564 w1569 w1574] -> w1536
                  frame 0, Default {
                  }
                  frame 1 {
                    n1003 = local read "量程选择"() -> (w1543:enum16{"低量程", "高量程", "0-2量程"})
                    n1004 = case shown="\"低量程\", 默认" w1543 {
                      tunnel: [u16 4626 ("starting address") u16 4632 ("starting address") u16 4638 ("starting address")] -> w1544
                      frame "低量程", Default {
                      }
                      frame "高量程" {
                      }
                      frame "0-2量程" {
                      }
                    }
                  }
                  frame 2 {
                    n1005 = local read "量程选择"() -> (w1548:enum16{"低量程", "高量程", "0-2量程"})
                    n1006 = case shown="\"低量程\", 默认" w1548 {
                      tunnel: [u16 4638 ("starting address") u16 4644 ("starting address") u16 4638 ("starting address")] -> w1549
                      frame "低量程", Default {
                      }
                      frame "高量程" {
                      }
                      frame "0-2量程" {
                      }
                    }
                  }
                  frame 3 {
                    n1007 = local read "量程选择"() -> (w1553:enum16{"低量程", "高量程", "0-2量程"})
                    n1008 = case shown="\"低量程\", 默认" w1553 {
                      tunnel: [u16 4650 ("starting address") u16 4656 ("starting address") u16 4638 ("starting address")] -> w1554
                      frame "低量程", Default {
                      }
                      frame "高量程" {
                      }
                      frame "0-2量程" {
                      }
                    }
                  }
                  frame 4 {
                    n1009 = local read "量程选择"() -> (w1558:enum16{"低量程", "高量程", "0-2量程"})
                    n1010 = case shown="\"低量程\", 默认" w1558 {
                      tunnel: [u16 4662 ("starting address") u16 4668 ("starting address") u16 4638 ("starting address")] -> w1559
                      frame "低量程", Default {
                      }
                      frame "高量程" {
                      }
                      frame "0-2量程" {
                      }
                    }
                  }
                  frame 5 {
                    n1011 = local read "量程选择"() -> (w1563:enum16{"低量程", "高量程", "0-2量程"})
                    n1012 = case shown="\"低量程\", 默认" w1563 {
                      tunnel: [u16 4674 ("starting address") u16 4680 ("starting address") u16 4638 ("starting address")] -> w1564
                      frame "低量程", Default {
                      }
                      frame "高量程" {
                      }
                      frame "0-2量程" {
                      }
                    }
                  }
                  frame 6 {
                    n1013 = local read "量程选择"() -> (w1568:enum16{"低量程", "高量程", "0-2量程"})
                    n1014 = case shown="\"低量程\", 默认" w1568 {
                      tunnel: [u16 4686 ("starting address") u16 4692 ("starting address") u16 4638 ("starting address")] -> w1569
                      frame "低量程", Default {
                      }
                      frame "高量程" {
                      }
                      frame "0-2量程" {
                      }
                    }
                  }
                  frame 7 {
                    n1015 = local read "量程选择"() -> (w1573:enum16{"低量程", "高量程", "0-2量程"})
                    n1016 = case shown="\"低量程\", 默认" w1573 {
                      tunnel: [u16 4698 ("starting address") u16 4704 ("starting address") u16 4638 ("starting address")] -> w1574
                      frame "低量程", Default {
                      }
                      frame "高量程" {
                      }
                      frame "0-2量程" {
                      }
                    }
                  }
                }
                n1017 = local read "K"() -> (w1541:dbl)
                n1018 = local read "b"() -> (w1540:dbl)
                n1019 = Build Array(w1541, w1540, 0.0 ("元素")) -> (w1539:dbl[])
                n1020 = call "浮点转CDAB整形cod.vi"("浮点数"=w1539) -> ("CDAB整形输出"=w1535:u16[])  [unwired: 10 in]
              }
              frame "多项式" {
                # "b,k,c"
                n1021 = local read "测量模式(公式)"() -> (w1580:u16)
                n1022 = case shown="1" w1580 {
                  tunnel: [u16 4626 ("starting address") w1588 w1593 w1598 w1603 w1608 w1613 w1618] -> w1579
                  frame 0, Default {
                  }
                  frame 1 {
                    n1023 = local read "量程选择"() -> (w1587:enum16{"低量程", "高量程", "0-2量程"})
                    n1024 = case shown="\"低量程\", 默认" w1587 {
                      tunnel: [u16 4626 ("starting address") u16 4632 ("starting address") u16 4638 ("starting address")] -> w1588
                      frame "低量程", Default {
                      }
                      frame "高量程" {
                      }
                      frame "0-2量程" {
                      }
                    }
                  }
                  frame 2 {
                    n1025 = local read "量程选择"() -> (w1592:enum16{"低量程", "高量程", "0-2量程"})
                    n1026 = case shown="\"低量程\", 默认" w1592 {
                      tunnel: [u16 4638 ("starting address") u16 4644 ("starting address") u16 4638 ("starting address")] -> w1593
                      frame "低量程", Default {
                      }
                      frame "高量程" {
                      }
                      frame "0-2量程" {
                      }
                    }
                  }
                  frame 3 {
                    n1027 = local read "量程选择"() -> (w1597:enum16{"低量程", "高量程", "0-2量程"})
                    n1028 = case shown="\"低量程\", 默认" w1597 {
                      tunnel: [u16 4650 ("starting address") u16 4656 ("starting address") u16 4638 ("starting address")] -> w1598
                      frame "低量程", Default {
                      }
                      frame "高量程" {
                      }
                      frame "0-2量程" {
                      }
                    }
                  }
                  frame 4 {
                    n1029 = local read "量程选择"() -> (w1602:enum16{"低量程", "高量程", "0-2量程"})
                    n1030 = case shown="\"低量程\", 默认" w1602 {
                      tunnel: [u16 4662 ("starting address") u16 4668 ("starting address") u16 4638 ("starting address")] -> w1603
                      frame "低量程", Default {
                      }
                      frame "高量程" {
                      }
                      frame "0-2量程" {
                      }
                    }
                  }
                  frame 5 {
                    n1031 = local read "量程选择"() -> (w1607:enum16{"低量程", "高量程", "0-2量程"})
                    n1032 = case shown="\"低量程\", 默认" w1607 {
                      tunnel: [u16 4674 ("starting address") u16 4680 ("starting address") u16 4638 ("starting address")] -> w1608
                      frame "低量程", Default {
                      }
                      frame "高量程" {
                      }
                      frame "0-2量程" {
                      }
                    }
                  }
                  frame 6 {
                    n1033 = local read "量程选择"() -> (w1612:enum16{"低量程", "高量程", "0-2量程"})
                    n1034 = case shown="\"低量程\", 默认" w1612 {
                      tunnel: [u16 4686 ("starting address") u16 4692 ("starting address") u16 4638 ("starting address")] -> w1613
                      frame "低量程", Default {
                      }
                      frame "高量程" {
                      }
                      frame "0-2量程" {
                      }
                    }
                  }
                  frame 7 {
                    n1035 = local read "量程选择"() -> (w1617:enum16{"低量程", "高量程", "0-2量程"})
                    n1036 = case shown="\"低量程\", 默认" w1617 {
                      tunnel: [u16 4698 ("starting address") u16 4704 ("starting address") u16 4638 ("starting address")] -> w1618
                      frame "低量程", Default {
                      }
                      frame "高量程" {
                      }
                      frame "0-2量程" {
                      }
                    }
                  }
                }
                n1037 = local read "多项式系数"() -> (w1585:dbl[])
                n1038 = Index Array(array=w1585) -> (element #1=w1582:dbl, element #2=w1583:dbl, element #3=w1581:dbl)  [unwired: 3 in]
                n1039 = Build Array(w1583, w1582, w1581) -> (w1584:dbl[])
                n1040 = call "浮点转CDAB整形cod.vi"("浮点数"=w1584) -> ("CDAB整形输出"=w1578:u16[])  [unwired: 10 in]
              }
            }
            n1041 = call "CODMnMB_api.vi"("STEP"=enum16{"open", "read", "write", "close"}."write", "values"=w1529, "starting address"=w1530) -> ("error out"=w1528:errorcluster)  [unwired: 5 in, 3 out]
            n1042 = case shown="错误" w1528 {
              tunnel: ["写入成功！" "写入失败！"] -> w1527
              frame No Error {
              }
              frame Error {
              }
            }
            n1043 = One Button Dialog(message=w1527) -> ()  [unwired: 1 in, 1 out]
          }
        }
      }
      event "一键写入": Value Change {
        n1044 = event-data() -> ()  [unwired: 1 in, 6 out]
        n1045 = Two Button Dialog(message="确认是否写入公式，写入会覆盖原有公式！" ("消息")) -> (T button?=w1622:bool)  [unwired: 2 in]
        n1046 = case shown="真" w1622 {
          frame False {
          }
          frame True {
            n1047 = local read "模型"() -> (w1626:enum32{"线性", "多项式"})
            n1048 = case shown="\"多项式\"" w1626 {
              tunnel: [w1629 w1680] -> w1624
              frame "线性", Default {
                n1049 = property on="测量模式(公式)" class="Ring (严格)"() -> ("NumItems"=w1630:u32)  [unwired: 2 in, 2 out]
                n1050 = for {
                  N: w1630 -> [_]
                  tunnel: [w1631] -> w1629
                  i -> [w1636]
                  n1051 = Increment(x=w1636) -> (x+1=w1635:i32)
                  n1052 = local read "K"() -> (w1640:dbl)
                  n1053 = case shown="1" w1635 {
                    tunnel: [u16 4626 ("starting address") w1646 w1651 w1656 w1661 w1666 w1671 w1676] -> w1633
                    frame 0, Default {
                    }
                    frame 1 {
                      n1054 = local read "量程选择"() -> (w1645:enum16{"低量程", "高量程", "0-2量程"})
                      n1055 = case shown="\"低量程\", 默认" w1645 {
                        tunnel: [u16 4626 ("starting address") u16 4632 ("starting address") u16 4638 ("starting address")] -> w1646
                        frame "低量程", Default {
                        }
                        frame "高量程" {
                        }
                        frame "0-2量程" {
                        }
                      }
                    }
                    frame 2 {
                      n1056 = local read "量程选择"() -> (w1650:enum16{"低量程", "高量程", "0-2量程"})
                      n1057 = case shown="\"低量程\", 默认" w1650 {
                        tunnel: [u16 4638 ("starting address") u16 4644 ("starting address") u16 4638 ("starting address")] -> w1651
                        frame "低量程", Default {
                        }
                        frame "高量程" {
                        }
                        frame "0-2量程" {
                        }
                      }
                    }
                    frame 3 {
                      n1058 = local read "量程选择"() -> (w1655:enum16{"低量程", "高量程", "0-2量程"})
                      n1059 = case shown="\"低量程\", 默认" w1655 {
                        tunnel: [u16 4650 ("starting address") u16 4656 ("starting address") u16 4638 ("starting address")] -> w1656
                        frame "低量程", Default {
                        }
                        frame "高量程" {
                        }
                        frame "0-2量程" {
                        }
                      }
                    }
                    frame 4 {
                      n1060 = local read "量程选择"() -> (w1660:enum16{"低量程", "高量程", "0-2量程"})
                      n1061 = case shown="\"高量程\"" w1660 {
                        tunnel: [u16 4662 ("starting address") u16 4668 ("starting address") u16 4638 ("starting address")] -> w1661
                        frame "低量程", Default {
                        }
                        frame "高量程" {
                        }
                        frame "0-2量程" {
                        }
                      }
                    }
                    frame 5 {
                      n1062 = local read "量程选择"() -> (w1665:enum16{"低量程", "高量程", "0-2量程"})
                      n1063 = case shown="\"低量程\", 默认" w1665 {
                        tunnel: [u16 4674 ("starting address") u16 4680 ("starting address") u16 4638 ("starting address")] -> w1666
                        frame "低量程", Default {
                        }
                        frame "高量程" {
                        }
                        frame "0-2量程" {
                        }
                      }
                    }
                    frame 6 {
                      n1064 = local read "量程选择"() -> (w1670:enum16{"低量程", "高量程", "0-2量程"})
                      n1065 = case shown="\"低量程\", 默认" w1670 {
                        tunnel: [u16 4686 ("starting address") u16 4692 ("starting address") u16 4638 ("starting address")] -> w1671
                        frame "低量程", Default {
                        }
                        frame "高量程" {
                        }
                        frame "0-2量程" {
                        }
                      }
                    }
                    frame 7 {
                      n1066 = local read "量程选择"() -> (w1675:enum16{"低量程", "高量程", "0-2量程"})
                      n1067 = case shown="\"低量程\", 默认" w1675 {
                        tunnel: [u16 4698 ("starting address") u16 4704 ("starting address") u16 4638 ("starting address")] -> w1676
                        frame "低量程", Default {
                        }
                        frame "高量程" {
                        }
                        frame "0-2量程" {
                        }
                      }
                    }
                  }
                  n1068 = local read "b"() -> (w1641:dbl)
                  n1069 = Build Array(w1640, w1641, 0.0 ("元素")) -> (w1642:dbl[])
                  n1070 = call "浮点转CDAB整形cod.vi"("浮点数"=w1642) -> ("CDAB整形输出"=w1639:u16[])  [unwired: 10 in]
                  n1071 = Insert Into Array(array=u16[] [], index=0 ("索引"), new element=w1639) -> (w1632:u16[])
                  n1072 = call "CODMnMB_api.vi"("STEP"=enum16{"open", "read", "write", "close"}."write", "values"=w1632, "starting address"=w1633) -> ("error out"=w1631:errorcluster)  [unwired: 5 in, 3 out]
                }
              }
              frame "多项式" {
                # "b,k,c"
                n1073 = property on="测量模式(公式)" class="Ring (严格)"() -> ("NumItems"=w1681:u32)  [unwired: 2 in, 2 out]
                n1074 = for {
                  N: w1681 -> [_]
                  tunnel: [w1682] -> w1680
                  i -> [w1687]
                  n1075 = local read "多项式系数"() -> (w1691:dbl[])
                  n1076 = Increment(x=w1687) -> (x+1=w1686:i32)
                  n1077 = case shown="2" w1686 {
                    tunnel: [u16 4626 ("starting address") w1698 w1703 w1708 w1713 w1718 w1723 w1728] -> w1683
                    frame 0, Default {
                    }
                    frame 1 {
                      n1078 = local read "量程选择"() -> (w1697:enum16{"低量程", "高量程", "0-2量程"})
                      n1079 = case shown="\"低量程\", 默认" w1697 {
                        tunnel: [u16 4626 ("starting address") u16 4632 ("starting address") u16 4638 ("starting address")] -> w1698
                        frame "低量程", Default {
                        }
                        frame "高量程" {
                        }
                        frame "0-2量程" {
                        }
                      }
                    }
                    frame 2 {
                      n1080 = local read "量程选择"() -> (w1702:enum16{"低量程", "高量程", "0-2量程"})
                      n1081 = case shown="\"低量程\", 默认" w1702 {
                        tunnel: [u16 4638 ("starting address") u16 4644 ("starting address") u16 4638 ("starting address")] -> w1703
                        frame "低量程", Default {
                        }
                        frame "高量程" {
                        }
                        frame "0-2量程" {
                        }
                      }
                    }
                    frame 3 {
                      n1082 = local read "量程选择"() -> (w1707:enum16{"低量程", "高量程", "0-2量程"})
                      n1083 = case shown="\"低量程\", 默认" w1707 {
                        tunnel: [u16 4650 ("starting address") u16 4656 ("starting address") u16 4638 ("starting address")] -> w1708
                        frame "低量程", Default {
                        }
                        frame "高量程" {
                        }
                        frame "0-2量程" {
                        }
                      }
                    }
                    frame 4 {
                      n1084 = local read "量程选择"() -> (w1712:enum16{"低量程", "高量程", "0-2量程"})
                      n1085 = case shown="\"低量程\", 默认" w1712 {
                        tunnel: [u16 4662 ("starting address") u16 4668 ("starting address") u16 4638 ("starting address")] -> w1713
                        frame "低量程", Default {
                        }
                        frame "高量程" {
                        }
                        frame "0-2量程" {
                        }
                      }
                    }
                    frame 5 {
                      n1086 = local read "量程选择"() -> (w1717:enum16{"低量程", "高量程", "0-2量程"})
                      n1087 = case shown="\"低量程\", 默认" w1717 {
                        tunnel: [u16 4674 ("starting address") u16 4680 ("starting address") u16 4638 ("starting address")] -> w1718
                        frame "低量程", Default {
                        }
                        frame "高量程" {
                        }
                        frame "0-2量程" {
                        }
                      }
                    }
                    frame 6 {
                      n1088 = local read "量程选择"() -> (w1722:enum16{"低量程", "高量程", "0-2量程"})
                      n1089 = case shown="\"低量程\", 默认" w1722 {
                        tunnel: [u16 4686 ("starting address") u16 4692 ("starting address") u16 4638 ("starting address")] -> w1723
                        frame "低量程", Default {
                        }
                        frame "高量程" {
                        }
                        frame "0-2量程" {
                        }
                      }
                    }
                    frame 7 {
                      n1090 = local read "量程选择"() -> (w1727:enum16{"低量程", "高量程", "0-2量程"})
                      n1091 = case shown="\"低量程\", 默认" w1727 {
                        tunnel: [u16 4698 ("starting address") u16 4704 ("starting address") u16 4638 ("starting address")] -> w1728
                        frame "低量程", Default {
                        }
                        frame "高量程" {
                        }
                        frame "0-2量程" {
                        }
                      }
                    }
                  }
                  n1092 = Index Array(array=w1691) -> (element #1=w1694:dbl, element #2=w1693:dbl, element #3=w1695:dbl)  [unwired: 3 in]
                  n1093 = Build Array(w1693, w1694, w1695) -> (w1692:dbl[])
                  n1094 = call "浮点转CDAB整形cod.vi"("浮点数"=w1692) -> ("CDAB整形输出"=w1690:u16[])  [unwired: 10 in]
                  n1095 = Insert Into Array(array=u16[] [], index=0 ("索引"), new element=w1690) -> (w1684:u16[])
                  n1096 = call "CODMnMB_api.vi"("STEP"=enum16{"open", "read", "write", "close"}."write", "values"=w1684, "starting address"=w1683) -> ("error out"=w1682:errorcluster)  [unwired: 5 in, 3 out]
                }
              }
            }
            n1097 = case shown="无错误" w1624 {
              tunnel: ["写入成功！" "写入失败！"] -> w1625
              frame No Error {
              }
              frame Error {
              }
            }
            n1098 = One Button Dialog(message=w1625) -> ()  [unwired: 1 in, 1 out]
          }
        }
      }
      event "滴定曲线": Value Change {
        n1099 = event-data() -> ()  [unwired: 1 in, 6 out]
        n1100 = property on="窗格" class="Pane"("Origin"=T17 {"Horizontal"=0, "Vertical"=3200} ("原点")) -> ()  [unwired: 2 in, 2 out]
      }
      event "历史波形": Value Change {
        n1101 = event-data() -> ()  [unwired: 1 in, 6 out]
        n1102 = call-poly <vilib>:"Read Waveforms from File.vi"() -> ("error out"=w1733:errorcluster, "first waveform in record"=w1734:waveform(dbl))  [unwired: 6 in, 2 out]
        n1103 = case shown="无错误" w1733 {
          tunnel: w1734 -> [w1737 _]
          frame No Error {
            n1104 = Unbundle By Name(w1737) -> ("t0"=→"波形时间":timestamp, "Y"=w1736:dbl[])  [unwired: 2 out]
            n1105 = local write "滴定数-ORP值"(w1736) -> ()
            n1106 = local write "ORP滴定曲线"(w1736) -> ()
          }
          frame Error {
            n1107 = One Button Dialog(message="打开失败" ("消息")) -> ()  [unwired: 1 in, 1 out]
          }
        }
      }
      event "释放串口": Value Change {
        n1108 = event-data() -> ()  [unwired: 1 in, 6 out]
        n1109 = Two Button Dialog(message="确认是否释放串口，释放串口将导致通信失败！" ("消息")) -> (T button?=w1739:bool)  [unwired: 2 in]
        n1110 = case shown="真" w1739 {
          tunnel: w1742 -> [_ w1744]
          tunnel: w1741 -> [_ w1743]
          frame False {
          }
          frame True {
            n1111 = Bundle By Name(cluster=cluster{"命令":string} {"命令"=""} ("元素"), "命令"="停用模块" ("名称（未命名）")) -> (w1745:cluster{"命令":string})
            n1112 = Enqueue Element(queue=w1744, element=w1745, error in (no error)=w1743) -> ()  [unwired: 1 in, 3 out]
          }
        }
      }
      event "打开串口": Value Change {
        n1113 = event-data() -> ()  [unwired: 1 in, 6 out]
        n1114 = flat-sequence {
          tunnel: w1749 -> [w1757]
          tunnel: w1748 -> [w1756]
          frame #0 {
            n1115 = global read "CODMn断电保存全局变量.vi" "MB通信方式选择"() -> (w1753:enum16{"串口", "TCP"})
            n1116 = global read "CODMn断电保存全局变量.vi" "VISA resource name"() -> (w1760:refnum<visa-resource-name>)
            n1117 = global read "CODMn断电保存全局变量.vi" "PORT"() -> (w1751:string)
            n1118 = global read "CODMn断电保存全局变量.vi" "IP"() -> (w1752:string)
            n1119 = call "串口配置.vi"("PORT"=w1751, "IP"=w1752, "MB通信方式选择"=w1753, "请选择串口:"=w1760) -> ("PORT 2"=w1754:string, "IP 2"=w1755:string, "确认 2"=w1758:bool, "VISA资源名称 2"=w1759:refnum<visa-resource-name>, "MB通信方式选择 2"=w1750:enum16{"串口", "TCP"})  [unwired: 3 in]
            n1120 = case shown="真" w1758 {
              tunnel: w1759 -> [_ w1769]
              tunnel: w1757 -> [_ w1765]
              tunnel: w1756 -> [_ w1764]
              tunnel: w1755 -> [_ w1763]
              tunnel: w1754 -> [_ w1762]
              tunnel: w1750 -> [_ w1761]
              frame False {
              }
              frame True {
                n1121 = global write "CODMn断电保存全局变量.vi" "MB通信方式选择"(w1761) -> ()
                n1122 = global write "CODMn断电保存全局变量.vi" "VISA resource name"(w1769) -> ()
                n1123 = global write "CODMn断电保存全局变量.vi" "PORT"(w1762) -> ()
                n1124 = global write "CODMn断电保存全局变量.vi" "IP"(w1763) -> ()
                n1125 = Bundle By Name(cluster=cluster{"命令":string} {"命令"=""} ("元素"), "命令"="启用模块" ("名称（未命名）")) -> (w1766:cluster{"命令":string})
                n1126 = Enqueue Element(queue=w1765, element=w1766, error in (no error)=w1764) -> ()  [unwired: 1 in, 3 out]
              }
            }
          }
          frame #1 {
            n1127 = global read "COD读取DATA全局.vi" "配置文件ini"() -> (w1783:string)
            n1128 = call <vilib>:"Application Directory.vi"() -> ("Application Directory"=w1770:path)
            n1129 = Build Path(base path=w1770, name or relative path=w1783) -> (appended path=w1771:path)
            n1130 = call <vilib>:"Open Config Data.vi"("configuration file path"=w1771) -> ("error out"=w1775:errorcluster, "refnum"=w1772:T16)  [unwired: 8 in, 1 out]
            n1131 = vi-ref "斯坦道CODMn.lvlib:CODMn断电保存全局变量.vi"() -> (w1773:refnum<vi>)
            n1132 = call <userlib>:"Write Panel to INI__ogtk.vi"("error in (no error)"=w1775, "VI ref"=w1773, "refnum"=w1772) -> ("error out"=w1776:errorcluster, "refnum out"=w1774:T16)  [unwired: 7 in]
            n1133 = call <vilib>:"Close Config Data.vi"("error in (no error)"=w1776, "refnum"=w1774) -> ("error out"=w1781:errorcluster, "file path"=w1782:path)  [unwired: 8 in]
            n1134 = Open/Create/Replace File(file path (use dialog)=w1782, error in=w1781) -> (refnum out=w1778:refnum<file>, error out=w1777:errorcluster)  [unwired: 4 in, 1 out]
            n1135 = Flush File(refnum=w1778, error in=w1777) -> (refnum out=w1779:refnum<file>, error out=w1780:errorcluster)
            n1136 = Close File(refnum=w1779, error in=w1780) -> ()  [unwired: 2 out]
          }
        }
      }
      event Timeout {
        n1137 = event-data() -> ()  [unwired: 1 in, 3 out]
      }
    }
  }
  n1138 = while {
    tunnel: w2 -> [w1789]
    tunnel: w1 -> [w1788]
    tunnel: [w1784] -> _
    stop <- FALSE stop-if-true
    # "CODMn与外部交互"
    n1139 = Dequeue Element(queue=w1789, error in (no error)=w1788) -> (element=w1790:T4)  [unwired: 1 in, 3 out]
    n1140 = Unbundle By Name(w1790) -> ("命令"=w1787:string, "测量模式"=w1786:T18, "CODMn量程切换"=w1785:enum32{"H", "L", "AUTO"})
    n1141 = case shown="\"停止命令\"" w1787 {
      tunnel: w1786 -> [_ w1793 _ _]
      tunnel: w1785 -> [_ _ _ w1823]
      tunnel: [_ w1792 w1818 w1822] -> w1784
      frame "假", Default {
      }
      frame "启动命令" {
        n1142 = case shown="\"校零\"" w1793 {
          tunnel: [u16 4608 ("address") u16 4608 ("address") u16 4608 ("address") u16 4608 ("address") u16 4608 ("address") u16 4608 ("address") u16 4608 ("address") u16 4608 ("address") u16 4608 ("address")] -> w1795
          tunnel: [u16 1 ("address") u16 2 ("address") u16 3 ("address") u16 4 ("address") u16 5 ("address") u16 7 ("address") u16 6 ("address") u16 8 ("address") u16 9 ("address")] -> w1799
          frame "水样测量" {
          }
          frame "标样核查" {
          }
          frame "零点核查" {
          }
          frame "跨度核查" {
          }
          frame "空白测试" {
          }
          frame "加标回收" {
          }
          frame "平行样" {
          }
          frame "校零" {
          }
          frame "校标" {
          }
        }
        n1143 = Insert Into Array(array=u16[] [] ("values"), index=0 ("索引"), new element=w1799) -> (w1794:u16[])
        n1144 = call "CODMnMB_api.vi"("STEP"=enum16{"open", "read", "write", "close"}."write", "values"=w1794, "starting address"=w1795) -> ("error out"=w1792:errorcluster)  [unwired: 5 in, 3 out]
      }
      frame "停止命令" {
        n1145 = call "CODMnMB_api.vi"("STEP"=enum16{"open", "read", "write", "close"}."write", "values"=u16[] [11], "starting address"=u16 4608) -> ("error out"=w1818:errorcluster)  [unwired: 5 in, 3 out]
      }
      frame "量程切换" {
        n1146 = case shown="\"H\"" w1823 {
          tunnel: [u16[] [1] ("values") u16[] [0] ("values") _] -> w1826
          frame "H" {
          }
          frame "L" {
          }
          frame "AUTO", Default {
          }
        }
        n1147 = call "CODMnMB_api.vi"("STEP"=enum16{"open", "read", "write", "close"}."write", "values"=w1826, "starting address"=u16 4276) -> ("error out"=w1822:errorcluster)  [unwired: 5 in, 3 out]
      }
    }
  }
  n1148 = while {
    tunnel: w16 -> [w1838]
    tunnel: w15 -> [w1837]
    tunnel: w7 -> [_]
    stop <- FALSE stop-if-true
    # "主循环界面显示"
    n1149 = flat-sequence {
      frame #0 {
        # "测量状态显示"
        n1150 = global read "COD读取DATA全局.vi" "测量状态"() -> (w1872:u16[])
        n1151 = To Word Integer(number=w1872) -> (16bit integer=w1883:i16[])
        n1152 = Index Array(array=w1883, index #1=0 ("索引"), index #4=3 ("索引"), index #14=13 ("索引"), index #15=14 ("索引"), index #21=20 ("索引"), index #32=31 ("索引")) -> (element #1=w1888:i16, element #2=w1887:i16, element #3=w1886:i16, element #4=→"CODMn工作状态":i16, element #5=→"模式（受控）":i16, element #6=→"进样管":i16, element #7=→"高锰酸钾":i16, element #8=→"草酸钠":i16, element #9=→"硫酸":i16, element #10=w1882:i16, element #11=w1903:i16, element #12=w1878:i16, element #13=→"报警数字":i16, element #14=w1909:i16, element #15=w1894:i16, element #16=→"多列列表框":i16, element #21=w1870:i16, element #33=→"分":i16, element #34=→"秒":i16)  [unwired: 28 in, 15 out]
        n1153 = Number To Decimal String(number=w1870) -> (decimal integer string=→"基本量程(显示)":string)  [unwired: 1 in]
        n1154 = global write "COD读取DATA全局.vi" "基本量程存储数据用"(w1870) -> ()
        n1155 = Build Array(w1888, w1887, w1886) -> (w1889:i16[])
        n1156 = To Single Precision Float(number=w1882) -> (single precision float=→"ORP显示":sgl)
        n1157 = call "HexToDate.vi"("数组"=w1889) -> ("DATE"=w1884:timestamp[])  [unwired: 10 in]
        n1158 = Index Array(array=w1884) -> (element=→"仪器时间":timestamp)  [unwired: 1 in]
        n1159 = Divide(x=w1903, y=u16 10) -> (x/y=→"温度":dbl)
        n1160 = Divide(x=w1894, y=u16 1000) -> (x/y=→"标度滴定值":dbl)
        n1161 = Equal?(x=w1878, y=u16 2) -> (x = y?=→"断电排液标记":bool)
        n1162 = Equal?(x=w1878, y=u16 1) -> (x = y?=→"排液标记":bool)
        n1163 = Divide(x=w1909, y=u16 1000) -> (x/y=→"零点滴定值":dbl)
      }
    }
    n1164 = flat-sequence {
      frame #0 {
        # "工作状态显示"
        n1165 = local read "CODMn工作状态"() -> (w1847:T1)
        n1166 = Equal?(x=w1847, y=u16 0) -> (x = y?=→"待机":bool)
        n1167 = Equal?(x=w1847, y=u16 8) -> (x = y?=→"校零标记":bool)
        n1168 = Equal?(x=w1847, y=u16 9) -> (x = y?=→"校标标记":bool)
        n1169 = Equal?(x=w1847, y=u16 1) -> (x = y?=→"水样测量":bool)
        n1170 = Equal?(x=w1847, y=u16 7) -> (x = y?=→"质控样测量":bool)
        n1171 = Equal?(x=w1847, y=u16 10) -> (x = y?=→"加标回收测量":bool)
        n1172 = Equal?(x=w1847, y=u16 2) -> (x = y?=→"标样核查标记":bool)
        n1173 = Equal?(x=w1847, y=u16 6) -> (x = y?=→"平行样测量":bool)
        n1174 = Equal?(x=w1847, y=u16 3) -> (x = y?=→"零点核查标记":bool)
        n1175 = Equal?(x=w1847, y=u16 4) -> (x = y?=→"跨度核查标记":bool)
        n1176 = Equal?(x=w1847, y=u16 5) -> (x = y?=→"空白测试标记":bool)
      }
    }
    n1177 = First Call?() -> (First Call?: T/F=w1836:bool)
    n1178 = case shown="真" w1836 {
      tunnel: w1838 -> [w1937 w1942]
      tunnel: w1837 -> [w1936 w1941]
      tunnel: [w1937 w1940] -> w1834
      tunnel: [w1936 w1939] -> w1833
      frame False {
      }
      frame True {
        n1179 = Bundle By Name(cluster=cluster{"命令":string} {"命令"=""} ("元素"), "命令"="CODMn读取参数" ("名称（未命名）")) -> (w1945:cluster{"命令":string})
        n1180 = Enqueue Element(queue=w1942, element=w1945, timeout in ms (-1)=1000 ("超时毫秒(-1)"), error in (no error)=w1941) -> (queue out=w1940:refnum<queue>, error out=w1939:errorcluster)  [unwired: 1 out]
      }
    }
    n1181 = Wait (ms)(milliseconds to wait=u32 1000 ("等待时间（毫秒）")) -> ()  [unwired: 1 out]
    n1182 = Get Queue Status(queue=w1834, error in (no error)=w1833) -> (queue out=w1830:refnum<queue>, error out=w1829:errorcluster, # elements in queue=w1832:i32)  [unwired: 1 in, 5 out]
    n1183 = Equal To 0?(x=w1832) -> (x = 0?=w1831:bool)
    n1184 = flat-sequence {
      frame #0 {
        # "CODMn读取状态"
        n1185 = global read "COD读取DATA全局.vi" "M输出点"() -> (w1956:bool[])
        n1186 = global read "COD读取DATA全局.vi" "温度"() -> (w1957:bool[])
        n1187 = Index Array(array=w1957) -> (element=→"加热":bool)  [unwired: 1 in]
        n1188 = Index Array(array=w1956) -> (element #1=→"搅拌":bool, element #4=→"进水样":bool, element #5=→"进蒸馏水":bool, element #6=→"进标液":bool, element #7=→"进质控样":bool, element #8=→"进加标回收样":bool, element #9=→"进高锰酸钾":bool, element #10=→"进草酸钠":bool, element #11=→"进硫酸":bool)  [unwired: 11 in, 2 out]
      }
    }
    n1189 = case shown="真" w1831 {
      tunnel: w1830 -> [_ w1842]
      tunnel: w1829 -> [_ w1841]
      frame False {
      }
      frame True {
        n1190 = Bundle By Name(cluster=cluster{"命令":string} {"命令"=""} ("元素"), "命令"="CODMn读取" ("名称（未命名）")) -> (w1844:cluster{"命令":string})
        n1191 = Enqueue Element(queue=w1842, element=w1844, timeout in ms (-1)=1000 ("超时毫秒(-1)"), error in (no error)=w1841) -> ()  [unwired: 3 out]
      }
    }
    n1192 = Get Date/Time In Seconds() -> (seconds since 1Jan1904=→"系统时间":timestamp)
    n1193 = flat-sequence {
      frame #0 {
        # "A，B，K"
        # "CODMn读取状态"
        n1194 = global read "COD读取DATA全局.vi" "ORP、时间"() -> (w1960:u16[])
        n1195 = To Word Integer(number=w1960) -> (16bit integer=w1981:i16[])
        n1196 = Split 1D Array(array=w1981, index=3 ("索引")) -> (first subarray=w1962:i16[], second subarray=w1980:i16[])
        n1197 = Index Array(array=w1962) -> (element #1=w1966:i16, element #2=w1965:i16, element #3=w1964:i16)  [unwired: 3 in]
        n1198 = Index Array(array=w1980) -> (element #1=w1975:i16, element #2=w1979:i16, element #3=w1978:i16, element #4=w1977:i16)  [unwired: 4 in]
        n1199 = Build Array(w1966, w1965, w1964) -> (w1963:i16[])
        n1200 = To Single Precision Float(number=w1978) -> (single precision float=w1969:sgl)
        n1201 = To Single Precision Float(number=w1975) -> (single precision float=w1974:sgl)
        n1202 = To Single Precision Float(number=w1979) -> (single precision float=w1973:sgl)
        n1203 = To Single Precision Float(number=w1977) -> (single precision float=w1968:sgl)
        n1204 = call "HexToDate.vi"("数组"=w1963) -> ("DATE"=w1967:timestamp[])  [unwired: 10 in]
        n1205 = Divide(x=w1974, y=sgl 100.0) -> (x/y=→"COD浓度（mg/L)":sgl)
        n1206 = Index Array(array=w1967) -> (element=w1961:timestamp)  [unwired: 1 in]
        n1207 = Number To Decimal String(number=w1973) -> (decimal integer string=→"ORP-A":string)  [unwired: 1 in]
        n1208 = Number To Decimal String(number=w1969) -> (decimal integer string=→"ORP-B":string)  [unwired: 1 in]
        n1209 = Number To Decimal String(number=w1968) -> (decimal integer string=→"ORP-K":string)  [unwired: 1 in]
        n1210 = Format Date/Time String(seconds (now)=w1961) -> (date/time string=→"数据时间":string)  [unwired: 2 in]
      }
    }
    n1211 = flat-sequence {
      frame #0 {
        # "报警状态显示"
        n1212 = local read "报警数字"() -> (w1912:i16)
        n1213 = Equal?(x=w1912, y=u16 9) -> (x = y?=w1915:bool)
        "进水样超量程" <- w1915
        n1214 = Equal?(x=w1912, y=u16 10) -> (x = y?=w1914:bool)
        "排液故障" <- w1914
        n1215 = Equal?(x=w1912, y=u16 2) -> (x = y?=w1922:bool)
        "温控器故障" <- w1922
        n1216 = Equal?(x=w1912, y=u16 3) -> (x = y?=w1921:bool)
        "加热故障" <- w1921
        n1217 = Equal?(x=w1912, y=u16 4) -> (x = y?=w1920:bool)
        "高锰酸钾报警" <- w1920
        n1218 = Equal?(x=w1912, y=u16 5) -> (x = y?=w1919:bool)
        "草酸钠报警" <- w1919
        n1219 = Equal?(x=w1912, y=u16 6) -> (x = y?=w1918:bool)
        "测量错误" <- w1918
        n1220 = Equal?(x=w1912, y=u16 8) -> (x = y?=w1917:bool)
        "校零错误" <- w1917
        n1221 = Equal?(x=w1912, y=u16 7) -> (x = y?=w1916:bool)
        "校标错误" <- w1916
        n1222 = Equal?(x=w1912, y=u16 1) -> (x = y?=w1923:bool)
        "ORP故障" <- w1923
        n1223 = Compound Arithmetic op=OR ("复合运算")(w1923, w1922, w1921, w1920, w1919, w1918, w1916, w1917, w1915, w1914) -> (→"故障标记":bool)
        n1224 = Bundle By Name(cluster=T3 {"ORP故障"=FALSE, "温控器故障"=FALSE, "加热故障"=FALSE, "高锰酸钾报警"=FALSE, "草酸钠报警"=FALSE, "测量错误"=FALSE, "校零错误"=FALSE, "校标错误"=FALSE, " 进水样超量程"=FALSE, "排液阀故障"=FALSE} ("报警簇"), "ORP故障"=w1923, "温控器故障"=w1922, "加热故障"=w1921, "高锰酸钾报警"=w1920, "草酸钠报警"=w1919, "测量错误"=w1918, "校零错误"=w1917, "校标错误"=w1916, "进水样超量程"=w1915, "排液阀故障"=w1914) -> (→"报警簇":T3)
      }
    }
  }
